vi "main_scan_3.vi"() -> ()   [LabVIEW 2009]
uses:
  <vilib>/userDefined/High Color/IMAQdx.ctl
  <vilib>/vision/Image Controls.llb/IMAQ Image.ctl
  global_stage_initialised.vi
  <vilib>/vision/driver/IMAQdx.llb/IMAQdx Buffer Number Mode.ctl
  <vilib>/Utility/file.llb/Write To Spreadsheet File (DBL).vi
  <vilib>/vision/driver/NI_Vision_Acquisition_Software.lvlib
  C:/Program Files/National Instruments/LabVIEW 2009/resource/objmgr/imaqdx.rc
panel:
  out "Vektor Summierte Helligkeit [a.u.]":dbl[](array[numeric])
  out "Vektor L/2-Position [°]":dbl[](array[numeric])
  out "Daten speichern":bool
  out "Leist/Pol # Schleifen":i64
  out "Leistungs-/Polarisationscan läuft":bool
  in  "Max. Spannungsdifferenz":dbl=150.0
  out "Geschätzte Messzeit":string="00:00"
  out "Start time [ms]":timestamp
  out "2D-Intensitätsverteilung (MCP)":dbl[][](graph)
  in  "# Photosignale":i32
  in  "Achs-ID":i32
  in  "Spannungskanal":refnum<k21>
  out "x-U-Scan läuft":bool
  out "Spannungsscan läuft":bool
  out "LAPD Spannung (V)":dbl format="%#.3g"
  out "Summierte Helligkeit (a.u.)":u64
  out "# Messschritte":i32
  out "Aktueller Messschritt":i32
  in  "LAPD-Daten speichern":bool
  in  "Summierte Helligkeit speichern":bool
  in  "Einzelbilder speichern":bool
  in  "Gemittelte Bilder speichern":bool
  in  "# Bilder/Messschritt":i32=1
  in  "SN von Rotationsbühne":i32=83831982
  in  "Wellenplatte [°]":refnum<k7>(container)
  out "Wellenplatte":bool
  in  "Waveplate ON/OFF":bool
  in  "Registerkarte":T1(tab)=enum."Leistungs-/Polarisationsscan"
  out "Aktuelle xyz-Position [mm]":dbl[](array[numeric]) format="%.5g"
  in  "Rasterweite [µm]":dbl[](array[numeric])
  in  "# Rasterschritte":i32[](array[numeric])=[1, 1, 1] min=1 step=1
  in  "Rasterung ON/OFF":bool
  out "Start xyz-Position [mm]":dbl[](array[numeric]) format="%.5g"
  in  "Rasterart":T2(ring)=enum."2D-Scan(xy)"
  out "Rasterschritt [µm]":dbl[](array[numeric])
  out "2D-Intensitätsverteilung (LAPD)":dbl[][](graph)
  out "Spannungsstart [V]":dbl[](array[numeric])
  out "TIP/SUP":string[](array[string])=["Tip", "Suppressor"]
  out "Spannungsschritt [V]":dbl[](array[numeric]) format="%.1g"
  out "Aktuelle Spannung [V]":dbl[](array[numeric]) format="%.1f"
  in  "# Spannungsschritte":i32[](array[numeric])
  in  "Spannungsweite [V]":dbl[](array[numeric])
  in  "Spannungsscan ON/OFF":bool
  out "Schräglage berücksichtigen":string="Schräglage berücksichtigen"
  in  "Ausgleichslage Start festlegen":bool
  out "x-U-Scan (Ausgleichslage) xy-Start [mm]":dbl[](array[numeric]) format="%_5g"
  in  "Raum-Koordinate 2 (Lagenausgleich)":enum16{"x-Achse", "y-Achse", "z-Achse"}(ring)=enum."y-Achse"
  out "x-U-Scan y-Startposition [mm]":dbl format="%.4g"
  out "x-U-Scan aktuelle y-Position [mm]":dbl format="%.4g"
  in  "x-U-Scan (Ausgleichslage) Steigung":dbl format="%_3g"
  out "x-U-Scan Spannungsstart [V]":dbl
  out "x-U-Scan Spannungsschritt [V]":dbl
  out "x-U-Scan aktuelle Spannung [V]":dbl
  in  "# x-U-Scan Spannungsschritte":i32
  in  "x-U-Scan Spannungsweite [V]":dbl
  in  "Raum-Koordinate 1":enum16{"x-Achse", "y-Achse", "z-Achse"}(ring)
  in  "Spannungs-Koordinate":enum16{"Tip-Spannung", "Suppressor-Spannung"}(ring)=2
  in  "x-U-Scan ON/OFF":bool
  in  "x-U-Scan x-Rasterweite [µm]":dbl
  in  "# x-U-Scan x-Rasterschritte":i32
  out "x-U-Scan x-Startposition [mm]":dbl format="%.4g"
  out "x-U-Scan aktuelle x-Position [mm]":dbl format="%.4g"
  out "x-U-Scan x-Rasterschritt [µm]":dbl
  out "x-U-Scan (Ausgleichslage) xy-End [mm]":dbl[](array[numeric]) format="%_5g"
  in  "Ausgleichslage Ende festlegen":bool
  in  "Max. Leistung (vK) [mW]":dbl
  out "Aktuelle Leistung (iK) [mW]":dbl
  out "Aktuelle L/2-Position [°]":dbl format="%_3g"
  out "L/2-Schritt [°]":dbl
  in  "Hin und Zurück":bool=TRUE
  in  "# L/2-Schritte":i32
  in  "L/2-Weite [°]":dbl
  in  "L/2-Start [°]":dbl
  in  "Leistuns- oder Polarisationsscan":u16(ring) items=["Polarisationsscan", "Leistungsscan"]
  in  "Leistungs-/Polarisationsscan ON/OFF":bool
  out "1D-Intensitätsverteilung (MCP)":T3(graph)
  in  "Sequenz Ordner":string="Referenzbilder"
  in  "Sequenzaufnahme ON":bool
  in  "MCP-Spannung [V]":dbl=1400.0
  in  "P-Schirm-Spannung [V]":dbl=4400.0
  in  "Proben-ID":string="140528_06"
  out "Messlogbuch":path
  out "Gemitteltes Bild":u64[][](array[numeric])
  in  "Polarisation [°]":dbl=90.0
  out "Current y step":i32
  out "Current z step":i32
  out "Current x step":i32
  out "Scanschleifenzähler":i32
  out "Kameraschleifenzähler":i32
  out "Steuerschleifenzähler":i32
  out "Bühne":bool
  in  "HV ON/OFF":bool
  out "HV-Steuerung":bool
  in  "Suppressor-Spannung [V]":dbl min=0.0 max=1000.0 step=1.0 format="%.1p"
  in  "Tip-Spannung [V]":dbl min=0.0 max=800.0 step=1.0 format="%.1p"
  in  "Leistung (iK) [mW]":dbl format="%.1f"
  in  "LAPD-Kanal (Meilhaus)":u32=1 max=31
  out "Save folder":string
  out "Buffer Number":u64
  out "ROI table":string[](array[string])=["Breite [px]", "Höhe [px]", "X-Offset [px]", "Y-Offset [px]"]
  in  "Vollbild":bool
  out "Frame Rate (FPS)":dbl format="%#_3g"
  in  "Buffer Interval":u32=1
  out "Ereignis: FrameDone?":refnum<event-registration>
  out "Image Display":T4(plugin-control)
  in  "ROI":i32[](array[numeric])=[640, 480, 0, 0]
  in  "Shutter time (ms)":u16(ring)=3 items=["1000", "500", "200", "100", "50", "20", "10"]
  out "Buffer Overrun":bool
  out "Image Memory":T4
  out "Kamera":bool
  in  "Kamera ON/OFF":bool
  in  "Detektionskamera":T5="cam0"
  out "Day folder":string
  in  "Root folder":string="E:\\GIPES\\Messungen\\"
  out "z-Achse":i32=3
  out "y-Achse":i32=2
  out "x-Achse":i32=1
  out "Event: Rasterung gestartet?":refnum<user-event>
  out "Fehler (Ausgang)":errorcluster
  in  "Programm beenden":bool
  out "Rasterung läuft":bool
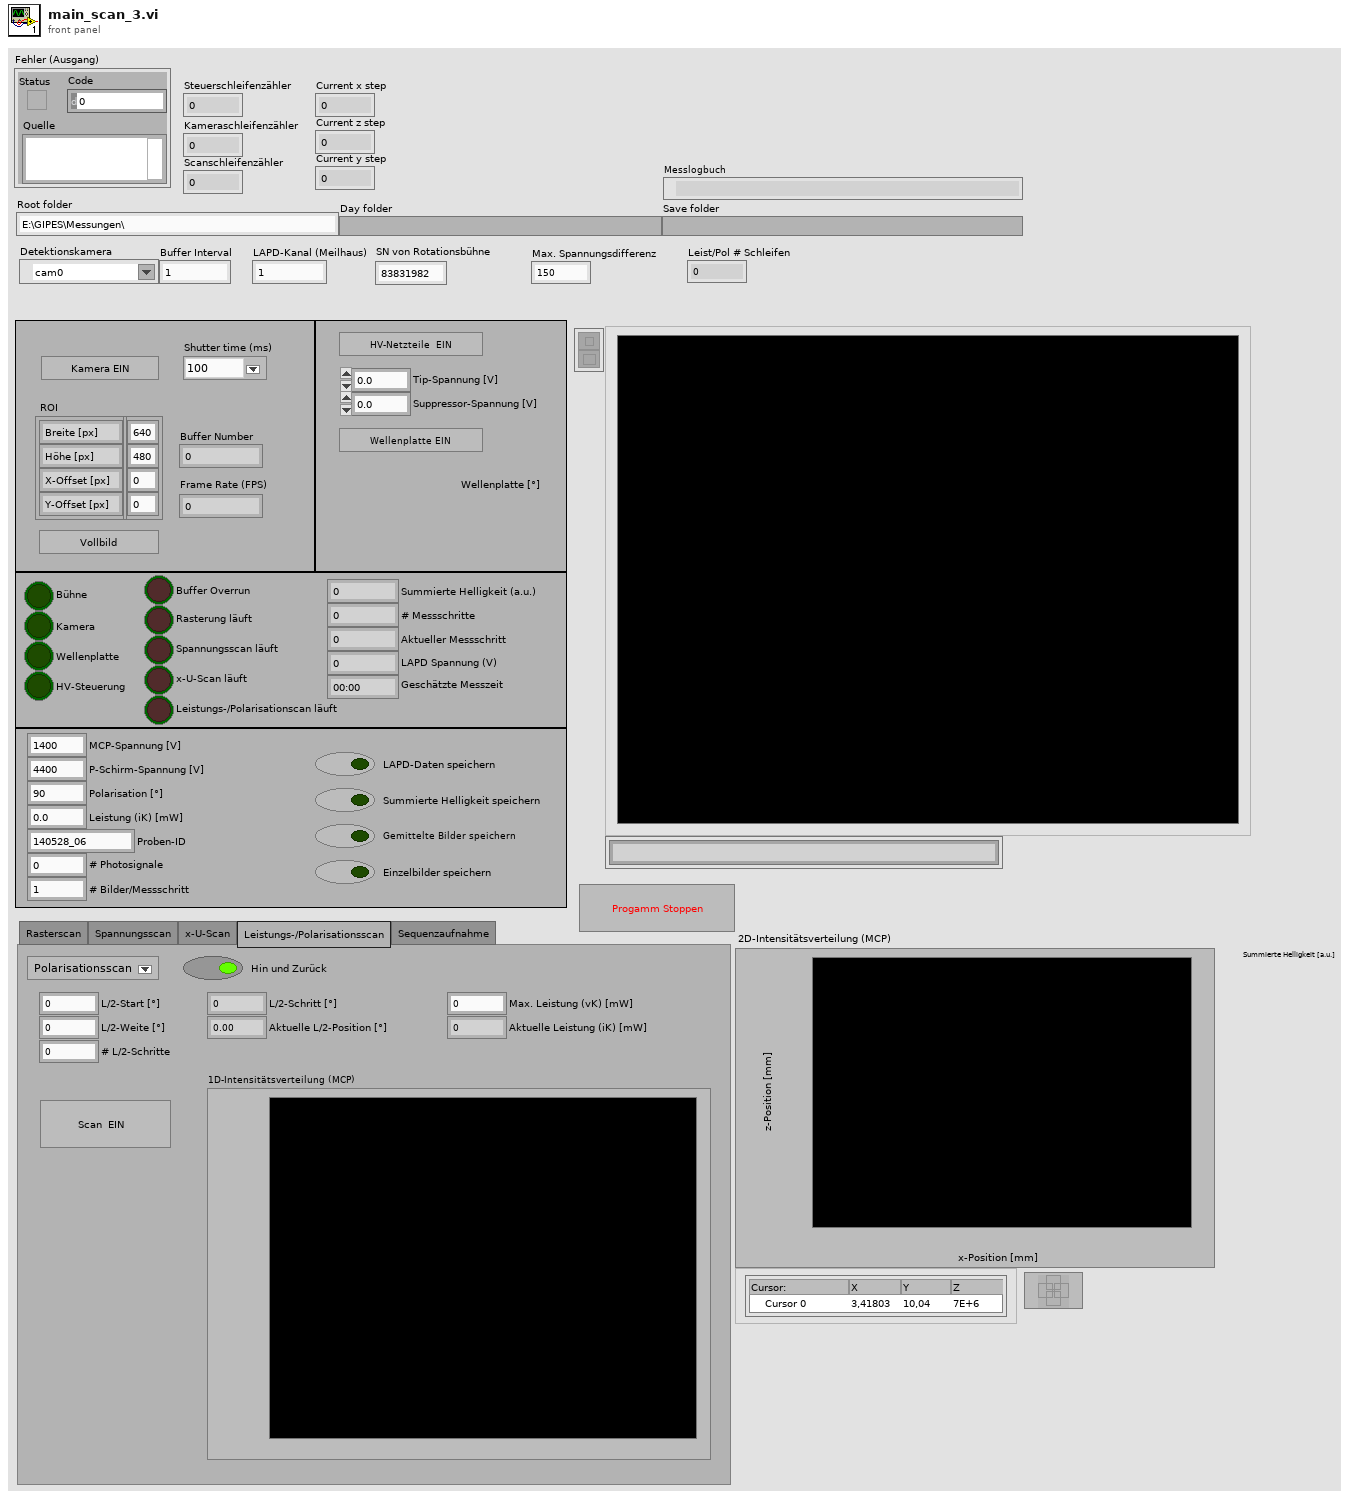
[diagram p1: front panel]
types:
  T1 = enum32{"Rasterscan", "Spannungsscan", "x-U-Scan", "Leistungs-/Polarisationsscan", "Sequenzaufnahme"}
  T2 = enum16{"Linescan(x)", "Linescan(z)", "2D-Scan(xy)", "2D-Scan(yz)", "2D-Scan(xz)"}
  T3 = cluster{"Vektor L/2-Position [°]":dbl[], "Vektor Summierte Helligkeit [a.u.]":dbl[]}
  T4 = typedef "IMAQ Image.ctl" = refnum<image>
  T5 = typedef "IMAQdx.ctl" = refnum<k21>
  T6 = enum32{"Bad", "Idle", "Run top level", "Running"}
  T7 = cluster{"Summierte Helligkeit (a.u.)":u64, "Aktuelle L/2-Position [°]":dbl}
  T8 = typedef "NI_Vision_Acquisition_Software.lvlib/IMAQdx Buffer Number Mode.ctl" = enum32{"Next", "Last", "Buffer Number"}
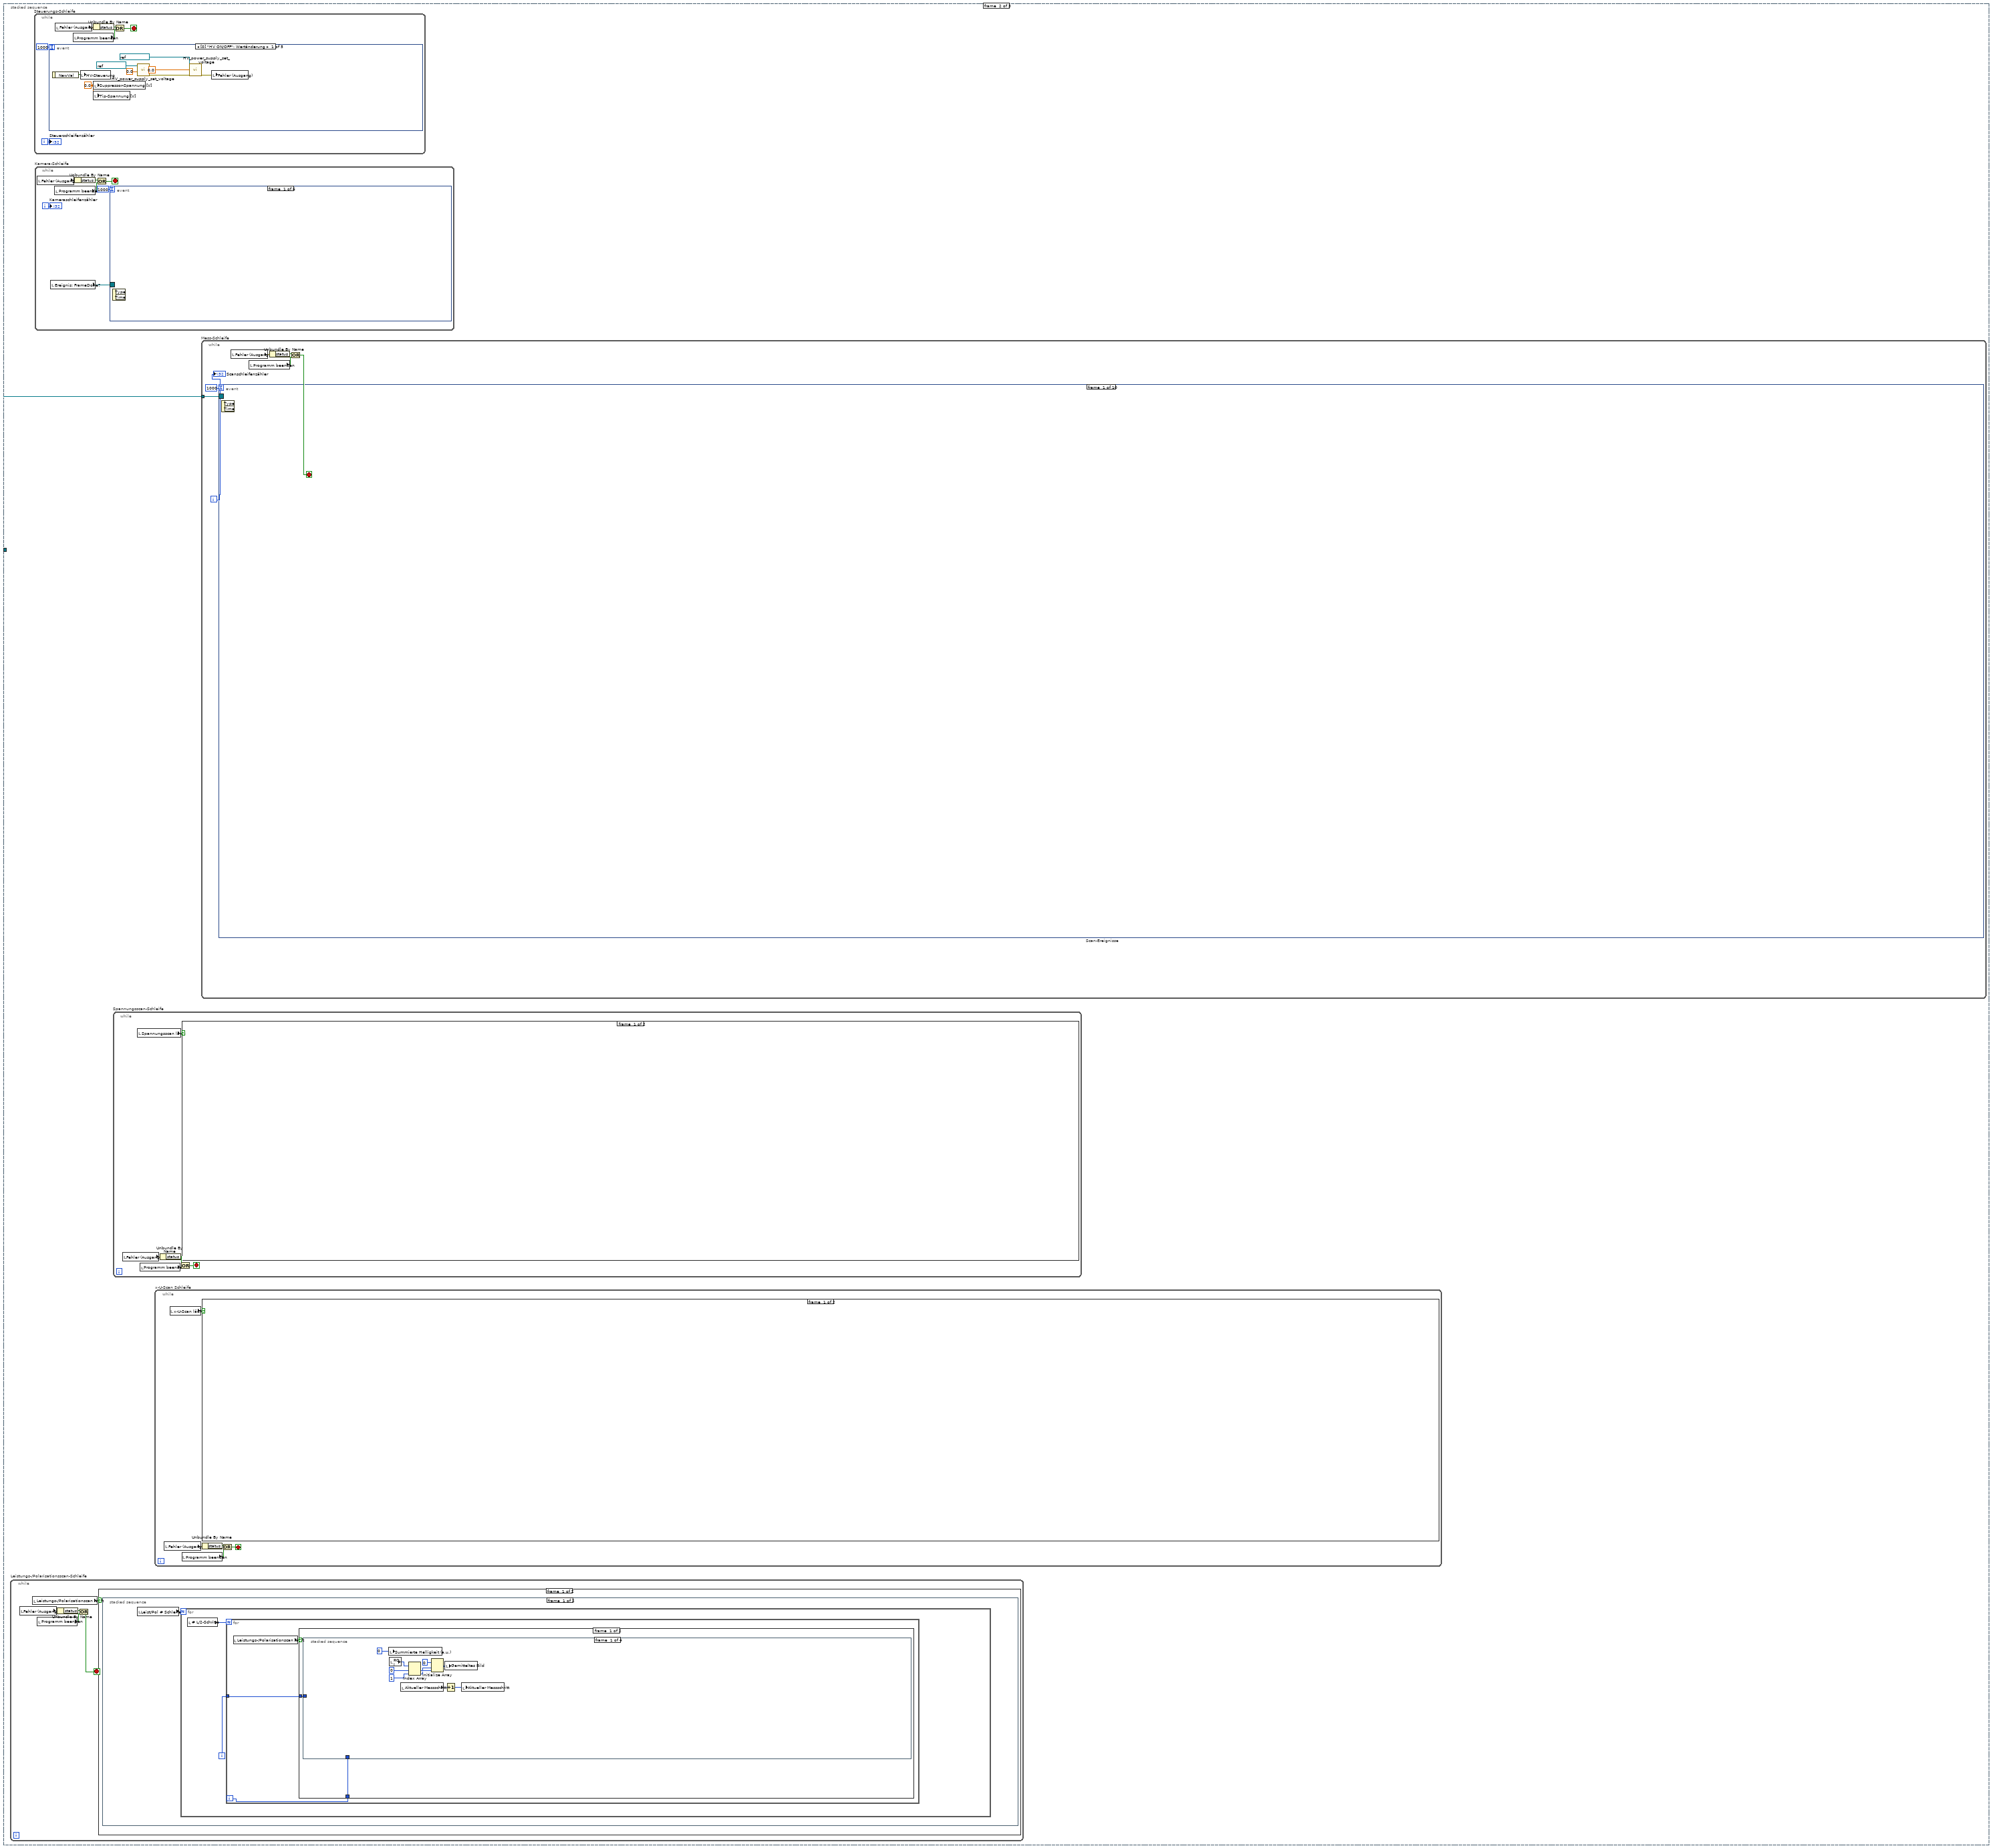
[diagram p3: hidden frame]
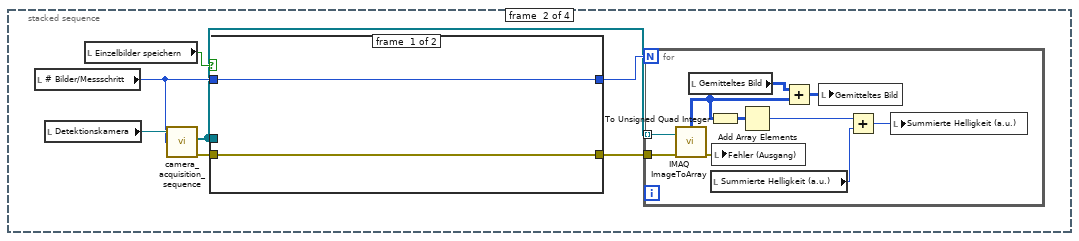
[diagram p4: hidden frame]
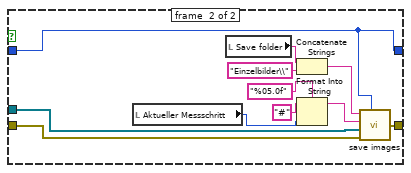
[diagram p5: hidden frame]
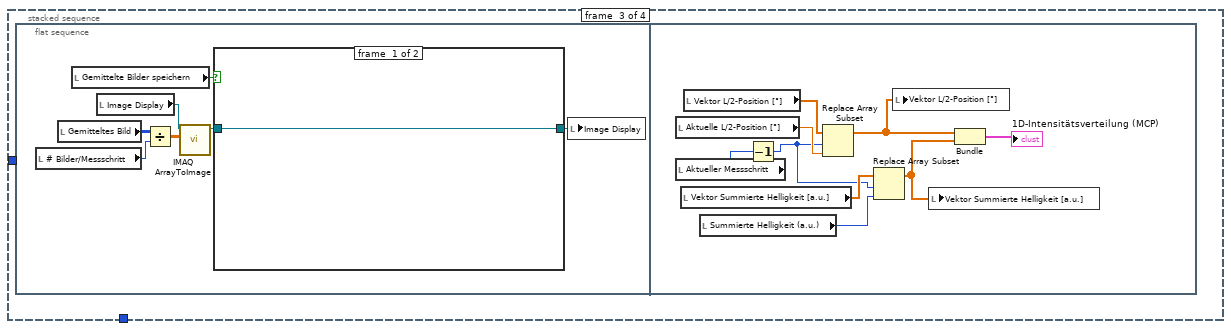
[diagram p6: hidden frame]
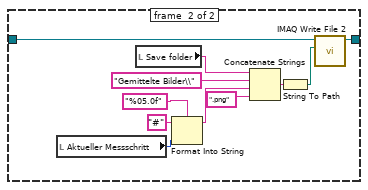
[diagram p7: hidden frame]
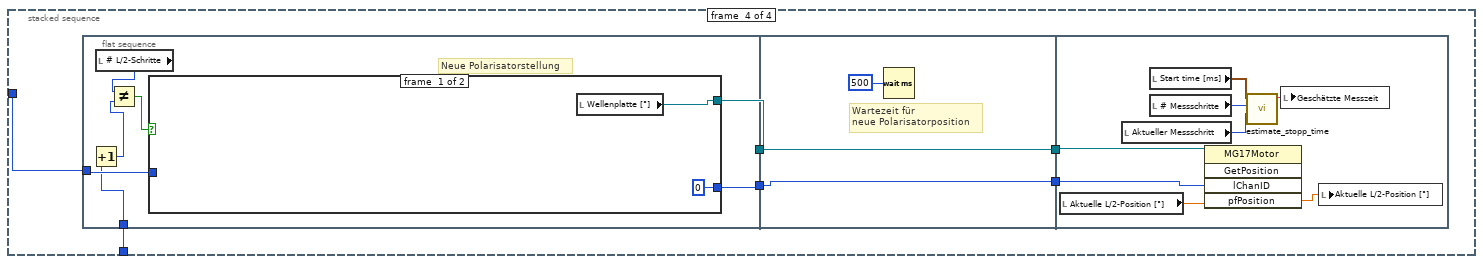
[diagram p8: hidden frame]
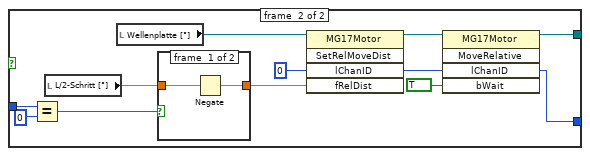
[diagram p9: hidden frame]
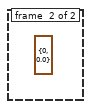
[diagram p11: hidden frame]
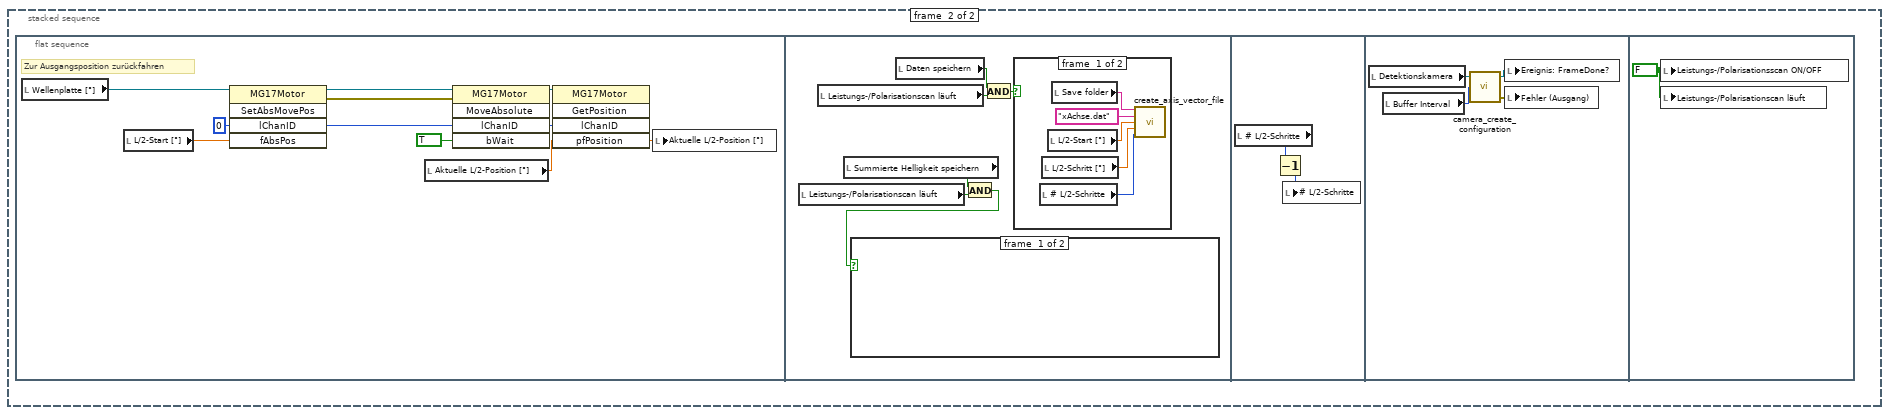
[diagram p12: hidden frame]
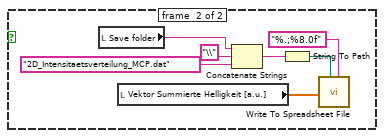
[diagram p13: hidden frame]
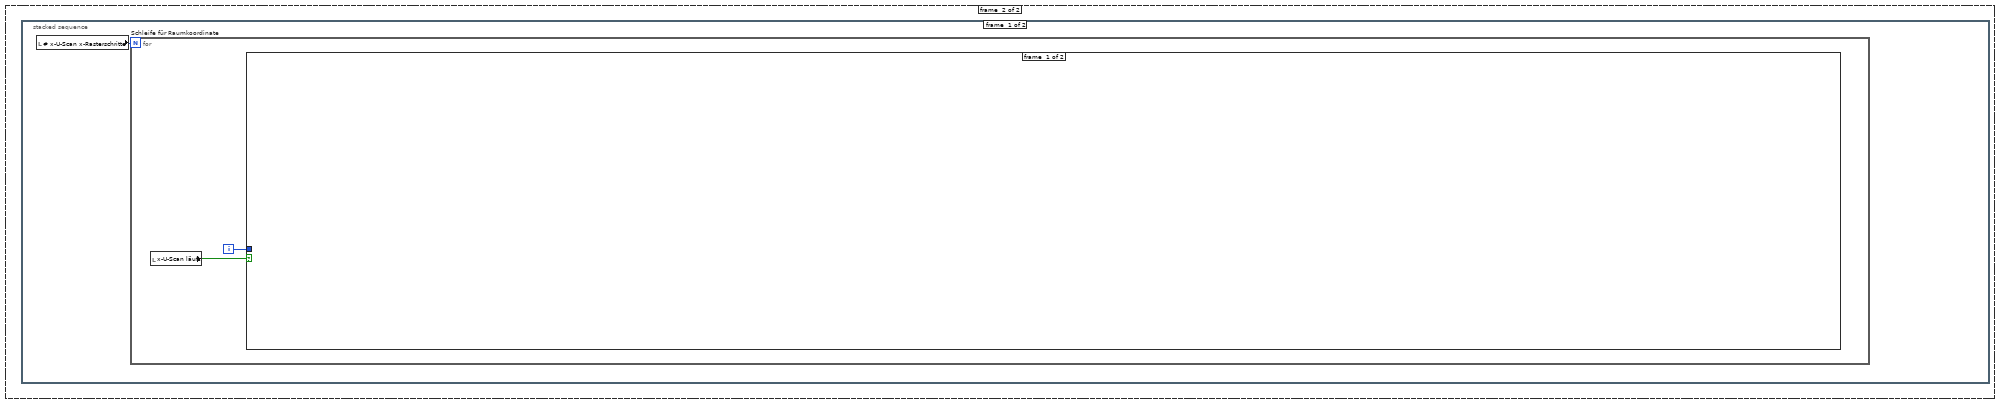
[diagram p16: hidden frame]
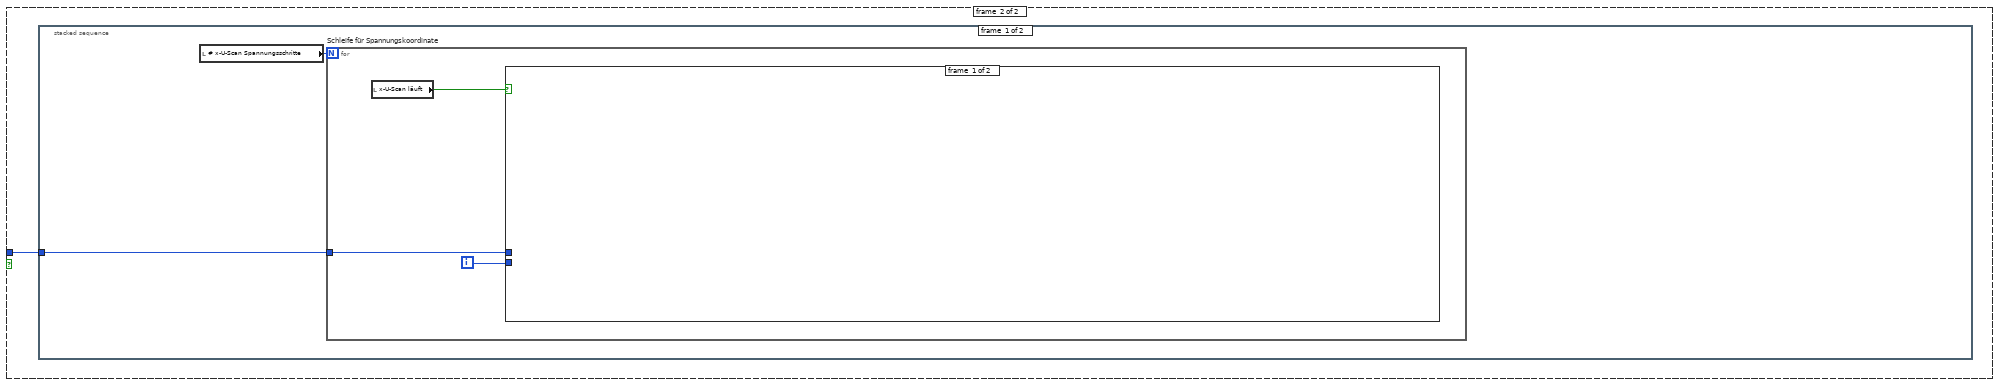
[diagram p17: hidden frame]
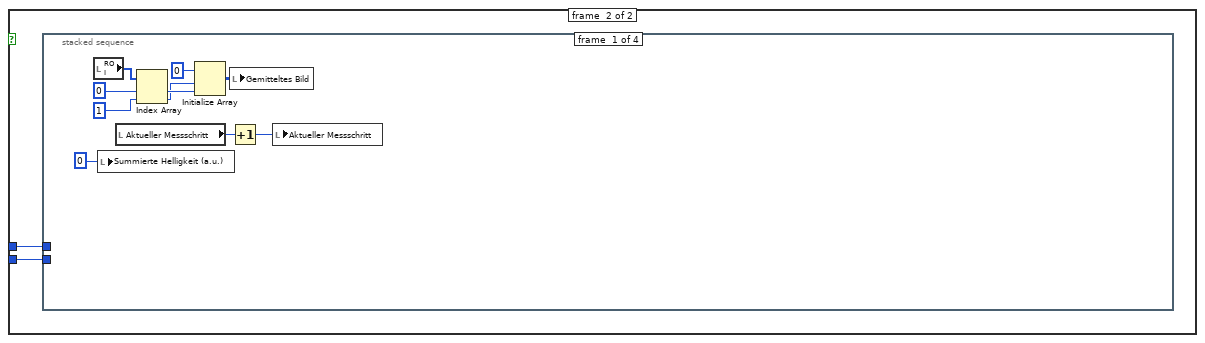
[diagram p18: hidden frame]
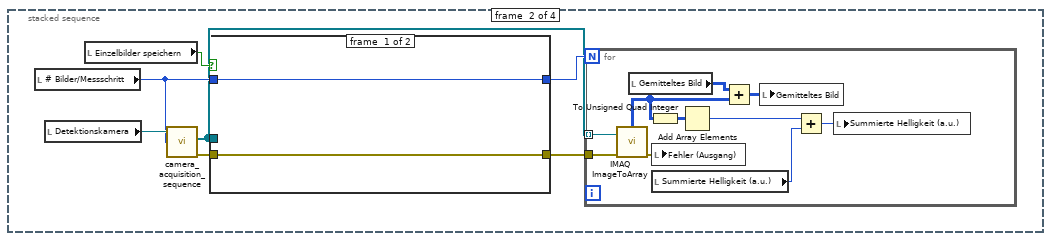
[diagram p19: hidden frame]
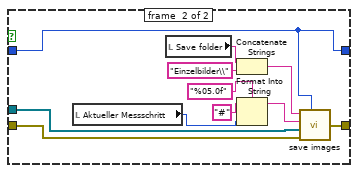
[diagram p20: hidden frame]
diagram:
  n1 = local read "Event: Rasterung gestartet?"() -> (w2:refnum<user-event>)
  n2 = register-events(w2) -> (reference out=w1:refnum<event-registration>)  [unwired: 2 in, 1 out]
  n3 = flat-sequence {
    frame #0 {
      w5 = 0.0 ("Aktuelle x-Position [mm]")
      w11 = 1 ("# x-U-Scan Spannungsschritte")
      w12 = 0.0 ("Aktuelle x-Position [mm]")
      w10 = 0.0 ("Suppressor-Spannung [V]")
      w25 = u16 3 items=["1000", "500", "200", "100", "50", "20", "10"] ("Shutter time (ms)")
      w3 = FALSE ("Scanstart")
      n4 = Initialize Array(1 ("Element"), 2 ("Dimension")) -> (w13:i32[])
      n5 = Initialize Array(1 ("Dimension"), 3 ("Dimension")) -> (w37:i32[])
      n6 = Initialize Array(0.0 ("Element"), 2 ("Dimension")) -> (w9:dbl[])
      "Aktuelle Spannung [V]" <- w9
      "Spannungsstart [V]" <- w9
      "x-U-Scan (Ausgleichslage) xy-Start [mm]" <- w9
      "x-U-Scan (Ausgleichslage) xy-End [mm]" <- w9
      n7 = Initialize Array(0.0 ("Element"), 3 ("Dimension")) -> (w19:dbl[])
      "Aktuelle xyz-Position [mm]" <- w19
      "Start xyz-Position [mm]" <- w19
      "Rasterschritt [µm]" <- w19
      n8 = local write "Tip-Spannung [V]"(0.0 ("Tip-Spannung [V]")) -> ()
      n9 = local write "# Photosignale"(10.0 ("Anzahl Mittelungen")) -> ()
      n10 = local write "# x-U-Scan x-Rasterschritte"(w11) -> ()
      n11 = local write "x-U-Scan x-Rasterweite [µm]"(w10) -> ()
      n12 = local write "Shutter time (ms)"(w25) -> ()
      n13 = local write "# Spannungsschritte"(w13) -> ()
      n14 = local write "ROI"(i32[] [640, 480, 0, 0] ("Region of Interest (px)")) -> ()
      n15 = local write "# x-U-Scan Spannungsschritte"(w11) -> ()
      n16 = local write "x-U-Scan Spannungsweite [V]"(w10) -> ()
      n17 = local write "Suppressor-Spannung [V]"(w10) -> ()
      n18 = local read "Aktueller Messschritt"() -> (w30:i32)
      n19 = local write "# Rasterschritte"(w37) -> ()
      n20 = local write "Spannungsweite [V]"(w9) -> ()
      n21 = local write "Rasterweite [µm]"(w19) -> ()
      n22 = local write "x-U-Scan (Ausgleichslage) Steigung"(0.0 ("x-U-Scan (Ausgleichslage) Steigung")) -> ()
      n23 = local write "HV ON/OFF"(w3) -> ()
      n24 = local write "Spannungsscan ON/OFF"(w3) -> ()
      n25 = local write "Buffer Overrun"(w3) -> ()
      n26 = local write "Programm beenden"(w3) -> ()
      n27 = local write "x-U-Scan ON/OFF"(w3) -> ()
      n28 = local write "x-U-Scan läuft"(w3) -> ()
      n29 = local write "Sequenzaufnahme ON"(w3) -> ()
      n30 = local write "Kamera ON/OFF"(w3) -> ()
      n31 = local write "Rasterung ON/OFF"(w3) -> ()
      n32 = local write "Rasterung läuft"(w3) -> ()
      n33 = local write "Spannungsscan ON/OFF"(w3) -> ()
      n34 = local write "Waveplate ON/OFF"(w3) -> ()
      n35 = Create User Event(user event datatype=w30) -> (user event=→"Event: Rasterung gestartet?":refnum<user-event>)  [unwired: 1 in, 1 out]
      n36 = local write "Leistungs-/Polarisationsscan ON/OFF"(w3) -> ()
      "Rasterung läuft" <- FALSE ("Scan aktiv")
      "# Messschritte" <- 0 ("# Messschritte")
      "Aktueller Messschritt" <- 0 ("Aktueller Messschritt")
      "x-Achse" <- 1 ("x-Achse")
      "y-Achse" <- 2 ("y-Achse")
      "z-Achse" <- 3 ("z-Achse")
      "Summierte Helligkeit (a.u.)" <- i64 0 ("Numerisches Element")
      "LAPD Spannung (V)" <- 0.0 ("Transmittierte Intensität (a.u.)")
      "Bühne" <- w3
      "Wellenplatte" <- w3
      "Kamera" <- FALSE ("Camera eingeschaltet")
      "HV-Steuerung" <- w3
      "Spannungsscan läuft" <- w3
      "x-U-Scan aktuelle x-Position [mm]" <- w12
      "x-U-Scan x-Rasterschritt [µm]" <- w12
      "x-U-Scan aktuelle Spannung [V]" <- w12
      "x-U-Scan Spannungsschritt [V]" <- w12
      "x-U-Scan x-Startposition [mm]" <- w12
      "x-U-Scan Spannungsstart [V]" <- w10
      "x-U-Scan aktuelle y-Position [mm]" <- 0.0 ("x-U-Scan aktuelle y-Position [mm]")
      "x-U-Scan y-Startposition [mm]" <- 0.0 ("x-U-Scan y-Startposition [mm]")
      "L/2-Schritt [°]" <- w5
      "Aktuelle L/2-Position [°]" <- w5
      "Aktuelle Leistung (iK) [mW]" <- w5
      "Leistungs-/Polarisationscan läuft" <- w3
      "Leist/Pol # Schleifen" <- i64 1 ("Leist/Pol # Schleifen")
      "Daten speichern" <- w3
    }
  }
  n37 = stacked-sequence {
    tunnel: w1 -> [_ w63 _]
    frame #0 {
      n38 = flat-sequence {
        frame #0 {
          # "Überprüfung ob die VI stage_control.vi ausgeführt wid, wenn nicht wird sie gestartet und gewartet bis die Bühne initialisiert ist"
          n39 = Open VI Reference(vi path=path "stage_control.vi" ("VI-Pfad")) -> (vi reference=w41:refnum<vi>)  [unwired: 5 in, 1 out]
          n40 = property class="VI"(reference=w41) -> (reference out=w40:refnum<vi>, error out=w39:errorcluster, "Exec.State"=w44:T6)  [unwired: 1 in]
          n41 = Equal?(x=w44, y=T6."Run top level") -> (x = y?=w42:bool)
          n42 = case shown="False" w42 {
            tunnel: w40 -> [w51 _]
            tunnel: w39 -> [w50 _]
            frame #0 {
              n43 = invoke class="VI" method="VI ausführen"(reference=w51, error in=w50, "Wait until done"=FALSE ("Warten bis beendet"), "Auto Dispose Ref"=FALSE ("Referenz automatisch schließen")) -> (reference out=w47:refnum<vi>)  [unwired: 1 in, 4 out]
              n44 = invoke class="VI" method="FP.Öffnen"(reference=w47) -> (reference out=w46:refnum<vi>)  [unwired: 4 in, 4 out]
              n45 = while {
                tunnel: w46 -> [w58]
                stop <- w53 stop-if-true
                n46 = property class="VI"(reference=w58) -> (error out=w57:errorcluster, "Exec.State"=w56:T6)  [unwired: 1 in, 1 out]
                n47 = global read "global_stage_initialised.vi" "Bühne initialisiert"() -> (w52:bool)
                n48 = local write "Fehler (Ausgang)"(w57) -> ()
                n49 = Equal?(x=w56, y=T6."Run top level") -> (x = y?=w54:bool)
                n50 = And(x=w52, y=w54) -> (x .and. y?=w53:bool)
              }
            }
            frame #1 {
            }
          }
        }
        frame #1 {
          n51 = local read "Root folder"() -> (w62:string)
          n52 = local write "Bühne"(TRUE ("Bühne bereit")) -> ()
          n53 = call "create_day_folder.vi"("Root folder"=w62) -> ("Day Folder"=w60:string)  [unwired: 9 in, 1 out]
          n54 = local write "Day folder"(w60) -> ()
          n55 = call "create_measure_log_file.vi"("Tagesordner"=w60) -> ("Messlogbuch"=w59:path)  [unwired: 9 in]
          n56 = local write "Messlogbuch"(w59) -> ()
        }
      }
    }
    frame #1 {
      n57 = while "Leistungs-/Polarisationsscan-Schleife" {
        stop <- w65 stop-if-true
        n58 = local read "Fehler (Ausgang)"() -> (w68:errorcluster)
        n59 = local read "Leistungs-/Polarisationscan läuft"() -> (w64:bool)
        n60 = local read "Programm beenden"() -> (w66:bool)
        n61 = Unbundle By Name(w68) -> ("status"=w67:bool)
        n62 = Or(x=w67, y=w66) -> (x .or. y?=w65:bool)
        n63 = case shown="True" w64 {
          frame #0 {
            n64 = stacked-sequence {
              frame #0 {
                n65 = local read "Leist/Pol # Schleifen"() -> (w69:i64)
                n66 = for {
                  N: w69 -> [_]
                  i -> [w70]
                  n67 = local read "# L/2-Schritte"() -> (w71:i32)
                  n68 = for "Schleife für L/2-Position" {
                    N: w71 -> [_]
                    tunnel: w70 -> [w73]
                    i -> [w72]
                    n69 = local read "Leistungs-/Polarisationscan läuft"() -> (w74:bool)
                    n70 = case shown="True" w74 {
                      tunnel: w73 -> [w76 _]
                      tunnel: w72 -> [w75 _]
                      frame #0 {
                        n71 = stacked-sequence {
                          tunnel: w76 -> [_ _ _ w150]
                          tunnel: w75 -> [_ _ _ w145]
                          frame #0 {
                            n72 = local write "Summierte Helligkeit (a.u.)"(u64 0 ("Summierte Helligkeit (a.u.)")) -> ()
                            n73 = local read "ROI"() -> (w82:i32[])
                            n74 = local read "Aktueller Messschritt"() -> (w79:i32)
                            n75 = Index Array(array=w82, index #1=0 ("Index"), index #2=1 ("Index")) -> (element #1=w86:i32, element #2=w85:i32)
                            n76 = Initialize Array(u64 0 ("Element"), w85, w86) -> (w80:u64[][])
                            n77 = local write "Gemitteltes Bild"(w80) -> ()
                            n78 = Increment(x=w79) -> (x+1=w78:i32)
                            n79 = local write "Aktueller Messschritt"(w78) -> ()
                          }
                          frame #1 {
                            n80 = local read "# Bilder/Messschritt"() -> (w90:i32)
                            n81 = local read "Detektionskamera"() -> (w93:T5)
                            n82 = local read "Einzelbilder speichern"() -> (w88:bool)
                            n83 = call "camera_acquisition_sequence.vi"("Session In"=w93, "Desired image number"=w90) -> ("Image Array"=w87:T4[], "error out"=w92:errorcluster)  [unwired: 2 in, 1 out]
                            n84 = case shown="True" w88 {
                              tunnel: w92 -> [w95 w103]
                              tunnel: [w95 w102] -> w91
                              tunnel: w90 -> [w94 w101]
                              tunnel: [w94 w101] -> w89
                              tunnel: w87 -> [_ w100]
                              frame #0 {
                              }
                              frame #1 {
                                n85 = local read "Aktueller Messschritt"() -> (w106:i32)
                                n86 = local read "Save folder"() -> (w98:string)
                                n87 = Concatenate Strings(w98, "Einzelbilder\\" ("String")) -> (w96:string)
                                n88 = Format Into String(format string="%05.0f" ("Format-String"), initial string="#" ("Eingangs-String"), w106) -> (resulting string=w99:string)  [unwired: 1 in, 1 out]
                                n89 = call "save images.vi"("Save Folder"=w96, "File name prefix"=w99, "Array"=w100, "error out 2"=w103, "Bilder/Messschritt"=w101) -> ("error out"=w102:errorcluster)
                              }
                            }
                            n90 = for {
                              N: w89 -> [_]
                              tunnel: w91 -> [w112]
                              tunnel: w87 -> [w110] mode=indexing
                              n91 = call "IMAQ ImageToArray"("error in (no error)"=w112, "Image"=w110) -> ("error out"=w111:errorcluster, "Image Pixels (U8)"=w109:u8[][])  [unwired: 2 in, 3 out]
                              n92 = local read "Gemitteltes Bild"() -> (w107:u64[][])
                              n93 = To Unsigned Quad Integer(1:w109) -> (0:w114:u64[][])
                              n94 = local read "Summierte Helligkeit (a.u.)"() -> (w115:u64)
                              n95 = local write "Fehler (Ausgang)"(w111) -> ()
                              n96 = Add Array Elements(numeric array=w114) -> (sum=w113:u64)
                              n97 = Add(x=w107, y=w109) -> (x+y=w108:u64[][])
                              n98 = local write "Gemitteltes Bild"(w108) -> ()
                              n99 = Add(x=w113, y=w115) -> (x+y=w116:u64)
                              n100 = local write "Summierte Helligkeit (a.u.)"(w116) -> ()
                            }
                          }
                          frame #2 {
                            n101 = flat-sequence {
                              frame #0 {
                                n102 = local read "# Bilder/Messschritt"() -> (w119:i32)
                                n103 = local read "Gemitteltes Bild"() -> (w117:u64[][])
                                n104 = local read "Gemittelte Bilder speichern"() -> (w123:bool)
                                n105 = local read "Image Display"() -> (w121:T4)
                                n106 = Divide(x=w117, y=w119) -> (x/y=w118:dbl[][])
                                n107 = call "IMAQ ArrayToImage"("Image Pixels (U8)"=w118, "Image"=w121) -> ("Image Out"=w120:T4)  [unwired: 8 in, 1 out]
                                n108 = case shown="True" w123 {
                                tunnel: w120 -> [w124 w135]
                                tunnel: [w124 w126] -> w122
                                frame #0 {
                                }
                                frame #1 {
                                n109 = local read "Aktueller Messschritt"() -> (w130:i32)
                                n110 = local read "Save folder"() -> (w132:string)
                                n111 = Format Into String(format string="%05.0f" ("Format-String"), initial string="#" ("Eingangs-String"), w130) -> (resulting string=w129:string)  [unwired: 1 in, 1 out]
                                n112 = Concatenate Strings(w132, "Gemittelte Bilder\\" ("String"), w129, ".png" ("String")) -> (w128:string)
                                n113 = String To Path(string=w128) -> (path=w127:path)
                                n114 = call-poly "IMAQ Write File 2"("File Path"=w127, "Image"=w135) -> ("Image Out (duplicate)"=w126:T4)  [unwired: 8 in, 1 out]
                                }
                                }
                                n115 = local write "Image Display"(w122) -> ()
                              }
                              frame #1 {
                                n116 = local read "Aktuelle L/2-Position [°]"() -> (w141:dbl)
                                n117 = local read "Aktueller Messschritt"() -> (w139:i32)
                                n118 = local read "Vektor Summierte Helligkeit [a.u.]"() -> (w143:dbl[])
                                n119 = local read "Vektor L/2-Position [°]"() -> (w142:dbl[])
                                n120 = local read "Summierte Helligkeit (a.u.)"() -> (w140:u64)
                                n121 = Decrement(x=w139) -> (x-1=w138:i32)
                                n122 = Replace Array Subset(array=w142, new element=w141, index=w138) -> (w137:dbl[])
                                n123 = Replace Array Subset(array=w143, new element=w140, index=w138) -> (w136:dbl[])
                                n124 = local write "Vektor L/2-Position [°]"(w137) -> ()
                                n125 = local write "Vektor Summierte Helligkeit [a.u.]"(w136) -> ()
                                n126 = Bundle("Vektor L/2-Position [°]"=w137, "Vektor Summierte Helligkeit [a.u.]"=w136) -> (→"1D-Intensitätsverteilung (MCP)":T3)  [unwired: 1 in]
                              }
                            }
                          }
                          frame #3 {
                            n127 = flat-sequence {
                              tunnel: w150 -> [w157]
                              tunnel: [w156] -> w149
                              tunnel: [w155] -> w148
                              tunnel: w145 -> [w154]
                              tunnel: w149 -> [w175]
                              tunnel: w148 -> [w176]
                              tunnel: [w176] -> w147
                              tunnel: [w175] -> w146
                              tunnel: w147 -> [w181]
                              tunnel: w146 -> [w180]
                              frame #0 {
                                # "Neue Polarisatorstellung"
                                n128 = Increment(x=w154) -> (x+1=w153:i32)
                                n129 = local read "# L/2-Schritte"() -> (w152:i32)
                                n130 = Not Equal?(x=w152, y=w153) -> (x != y?=w151:bool)
                                n131 = case shown="True" w151 {
                                tunnel: w157 -> [_ w164]
                                tunnel: [0 ("lChanID") w161] -> w156
                                tunnel: [w159 w160] -> w155
                                frame #0 {
                                n132 = local read "Wellenplatte [°]"() -> (w159:refnum<k7>)
                                }
                                frame #1 {
                                n133 = Equal?(x=w164, y=0) -> (x = y?=w162:bool)
                                n134 = local read "L/2-Schritt [°]"() -> (w166:dbl)
                                n135 = local read "Wellenplatte [°]"() -> (w167:refnum<k7>)
                                n136 = case shown="False" w162 {
                                tunnel: w166 -> [w173 w174]
                                tunnel: [w172 w174] -> w165
                                frame #0 {
                                n137 = Negate(x=w173) -> (-x=w172:dbl)
                                }
                                frame #1 {
                                }
                                }
                                n138 = invoke class="MG17Motor" method="SetRelMoveDist"(reference=w167, "lChanID"=0, "fRelDist"=w165) -> (reference out=w169:refnum<k7>, "lChanID"=w170:i32)  [unwired: 2 in, 3 out]
                                n139 = invoke class="MG17Motor" method="MoveRelative"(reference=w169, "lChanID"=w170, "bWait"=TRUE) -> (reference out=w160:refnum<k7>, "lChanID"=w161:i32)  [unwired: 2 in, 3 out]
                                }
                                }
                              }
                              frame #1 {
                                # "Wartezeit für\nneue Polarisatorposition"
                                n140 = Wait (ms)(milliseconds to wait=u32 500 ("Zu wartende ms")) -> ()  [unwired: 1 out]
                              }
                              frame #2 {
                                n141 = local read "Aktuelle L/2-Position [°]"() -> (w178:dbl)
                                n142 = local read "Aktueller Messschritt"() -> (w183:i32)
                                n143 = local read "Start time [ms]"() -> (w185:timestamp)
                                n144 = local read "# Messschritte"() -> (w184:i32)
                                n145 = invoke class="MG17Motor" method="GetPosition"(reference=w181, "lChanID"=w180, "pfPosition"=w178) -> ("pfPosition"=w179:sgl)  [unwired: 2 in, 4 out]
                                n146 = call "estimate_stopp_time.vi"("Aktueller Messschritt"=w183, "# Messschritte"=w184, "Startzeit"=w185) -> ("Stopp Zeit"=w182:string)  [unwired: 8 in]
                                n147 = local write "Geschätzte Messzeit"(w182) -> ()
                                n148 = local write "Aktuelle L/2-Position [°]"(w179) -> ()
                              }
                            }
                          }
                        }
                      }
                      frame #1 {
                        (unwired) T7 {"Summierte Helligkeit (a.u.)"=0, "Aktuelle L/2-Position [°]"=0.0}
                      }
                    }
                  }
                }
              }
              frame #1 {
                n149 = flat-sequence {
                  frame #0 {
                    # "Zur Ausgangsposition zurückfahren"
                    n150 = local read "Wellenplatte [°]"() -> (w196:refnum<k7>)
                    n151 = local read "L/2-Start [°]"() -> (w190:dbl)
                    n152 = invoke class="MG17Motor" method="SetAbsMovePos"(reference=w196, "lChanID"=0, "fAbsPos"=w190) -> (reference out=w194:refnum<k7>, error out=w191:errorcluster, "lChanID"=w192:i32)  [unwired: 2 in, 2 out]
                    n153 = local read "Aktuelle L/2-Position [°]"() -> (w188:dbl)
                    n154 = invoke class="MG17Motor" method="MoveAbsolute"(reference=w194, error in=w191, "lChanID"=w192, "bWait"=TRUE) -> (reference out=w187:refnum<k7>, "lChanID"=w186:i32)  [unwired: 1 in, 3 out]
                    n155 = invoke class="MG17Motor" method="GetPosition"(reference=w187, "lChanID"=w186, "pfPosition"=w188) -> ("pfPosition"=w189:sgl)  [unwired: 2 in, 4 out]
                    n156 = local write "Aktuelle L/2-Position [°]"(w189) -> ()
                  }
                  frame #1 {
                    n157 = local read "Leistungs-/Polarisationscan läuft"() -> (w199:bool)
                    n158 = local read "Leistungs-/Polarisationscan läuft"() -> (w201:bool)
                    n159 = local read "Summierte Helligkeit speichern"() -> (w198:bool)
                    n160 = local read "Daten speichern"() -> (w202:bool)
                    n161 = And(x=w198, y=w199) -> (x .and. y?=w197:bool)
                    n162 = case shown="True" w197 {
                      frame #0 {
                      }
                      frame #1 {
                        n163 = local read "Save folder"() -> (w203:string)
                        n164 = local read "Vektor Summierte Helligkeit [a.u.]"() -> (w204:dbl[])
                        n165 = Concatenate Strings(w203, "\\" ("String"), "2D_Intensitaetsverteilung_MCP.dat" ("String")) -> (w208:string)
                        n166 = String To Path(string=w208) -> (path=w207:path)
                        n167 = call-poly <vilib>:"Write To Spreadsheet File.vi"("format (%.3f)"="%.;%8.0f", "1D data"=w204, "file path (dialog if empty)"=w207) -> ()  [unwired: 5 in, 1 out]
                      }
                    }
                    n168 = And(x=w202, y=w201) -> (x .and. y?=w200:bool)
                    n169 = case shown="True" w200 {
                      frame #0 {
                        n170 = local read "# L/2-Schritte"() -> (w212:i32)
                        n171 = local read "L/2-Schritt [°]"() -> (w211:dbl)
                        n172 = local read "L/2-Start [°]"() -> (w210:dbl)
                        n173 = local read "Save folder"() -> (w213:string)
                        n174 = call "create_axis_vector_file.vi"("Save folder"=w213, "Dateiname"="xAchse.dat", "Start"=w210, "Schrittlänge"=w211, "# Schritte"=w212) -> ()  [unwired: 11 in]
                      }
                      frame #1 {
                      }
                    }
                  }
                  frame #2 {
                    n175 = local read "# L/2-Schritte"() -> (w216:i32)
                    n176 = Decrement(x=w216) -> (x-1=w215:i32)
                    n177 = local write "# L/2-Schritte"(w215) -> ()
                  }
                  frame #3 {
                    n178 = local read "Detektionskamera"() -> (w218:T5)
                    n179 = local read "Buffer Interval"() -> (w219:u32)
                    n180 = call "camera_create_configuration.vi"("BufferInterval"=w219, "Session Out 2"=w218) -> ("Fehler (Ausgang)"=w220:errorcluster, "Ereignisregistrierung (Referenz)"=w217:refnum<event-registration>)  [unwired: 1 in, 1 out]
                    n181 = local write "Ereignis: FrameDone?"(w217) -> ()
                    n182 = local write "Fehler (Ausgang)"(w220) -> ()
                  }
                  frame #4 {
                    w221 = FALSE ("Spannungsscan läuft")
                    n183 = local write "Leistungs-/Polarisationsscan ON/OFF"(w221) -> ()
                    n184 = local write "Leistungs-/Polarisationscan läuft"(w221) -> ()
                  }
                }
              }
            }
          }
          frame #1 {
          }
        }
      }
      n185 = while "Steuerungs-Schleife" {
        i -> [w578]
        stop <- w577 stop-if-true
        n186 = event shown="[0] \"HV ON/OFF\": Wertänderung" {
          selector: _ -> [_ _ _ _ _]
          dyn-events: _ -> [_ _ _ _ _]
          timeout: 1000 -> [_ _ _ _ _]
          event #0 {
            w583 = 0.0 ("Suppressor-Spannung [V]")
            n187 = event-data() -> ("NewVal"=w584:bool)  [unwired: 1 in]
            n188 = local write "HV-Steuerung"(w584) -> ()
            n189 = local write "Suppressor-Spannung [V]"(w583) -> ()
            n190 = local write "Tip-Spannung [V]"(w583) -> ()
            n191 = call "HV_power_supply_set_voltage.vi"("Desired output voltage in V (HV power supply)"=0.0, "Channel of HV power supply"=refnum<k21> "Dev0/Ao0") -> ("error out"=w586:errorcluster)  [unwired: 8 in]
            n192 = call "HV_power_supply_set_voltage.vi"("error in"=w586, "Desired output voltage in V (HV power supply)"=0.0, "Channel of HV power supply"=refnum<k21> "Dev0/Ao1") -> ("error out"=w585:errorcluster)  [unwired: 7 in]
            n193 = local write "Fehler (Ausgang)"(w585) -> ()
          }
          event #1 {
            n194 = event-data() -> ("NewVal"=w591:bool)  [unwired: 1 in]
            n195 = case shown="True" w591 {
              frame #0 {
                n196 = local read "Wellenplatte [°]"() -> (w594:refnum<k7>)
                n197 = invoke class="MG17Motor" method="StopCtrl"(reference=w594) -> (error out=w593:errorcluster)  [unwired: 2 in, 2 out]
                n198 = Unbundle By Name(w593) -> ("status"=w592:bool)
                n199 = local write "Wellenplatte"(w592) -> ()
              }
              frame #1 {
                n200 = property class="MG17Motor"(reference="Wellenplatte [°]", "HWSerialNum"="SN von Rotationsbühne") -> (reference out=w601:refnum<k7>, error out=w600:errorcluster)  [unwired: 1 in]
                n201 = invoke class="MG17Motor" method="StartCtrl"(reference=w601, error in=w600) -> (error out=w599:errorcluster)  [unwired: 1 in, 2 out]
                n202 = local write "Fehler (Ausgang)"(w599) -> ()
                n203 = Unbundle By Name(w599) -> ("status"=w598:bool)
                n204 = Not(x=w598) -> (.not. x?=w597:bool)
                n205 = local write "Wellenplatte"(w597) -> ()
              }
            }
          }
          event #2 {
            n206 = event-data() -> ("OldVal"=w602:dbl, "NewVal"=w608:dbl)  [unwired: 1 in]
            n207 = local read "Suppressor-Spannung [V]"() -> (w607:dbl)
            n208 = local read "Max. Spannungsdifferenz"() -> (w605:dbl)
            n209 = Subtract(x=w608, y=w607) -> (x-y=w606:dbl)
            n210 = local read "HV-Steuerung"() -> (w603:bool)
            n211 = Less Or Equal?(x=w606, y=w605) -> (x <= y?=w604:bool)
            n212 = case shown="True" w603 {
              tunnel: w604 -> [_ w610]
              tunnel: w602 -> [_ w609]
              frame #0 {
              }
              frame #1 {
                n213 = case shown="True" w610 {
                  tunnel: w609 -> [w611 _]
                  frame #0 {
                    n214 = local write "Tip-Spannung [V]"(w611) -> ()
                  }
                  frame #1 {
                    n215 = local read "Tip-Spannung [V]"() -> (w612:dbl)
                    n216 = call "HV_power_supply_set_voltage.vi"("Desired output voltage in V (HV power supply)"=w612, "Channel of HV power supply"=refnum<k21> "Dev0/Ao1") -> ("error out"=w613:errorcluster)  [unwired: 8 in]
                    n217 = local write "Fehler (Ausgang)"(w613) -> ()
                  }
                }
              }
            }
          }
          event #3 {
            n218 = event-data() -> ("OldVal"=w615:dbl, "NewVal"=w617:dbl)  [unwired: 1 in]
            n219 = local read "Tip-Spannung [V]"() -> (w616:dbl)
            n220 = local read "Max. Spannungsdifferenz"() -> (w618:dbl)
            n221 = Subtract(x=w616, y=w617) -> (x-y=w620:dbl)
            n222 = local read "HV-Steuerung"() -> (w621:bool)
            n223 = Less Or Equal?(x=w620, y=w618) -> (x <= y?=w619:bool)
            n224 = case shown="True" w621 {
              tunnel: w619 -> [_ w623]
              tunnel: w615 -> [_ w622]
              frame #0 {
              }
              frame #1 {
                n225 = case shown="True" w623 {
                  tunnel: w622 -> [w624 _]
                  frame #0 {
                    n226 = local write "Suppressor-Spannung [V]"(w624) -> ()
                  }
                  frame #1 {
                    n227 = local read "Suppressor-Spannung [V]"() -> (w625:dbl)
                    n228 = call "HV_power_supply_set_voltage.vi"("Desired output voltage in V (HV power supply)"=w625, "Channel of HV power supply"=refnum<k21> "Dev0/Ao0") -> ("error out"=w626:errorcluster)  [unwired: 8 in]
                    n229 = local write "Fehler (Ausgang)"(w626) -> ()
                  }
                }
              }
            }
          }
          event #4 {
            n230 = event-data() -> ()  [unwired: 1 in, 2 out]
          }
        }
        n231 = local read "Fehler (Ausgang)"() -> (w582:errorcluster)
        n232 = local read "Programm beenden"() -> (w581:bool)
        n233 = Unbundle By Name(w582) -> ("status"=w580:bool)
        n234 = Or(x=w580, y=w581) -> (x .or. y?=w577:bool)
        "Steuerschleifenzähler" <- w578
      }
      n235 = while "Kamera-Schleife" {
        i -> [w1587]
        stop <- w1588 stop-if-true
        n236 = local read "Fehler (Ausgang)"() -> (w1589:errorcluster)
        n237 = local read "Ereignis: FrameDone?"() -> (w1592:refnum<event-registration>)
        n238 = local read "Programm beenden"() -> (w1591:bool)
        n239 = Unbundle By Name(w1589) -> ("status"=w1590:bool)
        n240 = Or(x=w1590, y=w1591) -> (x .or. y?=w1588:bool)
        n241 = event "Kamera-Ereignisse" shown="[1] \"Kamera ON/OFF\": Wertänderung" {
          selector: w1592 -> [_ _ _ _ _ _]
          dyn-events: _ -> [_ _ _ _ _ _]
          timeout: 1000 -> [_ _ _ _ _ _]
          event #0 {
            n242 = event-data() -> ()  [unwired: 1 in, 2 out]
          }
          event #1 {
            n243 = event-data() -> ()  [unwired: 1 in, 4 out]
            n244 = local read "Detektionskamera"() -> (w1595:T5)
            n245 = local read "Kamera ON/OFF"() -> (w1596:bool)
            n246 = case shown="True" w1596 {
              tunnel: w1595 -> [w1597 w1602]
              tunnel: [w1600 w1603] -> w1594
              frame #0 {
                n247 = local read "Image Memory"() -> (w1598:T4)
                n248 = call "camera_release configuration_stop.vi"("Image Memory"=w1598, "Detektionskamera"=w1597) -> ("error out"=w1600:errorcluster, "status"=w1599:bool)
                n249 = local write "Kamera"(w1599) -> ()
              }
              frame #1 {
                n250 = local read "Buffer Interval"() -> (w1601:u32)
                n251 = call "camera_acquisition_continously.vi"("BufferInterval"=w1601, "Detektionskamera"=w1602) -> ("error out"=w1603:errorcluster, "Ereignis: FrameDone?"=w1604:refnum<event-registration>, "Image Memory"=w1605:T4, "Detektionskamera"=w1606:T5, "Kamera eingeschaltet?"=w1607:bool)
                n252 = local write "Kamera"(w1607) -> ()
                n253 = local write "Detektionskamera"(w1606) -> ()
                n254 = local write "Image Memory"(w1605) -> ()
                n255 = local write "Ereignis: FrameDone?"(w1604) -> ()
              }
            }
            n256 = local write "Fehler (Ausgang)"(w1594) -> ()
          }
          event #2 {
            w1620 = IMAQdx_Buffer_Number_Mode."Buffer Number"  # Buffer Number Mode
            n257 = event-data() -> ("ActualBufferNumber"=w1614:u32)  [unwired: 1 in]
            n258 = local read "Detektionskamera"() -> (w1619:T5)
            n259 = local read "Image Memory"() -> (w1618:T4)
            n260 = call <vilib>:"IMAQdx Get Image.vi"("Buffer Number Mode (Next)"=w1620, "Buffer Number In"=w1614, "Image In"=w1618, "Session In"=w1619) -> ("error out"=w1612:errorcluster, "Buffer Number Out"=w1615:u32, "Image Out"=w1611:T4, "Session Out"=w1616:T5)  [unwired: 1 in, 3 out]
            n261 = Not Equal?(x=w1615, y=w1614) -> (x != y?=w1613:bool)
            n262 = local write "Detektionskamera"(w1616) -> ()
            n263 = local write "Image Display"(w1611) -> ()
            n264 = call "IMAQ ImageToArray"("Image"=w1611) -> ("Image Pixels (U8)"=w1610:u8[][])  [unwired: 3 in, 4 out]
            n265 = local write "Image Memory"(w1611) -> ()
            n266 = local write "Buffer Number"(w1615) -> ()
            n267 = call "CalculateFPS.vi"("buffer number"=w1615) -> ("processed FPS"=w1617:dbl)  [unwired: 2 out]
            n268 = local write "Fehler (Ausgang)"(w1612) -> ()
            n269 = To Unsigned Quad Integer(1:w1610) -> (0:w1609:u64[][])
            n270 = local write "Frame Rate (FPS)"(w1617) -> ()
            n271 = local write "Buffer Overrun"(w1613) -> ()
            n272 = Add Array Elements(numeric array=w1609) -> (sum=w1608:u64)
            n273 = local write "Summierte Helligkeit (a.u.)"(w1608) -> ()
          }
          event #3 {
            n274 = event-data() -> ()  [unwired: 1 in, 2 out]
            n275 = local read "Kamera"() -> (w1621:bool)
            n276 = case shown="True" w1621 {
              frame #0 {
              }
              frame #1 {
                n277 = control-ref of="Shutter time (ms)"() -> (w1628:refnum<vi>)
                n278 = property class="Ring (strikt)"(reference=w1628) -> ("RingText.Text"=w1627:string)  [unwired: 1 in, 2 out]
                n279 = local read "Detektionskamera"() -> (w1626:T5)
                n280 = Decimal String To Number(string=w1627) -> (number=w1623:i32)  [unwired: 2 in, 1 out]
                n281 = property class="IMAQdx"(reference=w1626, "ActiveAttribute"="CameraAttributes::Shutter::Value", "ValueDBL"=w1623) -> (reference out=w1625:T5, error out=w1622:errorcluster)  [unwired: 1 in]
                n282 = local write "Detektionskamera"(w1625) -> ()
                n283 = local write "Fehler (Ausgang)"(w1622) -> ()
              }
            }
          }
          event #4 {
            n284 = event-data() -> ()  [unwired: 1 in, 1 out]
            n285 = local read "Kamera"() -> (w1629:bool)
            n286 = case shown="True" w1629 {
              frame #0 {
              }
              frame #1 {
                n287 = local read "Ereignis: FrameDone?"() -> (w1631:refnum<event-registration>)
                n288 = local read "Detektionskamera"() -> (w1635:T5)
                n289 = local read "Buffer Interval"() -> (w1634:u32)
                n290 = local read "ROI"() -> (w1636:i32[])
                n291 = call "camera_change_ROI.vi"("BufferInterval"=w1634, "Region of Interest"=w1636, "Ereignisregistrierung (Referenz) 2"=w1631, "Session In"=w1635) -> ("Fehler (Ausgang)"=w1630:errorcluster, "Ereignisregistrierung (Referenz)"=w1633:refnum<event-registration>, "Session Out"=w1632:T5)  [unwired: 5 in]
                n292 = local write "Detektionskamera"(w1632) -> ()
                n293 = local write "Ereignis: FrameDone?"(w1633) -> ()
                n294 = local write "Fehler (Ausgang)"(w1630) -> ()
              }
            }
          }
          event #5 {
            n295 = event-data() -> ("NewVal"=w1638:bool)  [unwired: 1 in, 1 out]
            n296 = local read "Kamera"() -> (w1639:bool)
            n297 = And(x=w1639, y=w1638) -> (x .and. y?=w1637:bool)
            n298 = case shown="True" w1637 {
              frame #0 {
              }
              frame #1 {
                n299 = local read "Ereignis: FrameDone?"() -> (w1642:refnum<event-registration>)
                n300 = local read "Detektionskamera"() -> (w1646:T5)
                n301 = local read "Buffer Interval"() -> (w1645:u32)
                n302 = call "camera_change_ROI.vi"("BufferInterval"=w1645, "Region of Interest"=i32[] [640, 480, 0, 0] ("Region of Interest (px)"), "Ereignisregistrierung (Referenz) 2"=w1642, "Session In"=w1646) -> ("Fehler (Ausgang)"=w1640:errorcluster, "Ereignisregistrierung (Referenz)"=w1644:refnum<event-registration>, "Session Out"=w1643:T5)  [unwired: 5 in]
                n303 = local write "Detektionskamera"(w1643) -> ()
                n304 = local write "Ereignis: FrameDone?"(w1644) -> ()
                n305 = local write "Fehler (Ausgang)"(w1640) -> ()
              }
            }
          }
        }
        "Kameraschleifenzähler" <- w1587
      }
      n306 = while "Spannungsscan-Schleife" {
        stop <- w401 stop-if-true
        n307 = local read "Fehler (Ausgang)"() -> (w402:errorcluster)
        n308 = local read "Spannungsscan läuft"() -> (w400:bool)
        n309 = local read "Programm beenden"() -> (w404:bool)
        n310 = Unbundle By Name(w402) -> ("status"=w403:bool)
        n311 = Or(x=w403, y=w404) -> (x .or. y?=w401:bool)
        n312 = case shown="True" w400 {
          frame #0 {
          }
          frame #1 {
            n313 = stacked-sequence {
              frame #0 {
                n314 = local read "# Spannungsschritte"() -> (w409:i32[])
                n315 = Index Array(array=w409, index #1=0 ("Index"), index #2=1 ("Index")) -> (element #1=w406:i32, element #2=w405:i32)
                n316 = for "Schleife für Tip-Spannung" {
                  N: w406 -> [_]
                  tunnel: w405 -> [w410]
                  i -> [w411]
                  n317 = local read "Spannungsscan läuft"() -> (w412:bool)
                  n318 = case shown="True" w412 {
                    tunnel: w411 -> [_ w414]
                    tunnel: w410 -> [_ w413]
                    frame #0 {
                    }
                    frame #1 {
                      n319 = stacked-sequence {
                        tunnel: w414 -> [w416 _]
                        tunnel: w413 -> [w415 _]
                        frame #0 {
                          n320 = for "Schleife für Suppressor-Spannung" {
                            N: w415 -> [_]
                            tunnel: w416 -> [w418]
                            i -> [w417]
                            n321 = local read "Spannungsscan läuft"() -> (w419:bool)
                            n322 = case shown="True" w419 {
                              tunnel: w418 -> [_ w421]
                              tunnel: w417 -> [_ w420]
                              frame #0 {
                              }
                              frame #1 {
                                n323 = stacked-sequence {
                                tunnel: w421 -> [_ _ w463 _]
                                tunnel: w420 -> [_ _ w462 _]
                                frame #0 {
                                n324 = local write "Summierte Helligkeit (a.u.)"(u64 0 ("Summierte Helligkeit (a.u.)")) -> ()
                                n325 = local read "ROI"() -> (w427:i32[])
                                n326 = local read "Aktueller Messschritt"() -> (w424:i32)
                                n327 = Index Array(array=w427, index #1=0 ("Index"), index #2=1 ("Index")) -> (element #1=w431:i32, element #2=w430:i32)
                                n328 = Initialize Array(u64 0 ("Element"), w430, w431) -> (w425:u64[][])
                                n329 = local write "Gemitteltes Bild"(w425) -> ()
                                n330 = Increment(x=w424) -> (x+1=w423:i32)
                                n331 = local write "Aktueller Messschritt"(w423) -> ()
                                }
                                frame #1 {
                                n332 = local read "# Bilder/Messschritt"() -> (w435:i32)
                                n333 = local read "Detektionskamera"() -> (w438:T5)
                                n334 = local read "Einzelbilder speichern"() -> (w433:bool)
                                n335 = call "camera_acquisition_sequence.vi"("Session In"=w438, "Desired image number"=w435) -> ("Image Array"=w432:T4[], "error out"=w437:errorcluster)  [unwired: 2 in, 1 out]
                                n336 = case shown="True" w433 {
                                tunnel: w437 -> [w440 w448]
                                tunnel: [w440 w447] -> w436
                                tunnel: w435 -> [w439 w446]
                                tunnel: [w439 w446] -> w434
                                tunnel: w432 -> [_ w445]
                                frame #0 {
                                }
                                frame #1 {
                                n337 = local read "Aktueller Messschritt"() -> (w451:i32)
                                n338 = local read "Save folder"() -> (w443:string)
                                n339 = Concatenate Strings(w443, "Einzelbilder\\" ("String")) -> (w441:string)
                                n340 = Format Into String(format string="%05.0f" ("Format-String"), initial string="#" ("Eingangs-String"), w451) -> (resulting string=w444:string)  [unwired: 1 in, 1 out]
                                n341 = call "save images.vi"("Save Folder"=w441, "File name prefix"=w444, "Array"=w445, "error out 2"=w448, "Bilder/Messschritt"=w446) -> ("error out"=w447:errorcluster)
                                }
                                }
                                n342 = for {
                                N: w434 -> [_]
                                tunnel: w436 -> [w457]
                                tunnel: w432 -> [w455] mode=indexing
                                n343 = call "IMAQ ImageToArray"("error in (no error)"=w457, "Image"=w455) -> ("error out"=w456:errorcluster, "Image Pixels (U8)"=w454:u8[][])  [unwired: 2 in, 3 out]
                                n344 = local read "Gemitteltes Bild"() -> (w452:u64[][])
                                n345 = To Unsigned Quad Integer(1:w454) -> (0:w459:u64[][])
                                n346 = local write "Fehler (Ausgang)"(w456) -> ()
                                n347 = Add Array Elements(numeric array=w459) -> (sum=w458:u64)
                                n348 = local read "Summierte Helligkeit (a.u.)"() -> (w460:u64)
                                n349 = Add(x=w452, y=w454) -> (x+y=w453:u64[][])
                                n350 = local write "Gemitteltes Bild"(w453) -> ()
                                n351 = Add(x=w458, y=w460) -> (x+y=w461:u64)
                                n352 = local write "Summierte Helligkeit (a.u.)"(w461) -> ()
                                }
                                }
                                frame #2 {
                                n353 = local read "# Bilder/Messschritt"() -> (w469:i32)
                                n354 = local read "2D-Intensitätsverteilung (MCP)"() -> (w466:dbl[][])
                                n355 = local read "Gemitteltes Bild"() -> (w467:u64[][])
                                n356 = local read "Summierte Helligkeit (a.u.)"() -> (w464:u64)
                                n357 = local read "Gemittelte Bilder speichern"() -> (w473:bool)
                                n358 = local read "Image Display"() -> (w471:T4)
                                n359 = Divide(x=w467, y=w469) -> (x/y=w468:dbl[][])
                                n360 = Replace Array Subset(array=w466, new element=w464, index (row)=w463, index (col)=w462) -> (w465:dbl[][])
                                n361 = call "IMAQ ArrayToImage"("Image Pixels (U8)"=w468, "Image"=w471) -> ("Image Out"=w470:T4)  [unwired: 8 in, 1 out]
                                n362 = local write "2D-Intensitätsverteilung (MCP)"(w465) -> ()
                                n363 = case shown="True" w473 {
                                tunnel: w470 -> [w474 w485]
                                tunnel: [w474 w476] -> w472
                                frame #0 {
                                }
                                frame #1 {
                                n364 = local read "Aktueller Messschritt"() -> (w480:i32)
                                n365 = local read "Save folder"() -> (w482:string)
                                n366 = Format Into String(format string="%05.0f" ("Format-String"), initial string="#" ("Eingangs-String"), w480) -> (resulting string=w479:string)  [unwired: 1 in, 1 out]
                                n367 = Concatenate Strings(w482, "Gemittelte Bilder\\" ("String"), w479, ".png" ("String")) -> (w478:string)
                                n368 = String To Path(string=w478) -> (path=w477:path)
                                n369 = call-poly "IMAQ Write File 2"("File Path"=w477, "Image"=w485) -> ("Image Out (duplicate)"=w476:T4)  [unwired: 8 in, 1 out]
                                }
                                }
                                n370 = local write "Image Display"(w472) -> ()
                                }
                                frame #3 {
                                n371 = flat-sequence {
                                frame #0 {
                                n372 = local read "Aktuelle Spannung [V]"() -> (w488:dbl[])
                                n373 = local read "Spannungsschritt [V]"() -> (w492:dbl[])
                                n374 = Index Array(array=w488, index=1 ("Index")) -> (element=w490:dbl)
                                n375 = Index Array(array=w492, index=1 ("Index")) -> (element=w491:dbl)
                                n376 = Add(x=w490, y=w491) -> (x+y=w486:dbl)
                                n377 = local write "Suppressor-Spannung [V]"(w486) -> ()
                                n378 = call "HV_power_supply_set_voltage.vi"("Desired output voltage in V (HV power supply)"=w486, "Channel of HV power supply"=refnum<k21> "Dev0/Ao0") -> ("error out"=w495:errorcluster)  [unwired: 8 in]
                                n379 = Replace Array Subset(array=w488, new element=w486, index=1 ("Index")) -> (w487:dbl[])
                                n380 = local write "Fehler (Ausgang)"(w495) -> ()
                                n381 = local write "Aktuelle Spannung [V]"(w487) -> ()
                                }
                                frame #1 {
                                # "Wartezeit für\nneue Spannung"
                                n382 = Wait (ms)(milliseconds to wait=u32 200 ("Zu wartende ms")) -> ()  [unwired: 1 out]
                                }
                                frame #2 {
                                n383 = local read "Aktueller Messschritt"() -> (w499:i32)
                                n384 = local read "Start time [ms]"() -> (w501:timestamp)
                                n385 = local read "# Messschritte"() -> (w500:i32)
                                n386 = call "estimate_stopp_time.vi"("Aktueller Messschritt"=w499, "# Messschritte"=w500, "Startzeit"=w501) -> ("Stopp Zeit"=w498:string)  [unwired: 8 in]
                                n387 = local write "Geschätzte Messzeit"(w498) -> ()
                                }
                                }
                                }
                                }
                              }
                            }
                          }
                        }
                        frame #1 {
                          n388 = flat-sequence {
                            frame #0 {
                              n389 = local read "Spannungsstart [V]"() -> (w507:dbl[])
                              n390 = local read "Aktuelle Spannung [V]"() -> (w509:dbl[])
                              n391 = Index Array(array=w507, index=1 ("Index")) -> (element=w502:dbl)
                              n392 = call "HV_power_supply_set_voltage.vi"("Desired output voltage in V (HV power supply)"=w502, "Channel of HV power supply"=refnum<k21> "Dev0/Ao0") -> ("error out"=w503:errorcluster)  [unwired: 8 in]
                              n393 = local write "Suppressor-Spannung [V]"(w502) -> ()
                              n394 = Replace Array Subset(array=w509, new element=w502, index=1 ("Index")) -> (w505:dbl[])
                              n395 = local write "Fehler (Ausgang)"(w503) -> ()
                              n396 = local write "Aktuelle Spannung [V]"(w505) -> ()
                            }
                            frame #1 {
                              n397 = local read "Aktuelle Spannung [V]"() -> (w512:dbl[])
                              n398 = local read "Spannungsschritt [V]"() -> (w516:dbl[])
                              n399 = Index Array(array=w512, index=0 ("Index")) -> (element=w514:dbl)
                              n400 = Index Array(array=w516, index=0 ("Index")) -> (element=w515:dbl)
                              n401 = Add(x=w514, y=w515) -> (x+y=w510:dbl)
                              n402 = call "HV_power_supply_set_voltage.vi"("Desired output voltage in V (HV power supply)"=w510, "Channel of HV power supply"=refnum<k21> "Dev0/Ao1") -> ("error out"=w519:errorcluster)  [unwired: 8 in]
                              n403 = local write "Tip-Spannung [V]"(w510) -> ()
                              n404 = local write "Fehler (Ausgang)"(w519) -> ()
                              n405 = Replace Array Subset(array=w512, new element=w510, index=0 ("Index")) -> (w511:dbl[])
                              n406 = local write "Aktuelle Spannung [V]"(w511) -> ()
                            }
                            frame #2 {
                              # "Wartezeit für\nStartspannung"
                              n407 = Wait (ms)(milliseconds to wait=u32 6000 ("Zu wartende ms")) -> ()  [unwired: 1 out]
                            }
                          }
                        }
                      }
                    }
                  }
                }
              }
              frame #1 {
                n408 = local read "Spannungsscan läuft"() -> (w522:bool)
                n409 = case shown="False" w522 {
                  frame #0 {
                    n410 = flat-sequence {
                      frame #0 {
                        # "Zur Ausgangsposition zurückfahren"
                        n411 = local read "Spannungsstart [V]"() -> (w528:dbl[])
                        n412 = local read "Spannungsstart [V]"() -> (w523:dbl[])
                        n413 = local read "Detektionskamera"() -> (w535:T5)
                        n414 = local read "Buffer Interval"() -> (w534:u32)
                        n415 = local write "Aktuelle Spannung [V]"(w523) -> ()
                        n416 = call "camera_create_configuration.vi"("BufferInterval"=w534, "Session Out 2"=w535) -> ("Fehler (Ausgang)"=w529:errorcluster, "Ereignisregistrierung (Referenz)"=w536:refnum<event-registration>)  [unwired: 1 in, 1 out]
                        n417 = Index Array(array=w528, index #1=0 ("Index"), index #2=1 ("Index")) -> (element #1=w524:dbl, element #2=w525:dbl)
                        n418 = local write "Tip-Spannung [V]"(w524) -> ()
                        n419 = local write "Suppressor-Spannung [V]"(w525) -> ()
                        n420 = local write "Ereignis: FrameDone?"(w536) -> ()
                        n421 = call "HV_power_supply_set_voltage.vi"("error in"=w529, "Desired output voltage in V (HV power supply)"=w525, "Channel of HV power supply"=refnum<k21> "Dev0/Ao0") -> ("error out"=w531:errorcluster)  [unwired: 7 in]
                        n422 = call "HV_power_supply_set_voltage.vi"("error in"=w531, "Desired output voltage in V (HV power supply)"=w524, "Channel of HV power supply"=refnum<k21> "Dev0/Ao1") -> ("error out"=w530:errorcluster)  [unwired: 7 in]
                        n423 = local write "Fehler (Ausgang)"(w530) -> ()
                      }
                    }
                  }
                  frame #1 {
                    n424 = flat-sequence {
                      frame #0 {
                        n425 = local read "2D-Intensitätsverteilung (MCP)"() -> (w537:dbl[][])
                        n426 = control-ref of="2D-Intensitätsverteilung (MCP)"() -> (w540:refnum<vi>)
                        n427 = Array Max & Min(array=w537) -> (max value=w538:dbl, min value=w539:dbl)  [unwired: 2 out]
                        n428 = property class="IntGraph (strikt)"(reference=w540, "ZScale.Maximum"=w538, "ZScale.Minimum"=w539) -> ()  [unwired: 1 in, 2 out]
                      }
                      frame #1 {
                        # "Zur Ausgangsposition zurückfahren"
                        n429 = local read "Spannungsstart [V]"() -> (w541:dbl[])
                        n430 = local read "Spannungsstart [V]"() -> (w546:dbl[])
                        n431 = local read "Detektionskamera"() -> (w553:T5)
                        n432 = local read "Buffer Interval"() -> (w552:u32)
                        n433 = local write "Aktuelle Spannung [V]"(w541) -> ()
                        n434 = call "camera_create_configuration.vi"("BufferInterval"=w552, "Session Out 2"=w553) -> ("Fehler (Ausgang)"=w547:errorcluster, "Ereignisregistrierung (Referenz)"=w554:refnum<event-registration>)  [unwired: 1 in, 1 out]
                        n435 = Index Array(array=w546, index #1=0 ("Index"), index #2=1 ("Index")) -> (element #1=w542:dbl, element #2=w543:dbl)
                        n436 = local write "Tip-Spannung [V]"(w542) -> ()
                        n437 = local write "Suppressor-Spannung [V]"(w543) -> ()
                        n438 = local write "Ereignis: FrameDone?"(w554) -> ()
                        n439 = call "HV_power_supply_set_voltage.vi"("error in"=w547, "Desired output voltage in V (HV power supply)"=w543, "Channel of HV power supply"=refnum<k21> "Dev0/Ao0") -> ("error out"=w549:errorcluster)  [unwired: 7 in]
                        n440 = call "HV_power_supply_set_voltage.vi"("error in"=w549, "Desired output voltage in V (HV power supply)"=w542, "Channel of HV power supply"=refnum<k21> "Dev0/Ao1") -> ("error out"=w548:errorcluster)  [unwired: 7 in]
                        n441 = local write "Fehler (Ausgang)"(w548) -> ()
                      }
                      frame #2 {
                        n442 = local read "Daten speichern"() -> (w555:bool)
                        n443 = case shown="True" w555 {
                          frame #0 {
                          }
                          frame #1 {
                            w556 = 1 ("Index")
                            w568 = 0 ("Index")
                            n444 = local read "Spannungsschritt [V]"() -> (w566:dbl[])
                            n445 = local read "# Spannungsschritte"() -> (w567:i32[])
                            n446 = local read "Spannungsstart [V]"() -> (w565:dbl[])
                            n447 = local read "Save folder"() -> (w557:string)
                            n448 = Index Array(array=w565, index #1=w568, index #2=w556) -> (element #1=w564:dbl, element #2=w560:dbl)
                            n449 = Index Array(array=w566, index #1=w568, index #2=w556) -> (element #1=w563:dbl, element #2=w559:dbl)
                            n450 = Index Array(array=w567, index #1=w568, index #2=w556) -> (element #1=w562:i32, element #2=w558:i32)
                            n451 = local read "2D-Intensitätsverteilung (MCP)"() -> (w574:dbl[][])
                            n452 = call "create_axis_vector_file.vi"("Save folder"=w557, "Dateiname"="xAchse.dat" ("Save folder"), "Start"=w564, "Schrittlänge"=w563, "# Schritte"=w562) -> ()  [unwired: 11 in]
                            n453 = call "create_axis_vector_file.vi"("Save folder"=w557, "Dateiname"="yAchse.dat", "Start"=w560, "Schrittlänge"=w559, "# Schritte"=w558) -> ()  [unwired: 11 in]
                            n454 = Concatenate Strings(w557, "\\" ("String"), "2D_Intensitaetsverteilung_MCP.dat" ("String")) -> (w571:string)
                            n455 = String To Path(string=w571) -> (path=w572:path)
                            n456 = call-poly <vilib>:"Write To Spreadsheet File.vi"("format (%.3f)"="%.;%8.0f", "2D data"=w574, "file path (dialog if empty)"=w572) -> ()  [unwired: 5 in, 1 out]
                          }
                        }
                      }
                      frame #3 {
                        w576 = FALSE ("Spannungsscan läuft")
                        n457 = local write "Spannungsscan ON/OFF"(w576) -> ()
                        n458 = local write "Spannungsscan läuft"(w576) -> ()
                      }
                    }
                  }
                }
              }
            }
          }
        }
      }
      n459 = while "x-U-Scan Schleife" {
        stop <- w223 stop-if-true
        n460 = local read "Fehler (Ausgang)"() -> (w224:errorcluster)
        n461 = local read "x-U-Scan läuft"() -> (w222:bool)
        n462 = local read "Programm beenden"() -> (w226:bool)
        n463 = case shown="True" w222 {
          frame #0 {
          }
          frame #1 {
            n464 = stacked-sequence {
              frame #0 {
                n465 = local read "# x-U-Scan x-Rasterschritte"() -> (w227:i32)
                n466 = for "Schleife für Raumkoordinate" {
                  N: w227 -> [_]
                  i -> [w228]
                  n467 = local read "x-U-Scan läuft"() -> (w229:bool)
                  n468 = case shown="True" w229 {
                    tunnel: w228 -> [_ w230]
                    frame #0 {
                    }
                    frame #1 {
                      n469 = stacked-sequence {
                        tunnel: w230 -> [w232 _]
                        frame #0 {
                          n470 = local read "# x-U-Scan Spannungsschritte"() -> (w231:i32)
                          n471 = for "Schleife für Spannungskoordinate" {
                            N: w231 -> [_]
                            tunnel: w232 -> [w234]
                            i -> [w233]
                            n472 = local read "x-U-Scan läuft"() -> (w235:bool)
                            n473 = case shown="True" w235 {
                              tunnel: w234 -> [_ w237]
                              tunnel: w233 -> [_ w236]
                              frame #0 {
                              }
                              frame #1 {
                                n474 = stacked-sequence {
                                tunnel: w237 -> [_ _ w279 _]
                                tunnel: w236 -> [_ _ w278 _]
                                frame #0 {
                                n475 = local read "ROI"() -> (w243:i32[])
                                n476 = local write "Summierte Helligkeit (a.u.)"(u64 0 ("Summierte Helligkeit (a.u.)")) -> ()
                                n477 = local read "Aktueller Messschritt"() -> (w240:i32)
                                n478 = Index Array(array=w243, index #1=0 ("Index"), index #2=1 ("Index")) -> (element #1=w247:i32, element #2=w246:i32)
                                n479 = Initialize Array(u64 0 ("Element"), w246, w247) -> (w241:u64[][])
                                n480 = local write "Gemitteltes Bild"(w241) -> ()
                                n481 = Increment(x=w240) -> (x+1=w239:i32)
                                n482 = local write "Aktueller Messschritt"(w239) -> ()
                                }
                                frame #1 {
                                n483 = local read "# Bilder/Messschritt"() -> (w251:i32)
                                n484 = local read "Detektionskamera"() -> (w254:T5)
                                n485 = local read "Einzelbilder speichern"() -> (w249:bool)
                                n486 = call "camera_acquisition_sequence.vi"("Session In"=w254, "Desired image number"=w251) -> ("Image Array"=w248:T4[], "error out"=w253:errorcluster)  [unwired: 2 in, 1 out]
                                n487 = case shown="True" w249 {
                                tunnel: w253 -> [w256 w264]
                                tunnel: [w256 w263] -> w252
                                tunnel: w251 -> [w255 w262]
                                tunnel: [w255 w262] -> w250
                                tunnel: w248 -> [_ w261]
                                frame #0 {
                                }
                                frame #1 {
                                n488 = local read "Aktueller Messschritt"() -> (w267:i32)
                                n489 = local read "Save folder"() -> (w259:string)
                                n490 = Concatenate Strings(w259, "Einzelbilder\\" ("String")) -> (w257:string)
                                n491 = Format Into String(format string="%05.0f" ("Format-String"), initial string="#" ("Eingangs-String"), w267) -> (resulting string=w260:string)  [unwired: 1 in, 1 out]
                                n492 = call "save images.vi"("Save Folder"=w257, "File name prefix"=w260, "Array"=w261, "error out 2"=w264, "Bilder/Messschritt"=w262) -> ("error out"=w263:errorcluster)
                                }
                                }
                                n493 = for {
                                N: w250 -> [_]
                                tunnel: w252 -> [w273]
                                tunnel: w248 -> [w271] mode=indexing
                                n494 = call "IMAQ ImageToArray"("error in (no error)"=w273, "Image"=w271) -> ("error out"=w272:errorcluster, "Image Pixels (U8)"=w270:u8[][])  [unwired: 2 in, 3 out]
                                n495 = local read "Gemitteltes Bild"() -> (w268:u64[][])
                                n496 = To Unsigned Quad Integer(1:w270) -> (0:w275:u64[][])
                                n497 = local write "Fehler (Ausgang)"(w272) -> ()
                                n498 = local read "Summierte Helligkeit (a.u.)"() -> (w276:u64)
                                n499 = Add Array Elements(numeric array=w275) -> (sum=w274:u64)
                                n500 = Add(x=w268, y=w270) -> (x+y=w269:u64[][])
                                n501 = local write "Gemitteltes Bild"(w269) -> ()
                                n502 = Add(x=w274, y=w276) -> (x+y=w277:u64)
                                n503 = local write "Summierte Helligkeit (a.u.)"(w277) -> ()
                                }
                                }
                                frame #2 {
                                n504 = local read "# Bilder/Messschritt"() -> (w285:i32)
                                n505 = local read "2D-Intensitätsverteilung (MCP)"() -> (w282:dbl[][])
                                n506 = local read "Gemitteltes Bild"() -> (w283:u64[][])
                                n507 = local read "Summierte Helligkeit (a.u.)"() -> (w280:u64)
                                n508 = local read "Gemittelte Bilder speichern"() -> (w289:bool)
                                n509 = local read "Image Display"() -> (w287:T4)
                                n510 = Divide(x=w283, y=w285) -> (x/y=w284:dbl[][])
                                n511 = call "IMAQ ArrayToImage"("Image Pixels (U8)"=w284, "Image"=w287) -> ("Image Out"=w286:T4)  [unwired: 8 in, 1 out]
                                n512 = Replace Array Subset(array=w282, new element=w280, index (row)=w279, index (col)=w278) -> (w281:dbl[][])
                                n513 = case shown="True" w289 {
                                tunnel: w286 -> [w290 w301]
                                tunnel: [w290 w292] -> w288
                                frame #0 {
                                }
                                frame #1 {
                                n514 = local read "Aktueller Messschritt"() -> (w296:i32)
                                n515 = local read "Save folder"() -> (w298:string)
                                n516 = Format Into String(format string="%05.0f" ("Format-String"), initial string="#" ("Eingangs-String"), w296) -> (resulting string=w295:string)  [unwired: 1 in, 1 out]
                                n517 = Concatenate Strings(w298, "Gemittelte Bilder\\" ("String"), w295, ".png" ("String")) -> (w294:string)
                                n518 = String To Path(string=w294) -> (path=w293:path)
                                n519 = call-poly "IMAQ Write File 2"("File Path"=w293, "Image"=w301) -> ("Image Out (duplicate)"=w292:T4)  [unwired: 8 in, 1 out]
                                }
                                }
                                n520 = local write "2D-Intensitätsverteilung (MCP)"(w281) -> ()
                                n521 = local write "Image Display"(w288) -> ()
                                }
                                frame #3 {
                                n522 = flat-sequence {
                                frame #0 {
                                n523 = local read "x-U-Scan aktuelle Spannung [V]"() -> (w304:dbl)
                                n524 = local read "x-U-Scan Spannungsschritt [V]"() -> (w305:dbl)
                                n525 = local read "Spannungskanal"() -> (w303:refnum<k21>)
                                n526 = Add(x=w304, y=w305) -> (x+y=w302:dbl)
                                n527 = call "HV_power_supply_set_voltage.vi"("Desired output voltage in V (HV power supply)"=w302, "Channel of HV power supply"=w303) -> ("error out"=w306:errorcluster)  [unwired: 8 in]
                                n528 = local write "x-U-Scan aktuelle Spannung [V]"(w302) -> ()
                                n529 = local write "Fehler (Ausgang)"(w306) -> ()
                                }
                                frame #1 {
                                # "Wartezeit für\nneue Spannung"
                                n530 = Wait (ms)(milliseconds to wait=u32 200 ("Zu wartende ms")) -> ()  [unwired: 1 out]
                                }
                                frame #2 {
                                n531 = local read "Aktueller Messschritt"() -> (w309:i32)
                                n532 = local read "# Messschritte"() -> (w310:i32)
                                n533 = local read "Start time [ms]"() -> (w311:timestamp)
                                n534 = call "estimate_stopp_time.vi"("Aktueller Messschritt"=w309, "# Messschritte"=w310, "Startzeit"=w311) -> ("Stopp Zeit"=w308:string)  [unwired: 8 in]
                                n535 = local write "Geschätzte Messzeit"(w308) -> ()
                                }
                                }
                                }
                                }
                              }
                            }
                          }
                        }
                        frame #1 {
                          n536 = flat-sequence {
                            frame #0 {
                              n537 = local read "x-U-Scan Spannungsstart [V]"() -> (w312:dbl)
                              n538 = local read "Spannungskanal"() -> (w313:refnum<k21>)
                              n539 = call "HV_power_supply_set_voltage.vi"("Desired output voltage in V (HV power supply)"=w312, "Channel of HV power supply"=w313) -> ("error out"=w314:errorcluster)  [unwired: 8 in]
                              n540 = local write "x-U-Scan aktuelle Spannung [V]"(w312) -> ()
                              n541 = local write "Fehler (Ausgang)"(w314) -> ()
                            }
                            frame #1 {
                              # "Fahre nächste x-Position an"
                              n542 = local read "x-U-Scan x-Rasterschritt [µm]"() -> (w319:dbl)
                              n543 = local read "Achs-ID"() -> (w318:i32)
                              n544 = Decrement(x=w318) -> (x-1=w317:i32)
                              n545 = call "stage_move_axis_relative.vi"("Achse"=w318, "Schrittweite [µm]"=w319) -> ("xyz-Position OUT [mm]"=w316:dbl[])  [unwired: 1 in, 2 out]
                              n546 = Index Array(array=w316, index=w317) -> (element=w315:dbl)
                              n547 = local write "x-U-Scan aktuelle x-Position [mm]"(w315) -> ()
                            }
                            frame #2 {
                              n548 = local read "x-U-Scan (Ausgleichslage) Steigung"() -> (w321:dbl)
                              n549 = Not Equal?(x=w321, y=0.0) -> (x != y?=w322:bool)
                              n550 = case shown="True" w322 {
                                frame #0 {
                                }
                                frame #1 {
                                # "Fahre nächste y-Position an"
                                n551 = local read "Raum-Koordinate 2 (Lagenausgleich)"() -> (w323:enum16{"x-Achse", "y-Achse", "z-Achse"})
                                n552 = local read "x-U-Scan (Ausgleichslage) Steigung"() -> (w325:dbl)
                                n553 = local read "x-U-Scan x-Rasterschritt [µm]"() -> (w327:dbl)
                                n554 = Multiply(x=w327, y=w325) -> (x*y=w326:dbl)
                                n555 = Increment(x=w323) -> (x+1=w324:enum16{"x-Achse", "y-Achse", "z-Achse"})
                                n556 = call "stage_move_axis_relative.vi"("Achse"=w324, "Schrittweite [µm]"=w326) -> ("xyz-Position OUT [mm]"=w328:dbl[])  [unwired: 1 in, 2 out]
                                n557 = Index Array(array=w328, index=w323) -> (element=w329:dbl)
                                n558 = local write "x-U-Scan aktuelle y-Position [mm]"(w329) -> ()
                                }
                              }
                            }
                            frame #3 {
                              # "Wartezeit für\nStartspannung"
                              n559 = Wait (ms)(milliseconds to wait=u32 6000 ("Zu wartende ms")) -> ()  [unwired: 1 out]
                            }
                          }
                        }
                      }
                    }
                  }
                }
              }
              frame #1 {
                n560 = local read "x-U-Scan läuft"() -> (w331:bool)
                n561 = case shown="True" w331 {
                  frame #0 {
                    n562 = flat-sequence {
                      frame #0 {
                        # "Zur Ausgangsposition zurückfahren"
                        n563 = local read "x-U-Scan x-Startposition [mm]"() -> (w332:dbl)
                        n564 = local read "Aktuelle xyz-Position [mm]"() -> (w335:dbl[])
                        n565 = local read "Achs-ID"() -> (w333:i32)
                        n566 = local read "x-U-Scan Spannungsstart [V]"() -> (w339:dbl)
                        n567 = Decrement(x=w333) -> (x-1=w334:i32)
                        n568 = Replace Array Subset(array=w335, new element=w332, index=w334) -> (w336:dbl[])
                        n569 = local read "Detektionskamera"() -> (w343:T5)
                        n570 = local read "Buffer Interval"() -> (w342:u32)
                        n571 = call "stage_move_axis_absolute.vi"("Ziel xyz IN [mm]"=w336, "Achse"=w333) -> ("error out"=w337:errorcluster)  [unwired: 1 in, 2 out]
                        n572 = local write "x-U-Scan aktuelle Spannung [V]"(w339) -> ()
                        n573 = local read "Spannungskanal"() -> (w340:refnum<k21>)
                        n574 = call "camera_create_configuration.vi"("error in"=w337, "BufferInterval"=w342, "Session Out 2"=w343) -> ("Fehler (Ausgang)"=w341:errorcluster, "Ereignisregistrierung (Referenz)"=w344:refnum<event-registration>)  [unwired: 1 out]
                        n575 = local write "Ereignis: FrameDone?"(w344) -> ()
                        n576 = call "HV_power_supply_set_voltage.vi"("error in"=w341, "Desired output voltage in V (HV power supply)"=w339, "Channel of HV power supply"=w340) -> ("error out"=w338:errorcluster)  [unwired: 7 in]
                        n577 = local write "Fehler (Ausgang)"(w338) -> ()
                      }
                    }
                  }
                  frame #1 {
                    n578 = flat-sequence {
                      frame #0 {
                        n579 = local read "2D-Intensitätsverteilung (MCP)"() -> (w345:dbl[][])
                        n580 = control-ref of="2D-Intensitätsverteilung (MCP)"() -> (w348:refnum<vi>)
                        n581 = Array Max & Min(array=w345) -> (max value=w346:dbl, min value=w347:dbl)  [unwired: 2 out]
                        n582 = property class="IntGraph (strikt)"(reference=w348, "ZScale.Maximum"=w346, "ZScale.Minimum"=w347) -> ()  [unwired: 1 in, 2 out]
                      }
                      frame #1 {
                        # "Zur Ausgangsposition zurückfahren"
                        n583 = local read "Start xyz-Position [mm]"() -> (w353:dbl[])
                        n584 = local read "x-U-Scan Spannungsstart [V]"() -> (w358:dbl)
                        n585 = local read "x-U-Scan Spannungsstart [V]"() -> (w356:dbl)
                        n586 = local read "Detektionskamera"() -> (w361:T5)
                        n587 = local read "Achs-ID"() -> (w350:i32)
                        n588 = local read "Buffer Interval"() -> (w360:u32)
                        n589 = local read "Spannungskanal"() -> (w357:refnum<k21>)
                        n590 = Decrement(x=w350) -> (x-1=w351:i32)
                        n591 = call "stage_move_axis_absolute.vi"("Ziel xyz IN [mm]"=w353, "Achse"=w350) -> ("error out"=w354:errorcluster, "Ziel xyz OUT [mm]"=w352:dbl[])  [unwired: 1 in, 1 out]
                        n592 = local write "x-U-Scan aktuelle Spannung [V]"(w358) -> ()
                        n593 = call "camera_create_configuration.vi"("error in"=w354, "BufferInterval"=w360, "Session Out 2"=w361) -> ("Fehler (Ausgang)"=w355:errorcluster, "Ereignisregistrierung (Referenz)"=w362:refnum<event-registration>)  [unwired: 1 out]
                        n594 = Index Array(array=w352, index=w351) -> (element=w349:dbl)
                        n595 = local write "x-U-Scan aktuelle Spannung [V]"(w356) -> ()
                        n596 = local write "x-U-Scan aktuelle x-Position [mm]"(w349) -> ()
                        n597 = local write "Ereignis: FrameDone?"(w362) -> ()
                        n598 = call "HV_power_supply_set_voltage.vi"("error in"=w355, "Desired output voltage in V (HV power supply)"=w356, "Channel of HV power supply"=w357) -> ("error out"=w359:errorcluster)  [unwired: 7 in]
                        n599 = local write "Fehler (Ausgang)"(w359) -> ()
                      }
                      frame #2 {
                        n600 = local read "x-U-Scan (Ausgleichslage) Steigung"() -> (w364:dbl)
                        n601 = Not Equal?(x=w364, y=0.0) -> (x != y?=w363:bool)
                        n602 = case shown="True" w363 {
                          frame #0 {
                          }
                          frame #1 {
                            n603 = local read "Raum-Koordinate 2 (Lagenausgleich)"() -> (w366:enum16{"x-Achse", "y-Achse", "z-Achse"})
                            n604 = local read "Start xyz-Position [mm]"() -> (w368:dbl[])
                            n605 = Increment(x=w366) -> (x+1=w367:enum16{"x-Achse", "y-Achse", "z-Achse"})
                            n606 = call "stage_move_axis_absolute.vi"("Ziel xyz IN [mm]"=w368, "Achse"=w367) -> ("Ziel xyz OUT [mm]"=w369:dbl[])  [unwired: 1 in, 2 out]
                            n607 = Index Array(array=w369, index=w366) -> (element=w370:dbl)
                            n608 = local write "x-U-Scan aktuelle y-Position [mm]"(w370) -> ()
                          }
                        }
                      }
                      frame #3 {
                        n609 = local read "Daten speichern"() -> (w371:bool)
                        n610 = case shown="True" w371 {
                          frame #0 {
                          }
                          frame #1 {
                            n611 = local read "x-U-Scan x-Rasterschritt [µm]"() -> (w379:dbl)
                            n612 = local read "x-U-Scan (Ausgleichslage) Steigung"() -> (w373:dbl)
                            n613 = local read "# x-U-Scan Spannungsschritte"() -> (w381:i32)
                            n614 = local read "x-U-Scan Spannungsschritt [V]"() -> (w382:dbl)
                            n615 = local read "x-U-Scan x-Startposition [mm]"() -> (w380:dbl)
                            n616 = local read "x-U-Scan Spannungsstart [V]"() -> (w383:dbl)
                            n617 = local read "# x-U-Scan x-Rasterschritte"() -> (w375:i32)
                            n618 = Divide(x=w379, y=1000.0) -> (x/y=w376:dbl)
                            n619 = local read "Save folder"() -> (w377:string)
                            n620 = Not Equal?(x=w373, y=0.0) -> (x != y?=w374:bool)
                            n621 = local read "2D-Intensitätsverteilung (MCP)"() -> (w390:dbl[][])
                            n622 = call "create_axis_vector_file.vi"("Save folder"=w377, "Dateiname"="yAchse.dat", "Start"=w383, "Schrittlänge"=w382, "# Schritte"=w381) -> ()  [unwired: 11 in]
                            n623 = case shown="True" w374 {
                              tunnel: w377 -> [_ w398]
                              tunnel: w376 -> [_ w395]
                              tunnel: w375 -> [_ w392]
                              frame #0 {
                              }
                              frame #1 {
                                n624 = local read "x-U-Scan (Ausgleichslage) Steigung"() -> (w396:dbl)
                                n625 = local read "x-U-Scan y-Startposition [mm]"() -> (w393:dbl)
                                n626 = Multiply(x=w395, y=w396) -> (x*y=w394:dbl)
                                n627 = call "create_axis_vector_file.vi"("Save folder"=w398, "Dateiname"="zAchse.dat", "Start"=w393, "Schrittlänge"=w394, "# Schritte"=w392) -> ()  [unwired: 11 in]
                              }
                            }
                            n628 = call "create_axis_vector_file.vi"("Save folder"=w377, "Dateiname"="xAchse.dat", "Start"=w380, "Schrittlänge"=w376, "# Schritte"=w375) -> ()  [unwired: 11 in]
                            n629 = Concatenate Strings(w377, "\\" ("String"), "2D_Intensitaetsverteilung_MCP.dat" ("String")) -> (w387:string)
                            n630 = String To Path(string=w387) -> (path=w388:path)
                            n631 = call-poly <vilib>:"Write To Spreadsheet File.vi"("format (%.3f)"="%.;%8.0f", "2D data"=w390, "file path (dialog if empty)"=w388) -> ()  [unwired: 5 in, 1 out]
                          }
                        }
                      }
                      frame #4 {
                        w399 = FALSE ("Spannungsscan läuft")
                        n632 = local write "x-U-Scan ON/OFF"(w399) -> ()
                        n633 = local write "x-U-Scan läuft"(w399) -> ()
                      }
                    }
                  }
                }
              }
            }
          }
        }
        n634 = Unbundle By Name(w224) -> ("status"=w225:bool)
        n635 = Or(x=w225, y=w226) -> (x .or. y?=w223:bool)
      }
      n636 = while "Mess-Schleife" {
        tunnel: w63 -> [w630]
        i -> [w629]
        stop <- w628 stop-if-true
        n637 = event "Scan-Ereignisse" shown="[4] \"Leistungs-/Polarisationsscan ON/OFF\": Wertänderung" {
          selector: w630 -> [_ _ _ _ _ _ _ _ _ _]
          dyn-events: _ -> [_ _ _ _ _ _ _ _ _ _]
          timeout: 1000 -> [_ _ _ _ _ _ _ _ _ _]
          event #0 {
            n638 = event-data() -> ()  [unwired: 1 in, 2 out]
          }
          event #1 {
            n639 = event-data() -> ("NewVal"=w637:bool)  [unwired: 1 in]
            n640 = local read "Kamera"() -> (w636:bool)
            n641 = And(x=w636, y=w637) -> (x .and. y?=w635:bool)
            n642 = case shown="True" w635 {
              frame #0 {
                n643 = local write "Rasterung läuft"(FALSE ("Rasterung läuft")) -> ()
              }
              frame #1 {
                n644 = stacked-sequence {
                  frame #0 {
                    n645 = flat-sequence {
                      tunnel: [w649] -> w639
                      tunnel: w639 -> [w717]
                      frame #0 {
                        n646 = Get Date/Time In Seconds() -> (seconds since 1Jan1904=w640:timestamp)
                        n647 = local write "Start time [ms]"(w640) -> ()
                        n648 = local read "Rasterweite [µm]"() -> (w660:dbl[])
                        n649 = local read "# Rasterschritte"() -> (w662:i32[])
                        n650 = control-ref of="Shutter time (ms)"() -> (w657:refnum<vi>)
                        n651 = local read "Rasterart"() -> (w663:T2)
                        n652 = case shown="\"2D-Scan(xz)\"" w663 {
                          tunnel: w662 -> [w671 w687 w692 w701 w707]
                          tunnel: [w670 w686 w693 w700 w704] -> w661
                          tunnel: w660 -> [w669 w677 w689 w697 w706]
                          tunnel: [w668 w676 w688 w696 w705] -> w659
                          frame #0 {
                            n653 = Replace Array Subset(array=w671, new element #1=1 ("Neues Element/Teil-Array"), index #1=1 ("Index"), new element #2=1 ("Neues Element/Teil-Array"), index #2=2 ("Index")) -> (w670:i32[])
                            n654 = Replace Array Subset(array=w669, new element #1=0.0 ("Neues Element/Teil-Array"), index #1=1 ("Index"), new element #2=0.0 ("Neues Element/Teil-Array"), index #2=2 ("Index")) -> (w668:dbl[])
                          }
                          frame #1 {
                            n655 = Replace Array Subset(array=w687, new element #1=1 ("Neues Element/Teil-Array"), index #1=0 ("Index"), new element #2=1 ("Neues Element/Teil-Array"), index #2=1 ("Index")) -> (w686:i32[])
                            n656 = Replace Array Subset(array=w677, new element #1=0.0 ("Neues Element/Teil-Array"), index #1=0 ("Index"), new element #2=0.0 ("Neues Element/Teil-Array"), index #2=1 ("Index")) -> (w676:dbl[])
                          }
                          frame #2 {
                            n657 = Replace Array Subset(array=w692, new element=1 ("Neues Element/Teil-Array"), index=2 ("Index")) -> (w693:i32[])
                            n658 = Replace Array Subset(array=w689, new element=0.0 ("Neues Element/Teil-Array"), index=2 ("Index")) -> (w688:dbl[])
                          }
                          frame #3 {
                            n659 = Replace Array Subset(array=w701, new element=1 ("Neues Element/Teil-Array"), index=0 ("Index")) -> (w700:i32[])
                            n660 = Replace Array Subset(array=w697, new element=0.0 ("Neues Element/Teil-Array"), index=0 ("Index")) -> (w696:dbl[])
                          }
                          frame #4 {
                            n661 = Replace Array Subset(array=w707, new element=1 ("Neues Element/Teil-Array"), index=1 ("Index")) -> (w704:i32[])
                            n662 = Replace Array Subset(array=w706, new element=0.0 ("Neues Element/Teil-Array"), index=1 ("Index")) -> (w705:dbl[])
                          }
                        }
                        n663 = property class="Ring (strikt)"(reference=w657) -> ("RingText.Text"=w656:string)  [unwired: 1 in, 2 out]
                        n664 = local read "# Bilder/Messschritt"() -> (w655:i32)
                        n665 = control-ref of="Rasterart"() -> (w658:refnum<vi>)
                        n666 = Decimal String To Number(string=w656) -> (number=w653:i32)  [unwired: 2 in, 1 out]
                        n667 = local read "Suppressor-Spannung [V]"() -> (w642:dbl)
                        n668 = local read "P-Schirm-Spannung [V]"() -> (w647:dbl)
                        n669 = property class="Enum (strikt)"(reference=w658) -> ("RingText.Text"=w644:string)  [unwired: 1 in, 2 out]
                        n670 = local read "MCP-Spannung [V]"() -> (w646:dbl)
                        n671 = local read "Leistung (iK) [mW]"() -> (w645:dbl)
                        n672 = local read "Tip-Spannung [V]"() -> (w641:dbl)
                        n673 = local read "Polarisation [°]"() -> (w650:dbl)
                        n674 = Multiply(x=w655, y=w653) -> (x*y=w654:i32)
                        n675 = local read "Messlogbuch"() -> (w652:path)
                        n676 = local read "Proben-ID"() -> (w651:string)
                        n677 = local read "ROI"() -> (w643:i32[])
                        n678 = local write "# Rasterschritte"(w661) -> ()
                        n679 = local write "Rasterweite [µm]"(w659) -> ()
                        n680 = call "stage_get_current_xyz.vi"() -> ("Aktuelle xyz-Position OUT [mm]"=w648:dbl[])  [unwired: 3 in, 1 out]
                        n681 = call "create_measure_log_entry.vi"("Messlogbuch-Pfad"=w652, "Probe"=w651, "Polarisation [°]"=w650, "Messart"=w644, "ROI"=w643, "Messungen/Messschritt"=w655, "Maximalleistung (iK) [mW]"=w645, "Tip-Spannung [V]"=w641, "Suppressor-Spannung [V]"=w642, "Zeit/Messschritt [ms]"=w653, "MCP-Spannung [V]"=w646, "Zeit/Messung [ms]"=w654, "Phosphorschirm-Spannung [V]"=w647, "xyz [mm]"=w648) -> ("Messung Nr."=w649:i32)  [unwired: 4 in, 1 out]
                      }
                      frame #1 {
                        n682 = local write "Aktueller Messschritt"(0 ("Aktueller Messschritt")) -> ()
                        n683 = local read "Rasterweite [µm]"() -> (w743:dbl[])
                        n684 = local read "Fehler (Ausgang)"() -> (w718:errorcluster)
                        n685 = local read "# Rasterschritte"() -> (w742:i32[])
                        n686 = local read "# Rasterschritte"() -> (w740:i32[])
                        n687 = local read "Day folder"() -> (w723:string)
                        n688 = Divide(x=w743, y=w742) -> (x/y=w741:dbl[])
                        n689 = local read "Summierte Helligkeit speichern"() -> (w715:bool)
                        n690 = Index Array(array=w740, index #1=0 ("Index"), index #2=1 ("Index"), index #3=2 ("Index")) -> (element #1=w737:i32, element #2=w736:i32, element #3=w735:i32)
                        n691 = local read "Gemittelte Bilder speichern"() -> (w713:bool)
                        n692 = local read "LAPD-Daten speichern"() -> (w712:bool)
                        n693 = local read "Einzelbilder speichern"() -> (w714:bool)
                        n694 = local read "Einzelbilder speichern"() -> (w726:bool)
                        n695 = local write "Rasterschritt [µm]"(w741) -> ()
                        n696 = call "create_save_folder.vi"("Day folder"=w723, "Measuring number"=w717, "Measuring folder"="Rasterung" ("Subfolder"), "error in"=w718) -> ("Save Folder"=w722:string, "Error Out"=w721:errorcluster)  [unwired: 5 in]
                        n697 = Multiply(x=w737, y=w736) -> (x*y=w734:i32)
                        n698 = local write "Save folder"(w722) -> ()
                        n699 = case shown="True" w726 {
                          tunnel: w721 -> [w744 w746]
                          tunnel: [w744 w745] -> w720
                          frame #0 {
                          }
                          frame #1 {
                            n700 = local read "Save folder"() -> (w749:string)
                            n701 = Concatenate Strings(w749, "\\Einzelbilder" ("Subfolder")) -> (w747:string)
                            n702 = String To Path(string=w747) -> (path=w750:path)
                            n703 = call <vilib>:"Check if File or Folder Exists.vi"("error in (no error)"=w746, "path"=w750) -> ("error out"=w745:errorcluster, "file or folder exists?"=w751:bool, "dup path"=w752:path)  [unwired: 7 in]
                            n704 = case shown="False" w751 {
                              tunnel: w752 -> [w753 _]
                              frame #0 {
                                n705 = Create Folder(path (use dialog)=w753) -> ()  [unwired: 2 in, 3 out]
                              }
                              frame #1 {
                              }
                            }
                          }
                        }
                        n706 = Compound Arithmetic op=OR(w713, w714, w715, w712) -> (w716:bool)
                        n707 = Multiply(x=w734, y=w735) -> (x*y=w733:i32)
                        n708 = local write "Daten speichern"(w716) -> ()
                        n709 = local write "# Messschritte"(w733) -> ()
                        n710 = local read "Gemittelte Bilder speichern"() -> (w727:bool)
                        n711 = case shown="True" w727 {
                          tunnel: w720 -> [w754 w756]
                          tunnel: [w754 w755] -> w719
                          frame #0 {
                          }
                          frame #1 {
                            n712 = local read "Save folder"() -> (w760:string)
                            n713 = Concatenate Strings(w760, "\\Gemittelte Bilder" ("Subfolder")) -> (w762:string)
                            n714 = String To Path(string=w762) -> (path=w759:path)
                            n715 = call <vilib>:"Check if File or Folder Exists.vi"("error in (no error)"=w756, "path"=w759) -> ("error out"=w755:errorcluster, "file or folder exists?"=w758:bool, "dup path"=w757:path)  [unwired: 7 in]
                            n716 = case shown="False" w758 {
                              tunnel: w757 -> [w763 _]
                              frame #0 {
                                n717 = Create Folder(path (use dialog)=w763) -> ()  [unwired: 2 in, 3 out]
                              }
                              frame #1 {
                              }
                            }
                          }
                        }
                        n718 = local read "Kamera"() -> (w729:bool)
                        n719 = case shown="True" w729 {
                          tunnel: [w764 w766] -> w728
                          tunnel: w719 -> [w764 w765]
                          frame #0 {
                          }
                          frame #1 {
                            n720 = local read "Ereignis: FrameDone?"() -> (w767:refnum<event-registration>)
                            n721 = local read "Detektionskamera"() -> (w768:T5)
                            n722 = call "camera_release_configuration.vi"("error in"=w765, "Session In"=w768, "Ereignisregistrierung (Referenz) 2"=w767) -> ("error out"=w766:errorcluster)  [unwired: 1 out]
                          }
                        }
                        n723 = call "stage_get_current_xyz.vi"("error in"=w728) -> ("error out"=w725:errorcluster, "Aktuelle xyz-Position OUT [mm]"=w730:dbl[])  [unwired: 2 in]
                        n724 = local write "Start xyz-Position [mm]"(w730) -> ()
                        n725 = local write "Fehler (Ausgang)"(w725) -> ()
                      }
                    }
                  }
                  frame #1 {
                    n726 = flat-sequence {
                      tunnel: [w783] -> w779
                      tunnel: [w782] -> w778
                      tunnel: [w781] -> w777
                      tunnel: [w781] -> w776
                      tunnel: [w781] -> w775
                      tunnel: [w781] -> w774
                      tunnel: [w781] -> w773
                      tunnel: [w780] -> w772
                      tunnel: [w781] -> w771
                      tunnel: [w781] -> w770
                      tunnel: [w780] -> w769
                      tunnel: w779 -> [w797]
                      tunnel: w778 -> [w807]
                      tunnel: w777 -> [w806]
                      tunnel: w776 -> [w805]
                      tunnel: w775 -> [w804]
                      tunnel: w774 -> [w803]
                      tunnel: w773 -> [w802]
                      tunnel: w772 -> [w801]
                      tunnel: w771 -> [w800]
                      tunnel: w770 -> [w799]
                      tunnel: w769 -> [w798]
                      frame #0 {
                        n727 = local read "Rasterart"() -> (w784:T2)
                        n728 = case shown="\"2D-Scan(yz)\"" w784 {
                          tunnel: [0 ("Index") 2 ("Index") 0 ("Index")] -> w780
                          tunnel: [1 ("Index") 1 ("Index") 2 ("Index")] -> w781
                          tunnel: ["x-Position [mm]" ("X-Achse.Namensbeschriftung.Text") "z-Position [mm]" ("Y-Achse.Namensbeschriftung.Text") "x-Position [mm]" ("Y-Achse.Namensbeschriftung.Text")] -> w783
                          tunnel: ["y-Position [mm]" ("Y-Achse.Namensbeschriftung.Text") "y-Position [mm]" ("X-Achse.Namensbeschriftung.Text") "z-Position [mm]" ("X-Achse.Namensbeschriftung.Text")] -> w782
                          frame #0 {
                          }
                          frame #1 {
                          }
                          frame #2 {
                          }
                        }
                      }
                      frame #1 {
                        w815 = 1000.0 ("y")
                        w834 = 1000.0 ("y")
                        n729 = local read "Rasterweite [µm]"() -> (w839:dbl[])
                        n730 = local read "Rasterweite [µm]"() -> (w810:dbl[])
                        n731 = local read "# Rasterschritte"() -> (w843:i32[])
                        n732 = local read "# Rasterschritte"() -> (w832:i32[])
                        n733 = local read "# Rasterschritte"() -> (w817:i32[])
                        n734 = local read "Start xyz-Position [mm]"() -> (w838:dbl[])
                        n735 = local read "Start xyz-Position [mm]"() -> (w811:dbl[])
                        n736 = Index Array(array=w843, index #1=w801, index #2=w806) -> (element #1=w841:i32, element #2=w842:i32)
                        n737 = Index Array(array=w839, index #1=w801, index #2=w800) -> (element #1=w835:dbl, element #2=w836:dbl)
                        n738 = Index Array(array=w832, index #1=w801, index #2=w805) -> (element #1=w828:i32, element #2=w830:i32)
                        n739 = Index Array(array=w810, index #1=w801, index #2=w802) -> (element #1=w814:dbl, element #2=w813:dbl)
                        n740 = Index Array(array=w817, index #1=w801, index #2=w804) -> (element #1=w821:i32, element #2=w819:i32)
                        n741 = Divide(x=w835, y=w834) -> (x/y=w829:dbl)
                        n742 = Divide(x=w836, y=w834) -> (x/y=w831:dbl)
                        n743 = Divide(x=w814, y=w815) -> (x/y=w820:dbl)
                        n744 = Divide(x=w813, y=w815) -> (x/y=w818:dbl)
                        n745 = Index Array(array=w838, index #1=w798, index #2=w799) -> (element #1=w837:dbl, element #2=w833:dbl)
                        n746 = Index Array(array=w811, index #1=w801, index #2=w803) -> (element #1=w812:dbl, element #2=w816:dbl)
                        n747 = control-ref of="2D-Intensitätsverteilung (MCP)"() -> (w840:refnum<vi>)
                        n748 = Initialize Array(0.0 ("y"), w841, w842) -> (w824:dbl[][])
                        n749 = Divide(x=w820, y=w821) -> (x/y=w822:dbl)
                        n750 = Divide(x=w818, y=w819) -> (x/y=w823:dbl)
                        n751 = Divide(x=w829, y=w828) -> (x/y=w827:dbl)
                        n752 = Divide(x=w831, y=w830) -> (x/y=w826:dbl)
                        n753 = local write "2D-Intensitätsverteilung (LAPD)"(w824) -> ()
                        n754 = local write "2D-Intensitätsverteilung (MCP)"(w824) -> ()
                        n755 = property class="IntGraph (strikt)"(reference=w840, "XScale.Offset"=w837, "XScale.Multiplier"=w827, "YScale.Offset"=w833, "YScale.Multiplier"=w826, "XScale.MinorInc"=w827, "YScale.MinorInc"=w826, "XScale.NameLbl.Text"=w797, "YScale.NameLbl.Text"=w807) -> (error out=w844:errorcluster)  [unwired: 1 in, 1 out]
                        n756 = control-ref of="2D-Intensitätsverteilung (LAPD)"() -> (w808:refnum<vi>)
                        n757 = property class="IntGraph (strikt)"(reference=w808, error in=w844, "XScale.Offset"=w812, "XScale.Multiplier"=w822, "YScale.Offset"=w816, "YScale.Multiplier"=w823, "XScale.MinorInc"=w822, "YScale.MinorInc"=w823, "XScale.NameLbl.Text"=w797, "YScale.NameLbl.Text"=w807) -> (error out=w809:errorcluster)  [unwired: 1 out]
                        n758 = local write "Fehler (Ausgang)"(w809) -> ()
                      }
                    }
                  }
                  frame #2 {
                    n759 = local write "Rasterung läuft"(TRUE ("x-Linsescan")) -> ()
                    n760 = local read "Event: Rasterung gestartet?"() -> (w848:refnum<user-event>)
                    n761 = local read "Aktueller Messschritt"() -> (w847:i32)
                    n762 = Generate User Event(user event=w848, event data cluster=w847) -> (user event out=w846:refnum<user-event>)  [unwired: 1 in, 1 out]
                    n763 = local write "Event: Rasterung gestartet?"(w846) -> ()
                  }
                }
              }
            }
          }
          event #2 {
            n764 = event-data() -> ()  [unwired: 1 in, 1 out]
            n765 = local read "Rasterweite [µm]"() -> (w850:dbl[])
            n766 = local read "# Rasterschritte"() -> (w861:i32[])
            n767 = Replace Array Subset(array=w861, new element #1=1 ("Neues Element/Teil-Array"), index #1=0 ("Index"), new element #2=1 ("Neues Element/Teil-Array"), index #2=1 ("Index"), new element #3=1 ("Neues Element/Teil-Array"), index #3=2 ("Index")) -> (w857:i32[])
            n768 = Replace Array Subset(array=w850, new element #1=0 ("Neues Element/Teil-Array"), index #1=0 ("Index"), new element #2=0 ("Neues Element/Teil-Array"), index #2=1 ("Index"), new element #3=0 ("Neues Element/Teil-Array"), index #3=2 ("Index")) -> (w849:dbl[])
            n769 = local write "# Rasterschritte"(w857) -> ()
            n770 = local write "Rasterweite [µm]"(w849) -> ()
          }
          event #3 {
            n771 = event-data() -> ()  [unwired: 1 in, 1 out]
            n772 = stacked-sequence {
              frame #0 {
                n773 = while "x-Schleife" {
                  i -> [w867]
                  stop <- w868 stop-if-true
                  n774 = stacked-sequence {
                    frame #0 {
                      n775 = while "z-Schleife" {
                        i -> [w875]
                        stop <- w877 stop-if-true
                        n776 = stacked-sequence {
                          frame #0 {
                            n777 = while "y-Schleife" {
                              i -> [w886]
                              stop <- w892 stop-if-true
                              # "Schleife für y-Achse"
                              n778 = stacked-sequence {
                                frame #0 {
                                # "Hier findet die Messung statt"
                                n779 = stacked-sequence {
                                frame #0 {
                                n780 = local write "LAPD Spannung (V)"(0.0 ("Transmittierte Intensität (a.u.)")) -> ()
                                n781 = local write "Summierte Helligkeit (a.u.)"(u64 0 ("Summierte Helligkeit (a.u.)")) -> ()
                                n782 = local read "ROI"() -> (w899:i32[])
                                n783 = Index Array(array=w899, index #1=0 ("Index"), index #2=1 ("Index")) -> (element #1=w895:i32, element #2=w896:i32)
                                n784 = local read "Aktueller Messschritt"() -> (w902:i32)
                                n785 = Initialize Array(u64 0 ("Element"), w896, w895) -> (w901:u64[][])
                                n786 = local write "Gemitteltes Bild"(w901) -> ()
                                n787 = Increment(x=w902) -> (x+1=w903:i32)
                                n788 = local write "Aktueller Messschritt"(w903) -> ()
                                }
                                frame #1 {
                                n789 = local read "# Photosignale"() -> (w913:i32)
                                n790 = local read "# Bilder/Messschritt"() -> (w909:i32)
                                n791 = local read "Detektionskamera"() -> (w912:T5)
                                n792 = for {
                                N: w913 -> [_]
                                n793 = Wait (ms)(milliseconds to wait=u32 10 ("Zu wartende ms")) -> ()  [unwired: 1 out]
                                n794 = local read "LAPD-Kanal (Meilhaus)"() -> (w931:u32)
                                n795 = local read "LAPD Spannung (V)"() -> (w929:dbl)
                                n796 = call "AISingle.vi"("Time Out"=u32 0, "Channel Number"=w931, "Board Number"=u32 0) -> ("Analog Input Voltage"=w930:dbl)
                                n797 = Add(x=w930, y=w929) -> (x+y=w928:dbl)
                                n798 = local write "LAPD Spannung (V)"(w928) -> ()
                                }
                                n799 = local read "Einzelbilder speichern"() -> (w907:bool)
                                n800 = call "camera_acquisition_sequence.vi"("Session In"=w912, "Desired image number"=w909) -> ("Image Array"=w906:T4[], "error out"=w911:errorcluster)  [unwired: 2 in, 1 out]
                                n801 = case shown="True" w907 {
                                tunnel: w911 -> [w915 w923]
                                tunnel: [w915 w922] -> w910
                                tunnel: w909 -> [w914 w921]
                                tunnel: [w914 w921] -> w908
                                tunnel: w906 -> [_ w920]
                                frame #0 {
                                }
                                frame #1 {
                                n802 = local read "Aktueller Messschritt"() -> (w926:i32)
                                n803 = local read "Save folder"() -> (w918:string)
                                n804 = Concatenate Strings(w918, "Einzelbilder\\" ("String")) -> (w916:string)
                                n805 = Format Into String(format string="%05.0f" ("Format-String"), initial string="#" ("Eingangs-String"), w926) -> (resulting string=w919:string)  [unwired: 1 in, 1 out]
                                n806 = call "save images.vi"("Save Folder"=w916, "File name prefix"=w919, "Array"=w920, "error out 2"=w923, "Bilder/Messschritt"=w921) -> ("error out"=w922:errorcluster)
                                }
                                }
                                n807 = for {
                                N: w908 -> [_]
                                tunnel: w910 -> [w939]
                                tunnel: w906 -> [w937] mode=indexing
                                n808 = call "IMAQ ImageToArray"("error in (no error)"=w939, "Image"=w937) -> ("error out"=w938:errorcluster, "Image Pixels (U8)"=w936:u8[][])  [unwired: 2 in, 3 out]
                                n809 = To Unsigned Quad Integer(1:w936) -> (0:w941:u64[][])
                                n810 = local write "Fehler (Ausgang)"(w938) -> ()
                                n811 = local read "Gemitteltes Bild"() -> (w934:u64[][])
                                n812 = Add Array Elements(numeric array=w941) -> (sum=w940:u64)
                                n813 = local read "Summierte Helligkeit (a.u.)"() -> (w942:u64)
                                n814 = Add(x=w934, y=w936) -> (x+y=w935:u64[][])
                                n815 = local write "Gemitteltes Bild"(w935) -> ()
                                n816 = Add(x=w940, y=w942) -> (x+y=w943:u64)
                                n817 = local write "Summierte Helligkeit (a.u.)"(w943) -> ()
                                }
                                }
                                frame #2 {
                                n818 = local read "Rasterart"() -> (w953:T2)
                                n819 = case shown="\"2D-Scan(xz)\"" w953 {
                                tunnel: [w975 w976 w978 w979 w981] -> w952
                                tunnel: [w974 w977 w978 w979 w980] -> w951
                                frame #0 {
                                n820 = local read "Current x step"() -> (w975:i32)
                                n821 = local read "Current y step"() -> (w974:i32)
                                }
                                frame #1 {
                                n822 = local read "Current z step"() -> (w976:i32)
                                n823 = local read "Current y step"() -> (w977:i32)
                                }
                                frame #2 {
                                n824 = local read "Current z step"() -> (w978:i32)
                                }
                                frame #3 {
                                n825 = local read "Current x step"() -> (w979:i32)
                                }
                                frame #4 {
                                n826 = local read "Current x step"() -> (w981:i32)
                                n827 = local read "Current z step"() -> (w980:i32)
                                }
                                }
                                n828 = local read "# Bilder/Messschritt"() -> (w948:i32)
                                n829 = local read "Gemitteltes Bild"() -> (w950:u64[][])
                                n830 = local read "LAPD Spannung (V)"() -> (w959:dbl)
                                n831 = local read "# Photosignale"() -> (w958:i32)
                                n832 = local read "Image Display"() -> (w946:T4)
                                n833 = Divide(x=w950, y=w948) -> (x/y=w949:dbl[][])
                                n834 = local read "2D-Intensitätsverteilung (LAPD)"() -> (w954:dbl[][])
                                n835 = local read "2D-Intensitätsverteilung (MCP)"() -> (w955:dbl[][])
                                n836 = local read "Gemittelte Bilder speichern"() -> (w944:bool)
                                n837 = local read "Summierte Helligkeit (a.u.)"() -> (w960:u64)
                                n838 = Divide(x=w959, y=w958) -> (x/y=w956:dbl)
                                n839 = call "IMAQ ArrayToImage"("Image Pixels (U8)"=w949, "Image"=w946) -> ("Image Out"=w947:T4)  [unwired: 8 in, 1 out]
                                n840 = Replace Array Subset(array=w955, new element=w960, index (row)=w952, index (col)=w951) -> (w961:dbl[][])
                                n841 = local write "LAPD Spannung (V)"(w956) -> ()
                                n842 = Replace Array Subset(array=w954, new element=w956, index (row)=w952, index (col)=w951) -> (w957:dbl[][])
                                n843 = case shown="True" w944 {
                                tunnel: w947 -> [w962 w973]
                                tunnel: [w962 w964] -> w945
                                frame #0 {
                                }
                                frame #1 {
                                n844 = local read "Aktueller Messschritt"() -> (w968:i32)
                                n845 = local read "Save folder"() -> (w970:string)
                                n846 = Format Into String(format string="%05.0f" ("Format-String"), initial string="#" ("Eingangs-String"), w968) -> (resulting string=w967:string)  [unwired: 1 in, 1 out]
                                n847 = Concatenate Strings(w970, "Gemittelte Bilder\\" ("String"), w967, ".png" ("String")) -> (w966:string)
                                n848 = String To Path(string=w966) -> (path=w965:path)
                                n849 = call-poly "IMAQ Write File 2"("File Path"=w965, "Image"=w973) -> ("Image Out (duplicate)"=w964:T4)  [unwired: 8 in, 1 out]
                                }
                                }
                                n850 = local write "2D-Intensitätsverteilung (MCP)"(w961) -> ()
                                n851 = local write "2D-Intensitätsverteilung (LAPD)"(w957) -> ()
                                n852 = local write "Image Display"(w945) -> ()
                                }
                                }
                                }
                                frame #1 {
                                n853 = local read "y-Achse"() -> (w987:i32)
                                n854 = local read "Aktueller Messschritt"() -> (w984:i32)
                                n855 = local read "Rasterschritt [µm]"() -> (w991:dbl[])
                                n856 = local read "Start time [ms]"() -> (w985:timestamp)
                                n857 = local read "# Messschritte"() -> (w983:i32)
                                n858 = Decrement(x=w987) -> (x-1=w990:i32)
                                n859 = Index Array(array=w991, index=w990) -> (element=w986:dbl)
                                n860 = call "estimate_stopp_time.vi"("Aktueller Messschritt"=w984, "# Messschritte"=w983, "Startzeit"=w985) -> ("Stopp Zeit"=w982:string)  [unwired: 8 in]
                                n861 = local write "Geschätzte Messzeit"(w982) -> ()
                                n862 = Not Equal?(x=w986, y=0.0) -> (x != y?=w988:bool)
                                n863 = case shown="True" w988 {
                                tunnel: w987 -> [_ w993]
                                tunnel: w986 -> [_ w992]
                                frame #0 {
                                }
                                frame #1 {
                                # "Fahre nächste y-Position an"
                                n864 = call "stage_move_axis_relative.vi"("Achse"=w993, "Schrittweite [µm]"=w992) -> ("error out"=w995:errorcluster, "xyz-Position OUT [mm]"=w994:dbl[])  [unwired: 1 in, 1 out]
                                n865 = local write "Aktuelle xyz-Position [mm]"(w994) -> ()
                                n866 = local write "Fehler (Ausgang)"(w995) -> ()
                                }
                                }
                                }
                              }
                              n867 = local read "y-Achse"() -> (w885:i32)
                              n868 = local read "# Rasterschritte"() -> (w891:i32[])
                              n869 = Decrement(x=w885) -> (x-1=w887:i32)
                              n870 = local read "Rasterung ON/OFF"() -> (w893:bool)
                              n871 = Increment(x=w886) -> (x+1=w888:i32)
                              n872 = Index Array(array=w891, index=w887) -> (element=w890:i32)
                              n873 = Equal?(x=w890, y=w888) -> (x = y?=w889:bool)
                              n874 = Not(x=w893) -> (.not. x?=w894:bool)
                              n875 = Or(x=w889, y=w894) -> (x .or. y?=w892:bool)
                              "Current y step" <- w886
                            }
                          }
                          frame #1 {
                            n876 = flat-sequence {
                              frame #0 {
                                n877 = local read "y-Achse"() -> (w997:i32)
                                n878 = local read "Rasterschritt [µm]"() -> (w1002:dbl[])
                                n879 = Decrement(x=w997) -> (x-1=w1001:i32)
                                n880 = local read "Start xyz-Position [mm]"() -> (w996:dbl[])
                                n881 = Index Array(array=w1002, index=w1001) -> (element=w1000:dbl)
                                n882 = Not Equal?(x=w1000, y=0.0) -> (x != y?=w998:bool)
                                n883 = case shown="True" w998 {
                                tunnel: w997 -> [_ w1004]
                                tunnel: w996 -> [_ w1003]
                                frame #0 {
                                }
                                frame #1 {
                                # "Fahre Startposition für y an"
                                n884 = call "stage_move_axis_absolute.vi"("Ziel xyz IN [mm]"=w1003, "Achse"=w1004) -> ("error out"=w1006:errorcluster, "Ziel xyz OUT [mm]"=w1005:dbl[])  [unwired: 1 in, 1 out]
                                n885 = local write "Aktuelle xyz-Position [mm]"(w1005) -> ()
                                n886 = local write "Fehler (Ausgang)"(w1006) -> ()
                                }
                                }
                              }
                              frame #1 {
                                n887 = local read "Rasterschritt [µm]"() -> (w1012:dbl[])
                                n888 = local read "z-Achse"() -> (w1007:i32)
                                n889 = Decrement(x=w1007) -> (x-1=w1008:i32)
                                n890 = Index Array(array=w1012, index=w1008) -> (element=w1009:dbl)
                                n891 = Not Equal?(x=w1009, y=0.0) -> (x != y?=w1010:bool)
                                n892 = case shown="True" w1010 {
                                tunnel: w1009 -> [_ w1014]
                                tunnel: w1007 -> [_ w1013]
                                frame #0 {
                                }
                                frame #1 {
                                # "Fahre nächste Position für z an"
                                n893 = call "stage_move_axis_relative.vi"("Achse"=w1013, "Schrittweite [µm]"=w1014) -> ("error out"=w1015:errorcluster, "xyz-Position OUT [mm]"=w1016:dbl[])  [unwired: 1 in, 1 out]
                                n894 = local write "Aktuelle xyz-Position [mm]"(w1016) -> ()
                                n895 = local write "Fehler (Ausgang)"(w1015) -> ()
                                }
                                }
                              }
                            }
                          }
                        }
                        n896 = local read "z-Achse"() -> (w876:i32)
                        n897 = local read "# Rasterschritte"() -> (w880:i32[])
                        n898 = Decrement(x=w876) -> (x-1=w884:i32)
                        n899 = local read "Rasterung ON/OFF"() -> (w879:bool)
                        n900 = Increment(x=w875) -> (x+1=w883:i32)
                        n901 = Index Array(array=w880, index=w884) -> (element=w881:i32)
                        n902 = Equal?(x=w881, y=w883) -> (x = y?=w882:bool)
                        n903 = Not(x=w879) -> (.not. x?=w878:bool)
                        n904 = Or(x=w882, y=w878) -> (x .or. y?=w877:bool)
                        "Current z step" <- w875
                      }
                    }
                    frame #1 {
                      n905 = flat-sequence {
                        frame #0 {
                          n906 = local read "z-Achse"() -> (w1017:i32)
                          n907 = local read "Rasterschritt [µm]"() -> (w1020:dbl[])
                          n908 = Decrement(x=w1017) -> (x-1=w1021:i32)
                          n909 = local read "Start xyz-Position [mm]"() -> (w1018:dbl[])
                          n910 = Index Array(array=w1020, index=w1021) -> (element=w1022:dbl)
                          n911 = Not Equal?(x=w1022, y=0.0) -> (x != y?=w1019:bool)
                          n912 = case shown="True" w1019 {
                            tunnel: w1018 -> [_ w1025]
                            tunnel: w1017 -> [_ w1024]
                            frame #0 {
                            }
                            frame #1 {
                              # "Fahre Startposition für z an"
                              n913 = call "stage_move_axis_absolute.vi"("Ziel xyz IN [mm]"=w1025, "Achse"=w1024) -> ("error out"=w1026:errorcluster, "Ziel xyz OUT [mm]"=w1027:dbl[])  [unwired: 1 in, 1 out]
                              n914 = local write "Aktuelle xyz-Position [mm]"(w1027) -> ()
                              n915 = local write "Fehler (Ausgang)"(w1026) -> ()
                            }
                          }
                        }
                        frame #1 {
                          n916 = local read "Rasterschritt [µm]"() -> (w1033:dbl[])
                          n917 = local read "x-Achse"() -> (w1028:i32)
                          n918 = Decrement(x=w1028) -> (x-1=w1032:i32)
                          n919 = Index Array(array=w1033, index=w1032) -> (element=w1031:dbl)
                          n920 = Not Equal?(x=w1031, y=0.0) -> (x != y?=w1029:bool)
                          n921 = case shown="True" w1029 {
                            tunnel: w1031 -> [_ w1036]
                            tunnel: w1028 -> [_ w1034]
                            frame #0 {
                            }
                            frame #1 {
                              # "Fahre nächste Position für x an"
                              n922 = call "stage_move_axis_relative.vi"("Achse"=w1034, "Schrittweite [µm]"=w1036) -> ("error out"=w1037:errorcluster, "xyz-Position OUT [mm]"=w1035:dbl[])  [unwired: 1 in, 1 out]
                              n923 = local write "Aktuelle xyz-Position [mm]"(w1035) -> ()
                              n924 = local write "Fehler (Ausgang)"(w1037) -> ()
                            }
                          }
                        }
                      }
                    }
                  }
                  n925 = local read "# Rasterschritte"() -> (w865:i32[])
                  n926 = local read "x-Achse"() -> (w866:i32)
                  n927 = Decrement(x=w866) -> (x-1=w869:i32)
                  n928 = local read "Rasterung ON/OFF"() -> (w873:bool)
                  n929 = Increment(x=w867) -> (x+1=w870:i32)
                  n930 = Index Array(array=w865, index=w869) -> (element=w872:i32)
                  n931 = Equal?(x=w872, y=w870) -> (x = y?=w871:bool)
                  n932 = Not(x=w873) -> (.not. x?=w874:bool)
                  n933 = Or(x=w871, y=w874) -> (x .or. y?=w868:bool)
                  "Current x step" <- w867
                }
              }
              frame #1 {
                n934 = flat-sequence {
                  frame #0 {
                    # "Zur Ausgangsposition zurückfahren"
                    n935 = local read "Start xyz-Position [mm]"() -> (w1128:dbl[])
                    n936 = local read "Detektionskamera"() -> (w1118:T5)
                    n937 = local read "Buffer Interval"() -> (w1117:u32)
                    n938 = call "camera_create_configuration.vi"("BufferInterval"=w1117, "Session Out 2"=w1118) -> ("Fehler (Ausgang)"=w1116:errorcluster, "Ereignisregistrierung (Referenz)"=w1119:refnum<event-registration>)  [unwired: 1 in, 1 out]
                    n939 = local write "Ereignis: FrameDone?"(w1119) -> ()
                    n940 = local read "x-Achse"() -> (w1125:i32)
                    n941 = call "stage_move_axis_absolute.vi"("error in"=w1116, "Ziel xyz IN [mm]"=w1128, "Achse"=w1125) -> ("error out"=w1121:errorcluster)  [unwired: 2 out]
                    n942 = local read "y-Achse"() -> (w1126:i32)
                    n943 = call "stage_move_axis_absolute.vi"("error in"=w1121, "Ziel xyz IN [mm]"=w1128, "Achse"=w1126) -> ("error out"=w1122:errorcluster)  [unwired: 2 out]
                    n944 = local read "z-Achse"() -> (w1127:i32)
                    n945 = call "stage_move_axis_absolute.vi"("error in"=w1122, "Ziel xyz IN [mm]"=w1128, "Achse"=w1127) -> ("error out"=w1123:errorcluster, "Fertig?"=w1124:bool, "Ziel xyz OUT [mm]"=w1129:dbl[])
                    n946 = Not(x=w1124) -> (.not. x?=w1120:bool)
                    n947 = local write "Aktuelle xyz-Position [mm]"(w1129) -> ()
                    n948 = local write "Fehler (Ausgang)"(w1123) -> ()
                    n949 = local write "Rasterung ON/OFF"(w1120) -> ()
                    n950 = local write "Rasterung läuft"(w1120) -> ()
                  }
                }
                n951 = local read "Daten speichern"() -> (w1038:bool)
                n952 = local read "LAPD-Daten speichern"() -> (w1047:bool)
                n953 = local read "2D-Intensitätsverteilung (MCP)"() -> (w1046:dbl[][])
                n954 = local read "Summierte Helligkeit speichern"() -> (w1048:bool)
                n955 = case shown="True" w1038 {
                  frame #0 {
                  }
                  frame #1 {
                    n956 = local read "Rasterschritt [µm]"() -> (w1050:dbl[])
                    n957 = Divide(x=w1050, y=1000) -> (x/y=w1051:dbl[])
                    n958 = local read "Start xyz-Position [mm]"() -> (w1053:dbl[])
                    n959 = local read "# Rasterschritte"() -> (w1054:i32[])
                    n960 = local read "Save folder"() -> (w1052:string)
                    n961 = local read "Rasterart"() -> (w1055:T2)
                    n962 = case shown="\"2D-Scan(xz)\"" w1055 {
                      tunnel: w1054 -> [w1058 w1065 w1077 w1098 w1108]
                      tunnel: w1053 -> [w1056 w1067 w1075 w1099 w1110]
                      tunnel: w1052 -> [w1059 w1068 w1074 w1097 w1111]
                      tunnel: w1051 -> [w1057 w1066 w1076 w1088 w1109]
                      frame #0 {
                        w1064 = 0 ("Index")
                        n963 = Index Array(array=w1056, index=w1064) -> (element=w1062:dbl)
                        n964 = Index Array(array=w1057, index=w1064) -> (element=w1060:dbl)
                        n965 = Index Array(array=w1058, index=w1064) -> (element=w1061:i32)
                        n966 = call "create_axis_vector_file.vi"("Save folder"=w1059, "Dateiname"="xAchse.dat", "Start"=w1062, "Schrittlänge"=w1060, "# Schritte"=w1061) -> ()  [unwired: 11 in]
                      }
                      frame #1 {
                        w1073 = 2 ("Index")
                        n967 = Index Array(array=w1067, index=w1073) -> (element=w1071:dbl)
                        n968 = Index Array(array=w1066, index=w1073) -> (element=w1069:dbl)
                        n969 = Index Array(array=w1065, index=w1073) -> (element=w1070:i32)
                        n970 = call "create_axis_vector_file.vi"("Save folder"=w1068, "Dateiname"="xAchse.dat", "Start"=w1071, "Schrittlänge"=w1069, "# Schritte"=w1070) -> ()  [unwired: 11 in]
                      }
                      frame #2 {
                        w1086 = 1 ("Index")
                        w1087 = 0 ("Index")
                        n971 = Index Array(array=w1075, index #1=w1087, index #2=w1086) -> (element #1=w1083:dbl, element #2=w1080:dbl)
                        n972 = Index Array(array=w1076, index #1=w1087, index #2=w1086) -> (element #1=w1081:dbl, element #2=w1079:dbl)
                        n973 = Index Array(array=w1077, index #1=w1087, index #2=w1086) -> (element #1=w1082:i32, element #2=w1078:i32)
                        n974 = call "create_axis_vector_file.vi"("Save folder"=w1074, "Dateiname"="xAchse.dat", "Start"=w1083, "Schrittlänge"=w1081, "# Schritte"=w1082) -> ()  [unwired: 11 in]
                        n975 = call "create_axis_vector_file.vi"("Save folder"=w1074, "Dateiname"="yAchse.dat", "Start"=w1080, "Schrittlänge"=w1079, "# Schritte"=w1078) -> ()  [unwired: 11 in]
                      }
                      frame #3 {
                        w1100 = 2 ("Index")
                        w1101 = 1 ("Index")
                        n976 = Index Array(array=w1099, index #1=w1101, index #2=w1100) -> (element #1=w1094:dbl, element #2=w1091:dbl)
                        n977 = Index Array(array=w1088, index #1=w1101, index #2=w1100) -> (element #1=w1092:dbl, element #2=w1090:dbl)
                        n978 = Index Array(array=w1098, index #1=w1101, index #2=w1100) -> (element #1=w1093:i32, element #2=w1089:i32)
                        n979 = call "create_axis_vector_file.vi"("Save folder"=w1097, "Dateiname"="yAchse.dat", "Start"=w1094, "Schrittlänge"=w1092, "# Schritte"=w1093) -> ()  [unwired: 11 in]
                        n980 = call "create_axis_vector_file.vi"("Save folder"=w1097, "Dateiname"="xAchse.dat", "Start"=w1091, "Schrittlänge"=w1090, "# Schritte"=w1089) -> ()  [unwired: 11 in]
                      }
                      frame #4 {
                        w1114 = 2 ("Index")
                        w1115 = 0 ("Index")
                        n981 = Index Array(array=w1110, index #1=w1115, index #2=w1114) -> (element #1=w1107:dbl, element #2=w1102:dbl)
                        n982 = Index Array(array=w1109, index #1=w1115, index #2=w1114) -> (element #1=w1106:dbl, element #2=w1103:dbl)
                        n983 = Index Array(array=w1108, index #1=w1115, index #2=w1114) -> (element #1=w1105:i32, element #2=w1104:i32)
                        n984 = call "create_axis_vector_file.vi"("Save folder"=w1111, "Dateiname"="xAchse.dat", "Start"=w1107, "Schrittlänge"=w1106, "# Schritte"=w1105) -> ()  [unwired: 11 in]
                        n985 = call "create_axis_vector_file.vi"("Save folder"=w1111, "Dateiname"="yAchse.dat", "Start"=w1102, "Schrittlänge"=w1103, "# Schritte"=w1104) -> ()  [unwired: 11 in]
                      }
                    }
                  }
                }
                n986 = local read "2D-Intensitätsverteilung (LAPD)"() -> (w1042:dbl[][])
                n987 = case shown="True" w1047 {
                  frame #0 {
                  }
                  frame #1 {
                    n988 = local read "Save folder"() -> (w1134:string)
                    n989 = Concatenate Strings(w1134, "\\" ("String"), "2D_Intensitaetsverteilung_LAPD.dat" ("String")) -> (w1136:string)
                    n990 = local read "2D-Intensitätsverteilung (LAPD)"() -> (w1132:dbl[][])
                    n991 = String To Path(string=w1136) -> (path=w1135:path)
                    n992 = call-poly <vilib>:"Write To Spreadsheet File.vi"("format (%.3f)"="%.;%.5f", "2D data"=w1132, "file path (dialog if empty)"=w1135) -> ()  [unwired: 5 in, 1 out]
                  }
                }
                n993 = control-ref of="2D-Intensitätsverteilung (MCP)"() -> (w1045:refnum<vi>)
                n994 = case shown="True" w1048 {
                  frame #0 {
                  }
                  frame #1 {
                    n995 = local read "Save folder"() -> (w1140:string)
                    n996 = Concatenate Strings(w1140, "\\" ("String"), "2D_Intensitaetsverteilung_MCP.dat" ("String")) -> (w1138:string)
                    n997 = local read "2D-Intensitätsverteilung (MCP)"() -> (w1142:dbl[][])
                    n998 = String To Path(string=w1138) -> (path=w1139:path)
                    n999 = call-poly <vilib>:"Write To Spreadsheet File.vi"("format (%.3f)"="%.;%8.0f", "2D data"=w1142, "file path (dialog if empty)"=w1139) -> ()  [unwired: 5 in, 1 out]
                  }
                }
                n1000 = Array Max & Min(array=w1046) -> (max value=w1044:dbl, min value=w1043:dbl)  [unwired: 2 out]
                n1001 = control-ref of="2D-Intensitätsverteilung (LAPD)"() -> (w1039:refnum<vi>)
                n1002 = Array Max & Min(array=w1042) -> (max value=w1041:dbl, min value=w1040:dbl)  [unwired: 2 out]
                n1003 = property class="IntGraph (strikt)"(reference=w1045, "ZScale.Maximum"=w1044, "ZScale.Minimum"=w1043) -> ()  [unwired: 1 in, 2 out]
                n1004 = property class="IntGraph (strikt)"(reference=w1039, "ZScale.Maximum"=w1041, "ZScale.Minimum"=w1040) -> ()  [unwired: 1 in, 2 out]
              }
            }
          }
          event #4 {
            n1005 = event-data() -> ("NewVal"=w1145:bool)  [unwired: 1 in, 3 out]
            n1006 = local read "Wellenplatte"() -> (w1146:bool)
            n1007 = local read "Kamera"() -> (w1147:bool)
            n1008 = Compound Arithmetic op=AND(w1147, w1145, w1146) -> (w1144:bool)
            n1009 = case shown="True" w1144 {
              frame #0 {
                n1010 = local write "Leistungs-/Polarisationscan läuft"(FALSE ("Messung läuft")) -> ()
              }
              frame #1 {
                n1011 = stacked-sequence {
                  frame #0 {
                    n1012 = flat-sequence {
                      tunnel: [w1173] -> w1152
                      tunnel: [w1165] -> w1150
                      tunnel: w1152 -> [w1202]
                      tunnel: [w1202] -> w1151
                      tunnel: w1150 -> [w1201]
                      tunnel: [w1201] -> w1149
                      tunnel: w1151 -> [w1209]
                      tunnel: w1149 -> [w1208]
                      frame #0 {
                        n1013 = local read "Hin und Zurück"() -> (w1159:bool)
                        n1014 = Get Date/Time In Seconds() -> (seconds since 1Jan1904=w1168:timestamp)
                        n1015 = local read "# L/2-Schritte"() -> (w1158:i32)
                        n1016 = local read "L/2-Weite [°]"() -> (w1163:dbl)
                        n1017 = local write "Aktueller Messschritt"(0 ("Aktueller Messschritt")) -> ()
                        n1018 = local write "Start time [ms]"(w1168) -> ()
                        n1019 = local read "Leistuns- oder Polarisationsscan"() -> (w1166:u16)
                        n1020 = Divide(x=w1163, y=w1158) -> (x/y=w1162:dbl)
                        n1021 = case shown="False" w1159 {
                          tunnel: w1158 -> [w1185 w1190]
                          tunnel: [w1183 w1188] -> w1153
                          frame #0 {
                            n1022 = local write "Leist/Pol # Schleifen"(i64 1 ("Leist/Pol # Schleifen")) -> ()
                            n1023 = Increment(x=w1185) -> (x+1=w1183:i32)
                          }
                          frame #1 {
                            n1024 = local write "Leist/Pol # Schleifen"(i64 2 ("Leist/Pol # Schleifen")) -> ()
                            n1025 = Increment(x=w1190) -> (x+1=w1186:i32)
                            n1026 = Multiply(x=w1186, y=2) -> (x*y=w1188:i32)
                          }
                        }
                        n1027 = local write "L/2-Schritt [°]"(w1162) -> ()
                        n1028 = local read "L/2-Start [°]"() -> (w1160:dbl)
                        n1029 = case shown="1" w1166 {
                          tunnel: ["Polarisationsscan" ("Subfolder") "Leistungsscan" ("Subfolder")] -> w1165
                          tunnel: [w1191 w1197] -> w1164
                          tunnel: [w1192 w1194] -> w1161
                          tunnel: w1160 -> [w1191 w1196]
                          frame #0 {
                            n1030 = local read "Leistung (iK) [mW]"() -> (w1192:dbl)
                          }
                          frame #1 {
                            n1031 = local read "Max. Leistung (vK) [mW]"() -> (w1195:dbl)
                            n1032 = local read "Polarisation [°]"() -> (w1197:dbl)
                            n1033 = call "calculate_power_in_chamber.vi"("Aktuelle L/2 Position [°]"=w1196, "Eingestellte Polarisation [°]"=w1197, "Max. Leistung (vK) [mW]"=w1195) -> ("Aktuelle Leistung (iK) [mW]"=w1194:dbl)  [unwired: 8 in]
                            n1034 = local write "Leistung (iK) [mW]"(w1194) -> ()
                          }
                        }
                        n1035 = Initialize Array(0.0 ("Element"), w1153) -> (w1157:dbl[])
                        n1036 = Initialize Array(0.0 ("Element"), w1153) -> (w1156:dbl[])
                        n1037 = local write "# Messschritte"(w1153) -> ()
                        n1038 = local write "Vektor Summierte Helligkeit [a.u.]"(w1157) -> ()
                        n1039 = local write "Vektor L/2-Position [°]"(w1156) -> ()
                        n1040 = control-ref of="Shutter time (ms)"() -> (w1182:refnum<vi>)
                        n1041 = property class="Ring (strikt)"(reference=w1182) -> ("RingText.Text"=w1181:string)  [unwired: 1 in, 2 out]
                        n1042 = local read "# Bilder/Messschritt"() -> (w1174:i32)
                        n1043 = local read "Suppressor-Spannung [V]"() -> (w1170:dbl)
                        n1044 = local read "P-Schirm-Spannung [V]"() -> (w1172:dbl)
                        n1045 = local read "MCP-Spannung [V]"() -> (w1171:dbl)
                        n1046 = local read "Tip-Spannung [V]"() -> (w1169:dbl)
                        n1047 = local read "Messlogbuch"() -> (w1179:path)
                        n1048 = call "stage_get_current_xyz.vi"() -> ("Aktuelle xyz-Position OUT [mm]"=w1167:dbl[])  [unwired: 3 in, 1 out]
                        n1049 = Decimal String To Number(string=w1181) -> (number=w1175:i32)  [unwired: 2 in, 1 out]
                        n1050 = local read "Proben-ID"() -> (w1178:string)
                        n1051 = Multiply(x=w1174, y=w1175) -> (x*y=w1176:i32)
                        n1052 = local write "Start xyz-Position [mm]"(w1167) -> ()
                        n1053 = local read "ROI"() -> (w1177:i32[])
                        n1054 = call "create_measure_log_entry.vi"("Messlogbuch-Pfad"=w1179, "Probe"=w1178, "Polarisation [°]"=w1164, "Messart"=w1165, "ROI"=w1177, "Messungen/Messschritt"=w1174, "Maximalleistung (iK) [mW]"=w1161, "Tip-Spannung [V]"=w1169, "Suppressor-Spannung [V]"=w1170, "Zeit/Messschritt [ms]"=w1175, "MCP-Spannung [V]"=w1171, "Zeit/Messung [ms]"=w1176, "Phosphorschirm-Spannung [V]"=w1172, "xyz [mm]"=w1167) -> ("Messung Nr."=w1173:i32)  [unwired: 4 in, 1 out]
                      }
                      frame #1 {
                        n1055 = local read "# L/2-Schritte"() -> (w1200:i32)
                        n1056 = Increment(x=w1200) -> (x+1=w1199:i32)
                        n1057 = local write "# L/2-Schritte"(w1199) -> ()
                      }
                      frame #2 {
                        n1058 = local read "Fehler (Ausgang)"() -> (w1211:errorcluster)
                        n1059 = local read "Summierte Helligkeit speichern"() -> (w1204:bool)
                        n1060 = local read "Einzelbilder speichern"() -> (w1217:bool)
                        n1061 = local read "Gemittelte Bilder speichern"() -> (w1206:bool)
                        n1062 = local read "Day folder"() -> (w1216:string)
                        n1063 = local read "LAPD-Daten speichern"() -> (w1207:bool)
                        n1064 = local read "Einzelbilder speichern"() -> (w1205:bool)
                        n1065 = call "create_save_folder.vi"("Day folder"=w1216, "Measuring number"=w1209, "Measuring folder"=w1208, "error in"=w1211) -> ("Save Folder"=w1215:string, "Error Out"=w1214:errorcluster)  [unwired: 5 in]
                        n1066 = local write "Save folder"(w1215) -> ()
                        n1067 = case shown="True" w1217 {
                          tunnel: w1214 -> [w1220 w1222]
                          tunnel: [w1220 w1221] -> w1213
                          frame #0 {
                          }
                          frame #1 {
                            n1068 = local read "Save folder"() -> (w1225:string)
                            n1069 = Concatenate Strings(w1225, "\\Einzelbilder" ("Subfolder")) -> (w1223:string)
                            n1070 = String To Path(string=w1223) -> (path=w1226:path)
                            n1071 = call <vilib>:"Check if File or Folder Exists.vi"("error in (no error)"=w1222, "path"=w1226) -> ("error out"=w1221:errorcluster, "file or folder exists?"=w1227:bool, "dup path"=w1228:path)  [unwired: 7 in]
                            n1072 = case shown="False" w1227 {
                              tunnel: w1228 -> [w1229 _]
                              frame #0 {
                                n1073 = Create Folder(path (use dialog)=w1229) -> ()  [unwired: 2 in, 3 out]
                              }
                              frame #1 {
                              }
                            }
                          }
                        }
                        n1074 = Compound Arithmetic op=OR(w1206, w1205, w1204, w1207) -> (w1203:bool)
                        n1075 = local write "Daten speichern"(w1203) -> ()
                        n1076 = local read "Gemittelte Bilder speichern"() -> (w1218:bool)
                        n1077 = case shown="True" w1218 {
                          tunnel: w1213 -> [w1230 w1232]
                          tunnel: [w1230 w1231] -> w1212
                          frame #0 {
                          }
                          frame #1 {
                            n1078 = local read "Save folder"() -> (w1236:string)
                            n1079 = Concatenate Strings(w1236, "\\Gemittelte Bilder" ("Subfolder")) -> (w1238:string)
                            n1080 = String To Path(string=w1238) -> (path=w1235:path)
                            n1081 = call <vilib>:"Check if File or Folder Exists.vi"("error in (no error)"=w1232, "path"=w1235) -> ("error out"=w1231:errorcluster, "file or folder exists?"=w1234:bool, "dup path"=w1233:path)  [unwired: 7 in]
                            n1082 = case shown="False" w1234 {
                              tunnel: w1233 -> [w1239 _]
                              frame #0 {
                                n1083 = Create Folder(path (use dialog)=w1239) -> ()  [unwired: 2 in, 3 out]
                              }
                              frame #1 {
                              }
                            }
                          }
                        }
                        n1084 = local read "Kamera"() -> (w1219:bool)
                        n1085 = case shown="True" w1219 {
                          tunnel: [w1240 w1242] -> w1210
                          tunnel: w1212 -> [w1240 w1241]
                          frame #0 {
                          }
                          frame #1 {
                            n1086 = local read "Ereignis: FrameDone?"() -> (w1243:refnum<event-registration>)
                            n1087 = local read "Detektionskamera"() -> (w1244:T5)
                            n1088 = call "camera_release_configuration.vi"("error in"=w1241, "Session In"=w1244, "Ereignisregistrierung (Referenz) 2"=w1243) -> ("error out"=w1242:errorcluster)  [unwired: 1 out]
                          }
                        }
                        n1089 = local write "Fehler (Ausgang)"(w1210) -> ()
                      }
                    }
                  }
                  frame #1 {
                    n1090 = flat-sequence {
                      frame #0 {
                        n1091 = local read "Wellenplatte [°]"() -> (w1255:refnum<k7>)
                        n1092 = local read "L/2-Start [°]"() -> (w1249:dbl)
                        n1093 = invoke class="MG17Motor" method="SetAbsMovePos"(reference=w1255, "lChanID"=0, "fAbsPos"=w1249) -> (reference out=w1253:refnum<k7>, error out=w1250:errorcluster, "lChanID"=w1251:i32)  [unwired: 2 in, 2 out]
                        n1094 = local read "Aktuelle L/2-Position [°]"() -> (w1247:dbl)
                        n1095 = invoke class="MG17Motor" method="MoveAbsolute"(reference=w1253, error in=w1250, "lChanID"=w1251, "bWait"=TRUE) -> (reference out=w1246:refnum<k7>, "lChanID"=w1245:i32)  [unwired: 1 in, 3 out]
                        n1096 = invoke class="MG17Motor" method="GetPosition"(reference=w1246, "lChanID"=w1245, "pfPosition"=w1247) -> ("pfPosition"=w1248:sgl)  [unwired: 2 in, 4 out]
                        n1097 = local write "Aktuelle L/2-Position [°]"(w1248) -> ()
                      }
                      frame #1 {
                        n1098 = local write "Leistungs-/Polarisationscan läuft"(TRUE ("Messung läuft")) -> ()
                      }
                    }
                  }
                }
              }
            }
          }
          event #5 {
            n1099 = event-data() -> ("NewVal"=w1259:bool)  [unwired: 1 in]
            n1100 = local read "HV-Steuerung"() -> (w1257:bool)
            n1101 = local read "Kamera"() -> (w1260:bool)
            n1102 = Compound Arithmetic op=AND(w1260, w1259, w1257) -> (w1258:bool)
            n1103 = case shown="True" w1258 {
              frame #0 {
                n1104 = local write "Spannungsscan läuft"(FALSE ("Messung läuft")) -> ()
              }
              frame #1 {
                n1105 = stacked-sequence {
                  frame #0 {
                    n1106 = flat-sequence {
                      tunnel: [w1275] -> w1262
                      tunnel: w1262 -> [w1296]
                      frame #0 {
                        n1107 = Get Date/Time In Seconds() -> (seconds since 1Jan1904=w1263:timestamp)
                        n1108 = local write "Aktueller Messschritt"(0 ("Aktueller Messschritt")) -> ()
                        n1109 = local write "Start time [ms]"(w1263) -> ()
                        n1110 = local read "# Spannungsschritte"() -> (w1284:i32[])
                        n1111 = local read "Spannungsweite [V]"() -> (w1283:dbl[])
                        n1112 = control-ref of="Shutter time (ms)"() -> (w1288:refnum<vi>)
                        n1113 = property class="Ring (strikt)"(reference=w1288) -> ("RingText.Text"=w1287:string)  [unwired: 1 in, 2 out]
                        n1114 = local read "Suppressor-Spannung [V]"() -> (w1265:dbl)
                        n1115 = local read "# Bilder/Messschritt"() -> (w1281:i32)
                        n1116 = local read "Spannungsstart [V]"() -> (w1269:dbl[])
                        n1117 = local read "Tip-Spannung [V]"() -> (w1266:dbl)
                        n1118 = Divide(x=w1283, y=w1284) -> (x/y=w1285:dbl[])
                        n1119 = Decimal String To Number(string=w1287) -> (number=w1270:i32)  [unwired: 2 in, 1 out]
                        n1120 = local read "P-Schirm-Spannung [V]"() -> (w1273:dbl)
                        n1121 = local read "MCP-Spannung [V]"() -> (w1272:dbl)
                        n1122 = local read "Leistung (iK) [mW]"() -> (w1271:dbl)
                        n1123 = local read "Polarisation [°]"() -> (w1278:dbl)
                        n1124 = local read "Messlogbuch"() -> (w1280:path)
                        n1125 = local read "Proben-ID"() -> (w1279:string)
                        n1126 = Multiply(x=w1281, y=w1270) -> (x*y=w1282:i32)
                        n1127 = local write "Spannungsschritt [V]"(w1285) -> ()
                        n1128 = Replace Array Subset(array=w1269, new element #1=w1266, index #1=0 ("Index"), new element #2=w1265, index #2=1 ("Index")) -> (w1264:dbl[])
                        n1129 = local read "ROI"() -> (w1276:i32[])
                        n1130 = local write "Spannungsstart [V]"(w1264) -> ()
                        n1131 = local write "Aktuelle Spannung [V]"(w1264) -> ()
                        n1132 = call "stage_get_current_xyz.vi"() -> ("Aktuelle xyz-Position OUT [mm]"=w1274:dbl[])  [unwired: 3 in, 1 out]
                        n1133 = call "create_measure_log_entry.vi"("Messlogbuch-Pfad"=w1280, "Probe"=w1279, "Polarisation [°]"=w1278, "Messart"="Spannungsscan", "ROI"=w1276, "Messungen/Messschritt"=w1281, "Maximalleistung (iK) [mW]"=w1271, "Tip-Spannung [V]"=w1266, "Suppressor-Spannung [V]"=w1265, "Zeit/Messschritt [ms]"=w1270, "MCP-Spannung [V]"=w1272, "Zeit/Messung [ms]"=w1282, "Phosphorschirm-Spannung [V]"=w1273, "xyz [mm]"=w1274) -> ("Messung Nr."=w1275:i32)  [unwired: 4 in, 1 out]
                      }
                      frame #1 {
                        n1134 = local read "Fehler (Ausgang)"() -> (w1297:errorcluster)
                        n1135 = local read "Day folder"() -> (w1302:string)
                        n1136 = local read "Einzelbilder speichern"() -> (w1304:bool)
                        n1137 = local read "# Spannungsschritte"() -> (w1311:i32[])
                        n1138 = local read "Summierte Helligkeit speichern"() -> (w1292:bool)
                        n1139 = call "create_save_folder.vi"("Day folder"=w1302, "Measuring number"=w1296, "Measuring folder"="Spannungsscan" ("Subfolder"), "error in"=w1297) -> ("Save Folder"=w1301:string, "Error Out"=w1300:errorcluster)  [unwired: 5 in]
                        n1140 = local read "Gemittelte Bilder speichern"() -> (w1290:bool)
                        n1141 = local read "LAPD-Daten speichern"() -> (w1289:bool)
                        n1142 = local read "Einzelbilder speichern"() -> (w1291:bool)
                        n1143 = local write "Save folder"(w1301) -> ()
                        n1144 = case shown="True" w1304 {
                          tunnel: w1300 -> [w1312 w1314]
                          tunnel: [w1312 w1313] -> w1299
                          frame #0 {
                          }
                          frame #1 {
                            n1145 = local read "Save folder"() -> (w1317:string)
                            n1146 = Concatenate Strings(w1317, "\\Einzelbilder" ("Subfolder")) -> (w1315:string)
                            n1147 = String To Path(string=w1315) -> (path=w1318:path)
                            n1148 = call <vilib>:"Check if File or Folder Exists.vi"("error in (no error)"=w1314, "path"=w1318) -> ("error out"=w1313:errorcluster, "file or folder exists?"=w1319:bool, "dup path"=w1320:path)  [unwired: 7 in]
                            n1149 = case shown="False" w1319 {
                              tunnel: w1320 -> [w1321 _]
                              frame #0 {
                                n1150 = Create Folder(path (use dialog)=w1321) -> ()  [unwired: 2 in, 3 out]
                              }
                              frame #1 {
                              }
                            }
                          }
                        }
                        n1151 = Index Array(array=w1311, index #1=0 ("Index"), index #2=1 ("Index")) -> (element #1=w1308:i32, element #2=w1307:i32)
                        n1152 = Multiply(x=w1308, y=w1307) -> (x*y=w1294:i32)
                        n1153 = Compound Arithmetic op=OR(w1290, w1291, w1292, w1289) -> (w1293:bool)
                        n1154 = local write "Daten speichern"(w1293) -> ()
                        n1155 = local write "# Messschritte"(w1294) -> ()
                        n1156 = local read "Gemittelte Bilder speichern"() -> (w1305:bool)
                        n1157 = case shown="True" w1305 {
                          tunnel: w1299 -> [w1322 w1324]
                          tunnel: [w1322 w1323] -> w1298
                          frame #0 {
                          }
                          frame #1 {
                            n1158 = local read "Save folder"() -> (w1328:string)
                            n1159 = Concatenate Strings(w1328, "\\Gemittelte Bilder" ("Subfolder")) -> (w1330:string)
                            n1160 = String To Path(string=w1330) -> (path=w1327:path)
                            n1161 = call <vilib>:"Check if File or Folder Exists.vi"("error in (no error)"=w1324, "path"=w1327) -> ("error out"=w1323:errorcluster, "file or folder exists?"=w1326:bool, "dup path"=w1325:path)  [unwired: 7 in]
                            n1162 = case shown="False" w1326 {
                              tunnel: w1325 -> [w1331 _]
                              frame #0 {
                                n1163 = Create Folder(path (use dialog)=w1331) -> ()  [unwired: 2 in, 3 out]
                              }
                              frame #1 {
                              }
                            }
                          }
                        }
                        n1164 = local read "Kamera"() -> (w1306:bool)
                        n1165 = case shown="True" w1306 {
                          tunnel: [w1332 w1334] -> w1295
                          tunnel: w1298 -> [w1332 w1333]
                          frame #0 {
                          }
                          frame #1 {
                            n1166 = local read "Ereignis: FrameDone?"() -> (w1335:refnum<event-registration>)
                            n1167 = local read "Detektionskamera"() -> (w1336:T5)
                            n1168 = call "camera_release_configuration.vi"("error in"=w1333, "Session In"=w1336, "Ereignisregistrierung (Referenz) 2"=w1335) -> ("error out"=w1334:errorcluster)  [unwired: 1 out]
                          }
                        }
                        n1169 = local write "Fehler (Ausgang)"(w1295) -> ()
                      }
                    }
                  }
                  frame #1 {
                    n1170 = flat-sequence {
                      frame #0 {
                        w1342 = 1 ("Index")
                        w1343 = 0 ("Index")
                        n1171 = local read "# Spannungsschritte"() -> (w1353:i32[])
                        n1172 = local read "Spannungsstart [V]"() -> (w1338:dbl[])
                        n1173 = local read "Spannungsschritt [V]"() -> (w1341:dbl[])
                        n1174 = Index Array(array=w1353, index #1=w1343, index #2=w1342) -> (element #1=w1351:i32, element #2=w1352:i32)
                        n1175 = Index Array(array=w1338, index #1=w1343, index #2=w1342) -> (element #1=w1340:dbl, element #2=w1339:dbl)
                        n1176 = control-ref of="2D-Intensitätsverteilung (MCP)"() -> (w1337:refnum<vi>)
                        n1177 = Index Array(array=w1341, index #1=w1343, index #2=w1342) -> (element #1=w1345:dbl, element #2=w1344:dbl)
                        n1178 = Initialize Array(0.0 ("y"), w1351, w1352) -> (w1349:dbl[][])
                        n1179 = local write "2D-Intensitätsverteilung (MCP)"(w1349) -> ()
                        n1180 = property class="IntGraph (strikt)"(reference=w1337, "XScale.Offset"=w1340, "XScale.Multiplier"=w1345, "YScale.Offset"=w1339, "YScale.Multiplier"=w1344, "XScale.MinorInc"=w1345, "YScale.MinorInc"=w1344, "XScale.NameLbl.Text"="Tip-Spannung [V]" ("Y-Achse.Namensbeschriftung.Text"), "YScale.NameLbl.Text"="Suppressor-Spannung [V]" ("X-Achse.Namensbeschriftung.Text")) -> (error out=w1348:errorcluster)  [unwired: 1 in, 1 out]
                        n1181 = local write "Fehler (Ausgang)"(w1348) -> ()
                      }
                      frame #1 {
                        n1182 = local write "Spannungsscan läuft"(TRUE ("Messung läuft")) -> ()
                      }
                    }
                  }
                }
              }
            }
          }
          event #6 {
            n1183 = event-data() -> ("NewVal"=w1357:bool)  [unwired: 1 in]
            n1184 = local read "HV-Steuerung"() -> (w1355:bool)
            n1185 = local read "Kamera"() -> (w1358:bool)
            n1186 = Compound Arithmetic op=AND(w1358, w1357, w1355) -> (w1356:bool)
            n1187 = case shown="True" w1356 {
              frame #0 {
                n1188 = local write "x-U-Scan läuft"(FALSE ("Messung läuft")) -> ()
              }
              frame #1 {
                n1189 = stacked-sequence {
                  frame #0 {
                    # "Falls der gewählte Startwert für den Scan und der Startwert zur Berechnung der Ausgleichslage nicht identisch sind muss ein korrigierter Wert für die Raum-Koordinate 2 angefahren werden"
                    n1190 = local read "x-U-Scan (Ausgleichslage) Steigung"() -> (w1361:dbl)
                    n1191 = Not Equal?(x=w1361, y=0.0) -> (x != y?=w1362:bool)
                    n1192 = case shown="True" w1362 {
                      frame #0 {
                      }
                      frame #1 {
                        n1193 = flat-sequence {
                          tunnel: [w1365] -> w1363
                          tunnel: w1363 -> [w1378]
                          frame #0 {
                            n1194 = local read "x-U-Scan (Ausgleichslage) xy-Start [mm]"() -> (w1376:dbl[])
                            n1195 = local read "Raum-Koordinate 2 (Lagenausgleich)"() -> (w1365:enum16{"x-Achse", "y-Achse", "z-Achse"})
                            n1196 = local read "Raum-Koordinate 1"() -> (w1374:enum16{"x-Achse", "y-Achse", "z-Achse"})
                            n1197 = call "stage_get_current_xyz.vi"() -> ("Aktuelle xyz-Position OUT [mm]"=w1367:dbl[])  [unwired: 3 in, 1 out]
                            n1198 = local read "x-U-Scan (Ausgleichslage) Steigung"() -> (w1371:dbl)
                            n1199 = Index Array(array=w1367, index=w1374) -> (element=w1373:dbl)
                            n1200 = Index Array(array=w1376, index #1=w1374, index #2=w1365) -> (element #1=w1375:dbl, element #2=w1368:dbl)
                            n1201 = Subtract(x=w1373, y=w1375) -> (x-y=w1372:dbl)
                            n1202 = local write "x-U-Scan x-Startposition [mm]"(w1373) -> ()
                            n1203 = Multiply(x=w1372, y=w1371) -> (x*y=w1369:dbl)
                            n1204 = Increment(x=w1365) -> (x+1=w1370:enum16{"x-Achse", "y-Achse", "z-Achse"})
                            n1205 = Add(x=w1369, y=w1368) -> (x+y=w1364:dbl)
                            n1206 = Replace Array Subset(array=w1367, new element=w1364, index=w1365) -> (w1366:dbl[])
                            n1207 = call "stage_move_axis_absolute.vi"("Ziel xyz IN [mm]"=w1366, "Achse"=w1370) -> ()  [unwired: 1 in, 3 out]
                          }
                          frame #1 {
                            n1208 = call "stage_get_current_xyz.vi"() -> ("Aktuelle xyz-Position OUT [mm]"=w1379:dbl[])  [unwired: 3 in, 1 out]
                            n1209 = local write "Start xyz-Position [mm]"(w1379) -> ()
                            n1210 = Index Array(array=w1379, index=w1378) -> (element=w1377:dbl)
                            n1211 = local write "x-U-Scan y-Startposition [mm]"(w1377) -> ()
                          }
                        }
                      }
                    }
                  }
                  frame #1 {
                    n1212 = flat-sequence {
                      tunnel: [w1395] -> w1380
                      tunnel: w1380 -> [w1426]
                      frame #0 {
                        n1213 = Get Date/Time In Seconds() -> (seconds since 1Jan1904=w1386:timestamp)
                        n1214 = local write "Aktueller Messschritt"(0 ("Aktueller Messschritt")) -> ()
                        n1215 = local write "Start time [ms]"(w1386) -> ()
                        n1216 = local read "Spannungs-Koordinate"() -> (w1405:enum16{"Tip-Spannung", "Suppressor-Spannung"})
                        n1217 = local read "# x-U-Scan Spannungsschritte"() -> (w1410:i32)
                        n1218 = local read "x-U-Scan x-Rasterweite [µm]"() -> (w1408:dbl)
                        n1219 = local read "x-U-Scan Spannungsweite [V]"() -> (w1409:dbl)
                        n1220 = local read "# x-U-Scan x-Rasterschritte"() -> (w1407:i32)
                        n1221 = control-ref of="Shutter time (ms)"() -> (w1414:refnum<vi>)
                        n1222 = case shown="\"Suppressor-Spannung\", Voreinstellung" w1405 {
                          tunnel: [refnum<k21> "Dev0/Ao1" ("Spannungskanal") refnum<k21> "Dev0/Ao0" ("Spannungskanal")] -> w1404
                          tunnel: [w1415 w1417] -> w1387
                          frame #0 {
                            n1223 = local read "Tip-Spannung [V]"() -> (w1415:dbl)
                          }
                          frame #1 {
                            n1224 = local read "Suppressor-Spannung [V]"() -> (w1417:dbl)
                          }
                        }
                        n1225 = property class="Ring (strikt)"(reference=w1414) -> ("RingText.Text"=w1413:string)  [unwired: 1 in, 2 out]
                        n1226 = Divide(x=w1409, y=w1410) -> (x/y=w1411:dbl)
                        n1227 = Divide(x=w1408, y=w1407) -> (x/y=w1406:dbl)
                        n1228 = local read "# Bilder/Messschritt"() -> (w1396:i32)
                        n1229 = local write "x-U-Scan Spannungsschritt [V]"(w1411) -> ()
                        n1230 = local write "x-U-Scan x-Rasterschritt [µm]"(w1406) -> ()
                        n1231 = Decimal String To Number(string=w1413) -> (number=w1397:i32)  [unwired: 2 in, 1 out]
                        n1232 = local read "Suppressor-Spannung [V]"() -> (w1391:dbl)
                        n1233 = local read "P-Schirm-Spannung [V]"() -> (w1394:dbl)
                        n1234 = local read "MCP-Spannung [V]"() -> (w1393:dbl)
                        n1235 = local read "Leistung (iK) [mW]"() -> (w1392:dbl)
                        n1236 = local read "Tip-Spannung [V]"() -> (w1390:dbl)
                        n1237 = local read "Polarisation [°]"() -> (w1401:dbl)
                        n1238 = local read "Messlogbuch"() -> (w1403:path)
                        n1239 = local read "Proben-ID"() -> (w1402:string)
                        n1240 = Multiply(x=w1396, y=w1397) -> (x*y=w1398:i32)
                        n1241 = local read "ROI"() -> (w1399:i32[])
                        n1242 = local read "Raum-Koordinate 2 (Lagenausgleich)"() -> (w1383:enum16{"x-Achse", "y-Achse", "z-Achse"})
                        n1243 = local read "Raum-Koordinate 1"() -> (w1384:enum16{"x-Achse", "y-Achse", "z-Achse"})
                        n1244 = call "stage_get_current_xyz.vi"() -> ("Aktuelle xyz-Position OUT [mm]"=w1385:dbl[])  [unwired: 3 in, 1 out]
                        n1245 = call "create_measure_log_entry.vi"("Messlogbuch-Pfad"=w1403, "Probe"=w1402, "Polarisation [°]"=w1401, "Messart"="x-U-Scan", "ROI"=w1399, "Messungen/Messschritt"=w1396, "Maximalleistung (iK) [mW]"=w1392, "Tip-Spannung [V]"=w1390, "Suppressor-Spannung [V]"=w1391, "Zeit/Messschritt [ms]"=w1397, "MCP-Spannung [V]"=w1393, "Zeit/Messung [ms]"=w1398, "Phosphorschirm-Spannung [V]"=w1394, "xyz [mm]"=w1385) -> ("Messung Nr."=w1395:i32)  [unwired: 4 in, 1 out]
                        n1246 = local write "Start xyz-Position [mm]"(w1385) -> ()
                        n1247 = Index Array(array=w1385, index #1=w1384, index #2=w1383) -> (element #1=w1381:dbl, element #2=w1382:dbl)
                        n1248 = Add(x=w1384, y=1) -> (x+y=w1388:i32)
                        n1249 = local write "Spannungskanal"(w1404) -> ()
                        n1250 = local write "x-U-Scan Spannungsstart [V]"(w1387) -> ()
                        n1251 = local write "x-U-Scan aktuelle Spannung [V]"(w1387) -> ()
                        n1252 = local write "x-U-Scan x-Startposition [mm]"(w1381) -> ()
                        n1253 = local write "x-U-Scan aktuelle x-Position [mm]"(w1381) -> ()
                        n1254 = local write "x-U-Scan aktuelle y-Position [mm]"(w1382) -> ()
                        n1255 = local write "x-U-Scan y-Startposition [mm]"(w1382) -> ()
                        n1256 = local write "Achs-ID"(w1388) -> ()
                      }
                      frame #1 {
                        n1257 = local read "Fehler (Ausgang)"() -> (w1429:errorcluster)
                        n1258 = local read "Day folder"() -> (w1434:string)
                        n1259 = local read "Summierte Helligkeit speichern"() -> (w1422:bool)
                        n1260 = local read "# x-U-Scan Spannungsschritte"() -> (w1425:i32)
                        n1261 = local read "# x-U-Scan x-Rasterschritte"() -> (w1424:i32)
                        n1262 = local read "Gemittelte Bilder speichern"() -> (w1420:bool)
                        n1263 = local read "LAPD-Daten speichern"() -> (w1419:bool)
                        n1264 = local read "Einzelbilder speichern"() -> (w1421:bool)
                        n1265 = local read "Einzelbilder speichern"() -> (w1436:bool)
                        n1266 = call "create_save_folder.vi"("Day folder"=w1434, "Measuring number"=w1426, "Measuring folder"="x-U-Scan" ("Subfolder"), "error in"=w1429) -> ("Save Folder"=w1433:string, "Error Out"=w1432:errorcluster)  [unwired: 5 in]
                        n1267 = Multiply(x=w1425, y=w1424) -> (x*y=w1427:i32)
                        n1268 = local write "Save folder"(w1433) -> ()
                        n1269 = case shown="True" w1436 {
                          tunnel: w1432 -> [w1439 w1441]
                          tunnel: [w1439 w1440] -> w1431
                          frame #0 {
                          }
                          frame #1 {
                            n1270 = local read "Save folder"() -> (w1444:string)
                            n1271 = Concatenate Strings(w1444, "\\Einzelbilder" ("Subfolder")) -> (w1442:string)
                            n1272 = String To Path(string=w1442) -> (path=w1445:path)
                            n1273 = call <vilib>:"Check if File or Folder Exists.vi"("error in (no error)"=w1441, "path"=w1445) -> ("error out"=w1440:errorcluster, "file or folder exists?"=w1446:bool, "dup path"=w1447:path)  [unwired: 7 in]
                            n1274 = case shown="False" w1446 {
                              tunnel: w1447 -> [w1448 _]
                              frame #0 {
                                n1275 = Create Folder(path (use dialog)=w1448) -> ()  [unwired: 2 in, 3 out]
                              }
                              frame #1 {
                              }
                            }
                          }
                        }
                        n1276 = Compound Arithmetic op=OR(w1420, w1421, w1422, w1419) -> (w1423:bool)
                        n1277 = local write "Daten speichern"(w1423) -> ()
                        n1278 = local write "# Messschritte"(w1427) -> ()
                        n1279 = local read "Gemittelte Bilder speichern"() -> (w1437:bool)
                        n1280 = case shown="True" w1437 {
                          tunnel: w1431 -> [w1449 w1451]
                          tunnel: [w1449 w1450] -> w1430
                          frame #0 {
                          }
                          frame #1 {
                            n1281 = local read "Save folder"() -> (w1455:string)
                            n1282 = Concatenate Strings(w1455, "\\Gemittelte Bilder" ("Subfolder")) -> (w1457:string)
                            n1283 = String To Path(string=w1457) -> (path=w1454:path)
                            n1284 = call <vilib>:"Check if File or Folder Exists.vi"("error in (no error)"=w1451, "path"=w1454) -> ("error out"=w1450:errorcluster, "file or folder exists?"=w1453:bool, "dup path"=w1452:path)  [unwired: 7 in]
                            n1285 = case shown="False" w1453 {
                              tunnel: w1452 -> [w1458 _]
                              frame #0 {
                                n1286 = Create Folder(path (use dialog)=w1458) -> ()  [unwired: 2 in, 3 out]
                              }
                              frame #1 {
                              }
                            }
                          }
                        }
                        n1287 = local read "Kamera"() -> (w1438:bool)
                        n1288 = case shown="True" w1438 {
                          tunnel: [w1459 w1461] -> w1428
                          tunnel: w1430 -> [w1459 w1460]
                          frame #0 {
                          }
                          frame #1 {
                            n1289 = local read "Ereignis: FrameDone?"() -> (w1462:refnum<event-registration>)
                            n1290 = local read "Detektionskamera"() -> (w1463:T5)
                            n1291 = call "camera_release_configuration.vi"("error in"=w1460, "Session In"=w1463, "Ereignisregistrierung (Referenz) 2"=w1462) -> ("error out"=w1461:errorcluster)  [unwired: 1 out]
                          }
                        }
                        n1292 = local write "Fehler (Ausgang)"(w1428) -> ()
                      }
                    }
                  }
                  frame #2 {
                    n1293 = flat-sequence {
                      frame #0 {
                        n1294 = local read "# x-U-Scan Spannungsschritte"() -> (w1472:i32)
                        n1295 = local read "x-U-Scan x-Rasterschritt [µm]"() -> (w1465:dbl)
                        n1296 = local read "# x-U-Scan x-Rasterschritte"() -> (w1471:i32)
                        n1297 = Initialize Array(0.0 ("y"), w1471, w1472) -> (w1476:dbl[][])
                        n1298 = Divide(x=w1465, y=1000.0) -> (x/y=w1466:dbl)
                        n1299 = local write "2D-Intensitätsverteilung (MCP)"(w1476) -> ()
                        n1300 = local read "x-U-Scan Spannungsschritt [V]"() -> (w1468:dbl)
                        n1301 = local read "x-U-Scan x-Startposition [mm]"() -> (w1469:dbl)
                        n1302 = local read "x-U-Scan Spannungsstart [V]"() -> (w1470:dbl)
                        n1303 = control-ref of="2D-Intensitätsverteilung (MCP)"() -> (w1467:refnum<vi>)
                        n1304 = property class="IntGraph (strikt)"(reference=w1467, "XScale.Offset"=w1469, "XScale.Multiplier"=w1466, "YScale.Offset"=w1470, "YScale.Multiplier"=w1468, "XScale.MinorInc"=w1466, "YScale.MinorInc"=w1468, "XScale.NameLbl.Text"="Position [mm]" ("Y-Achse.Namensbeschriftung.Text"), "YScale.NameLbl.Text"="Spannung [V]" ("X-Achse.Namensbeschriftung.Text")) -> (error out=w1475:errorcluster)  [unwired: 1 in, 1 out]
                        n1305 = local write "Fehler (Ausgang)"(w1475) -> ()
                      }
                      frame #1 {
                        n1306 = local write "x-U-Scan läuft"(TRUE ("Messung läuft")) -> ()
                      }
                    }
                  }
                }
              }
            }
          }
          event #7 {
            n1307 = event-data() -> ("NewVal"=w1479:bool)  [unwired: 1 in]
            n1308 = case shown="True" w1479 {
              frame #0 {
              }
              frame #1 {
                n1309 = flat-sequence {
                  tunnel: [w1484] -> w1480
                  tunnel: w1480 -> [w1501]
                  frame #0 {
                    n1310 = local write "Ausgleichslage Start festlegen"(FALSE ("Ausgleichslage Ende festlegen")) -> ()
                    n1311 = local read "Raum-Koordinate 2 (Lagenausgleich)"() -> (w1482:enum16{"x-Achse", "y-Achse", "z-Achse"})
                    n1312 = local read "Raum-Koordinate 1"() -> (w1483:enum16{"x-Achse", "y-Achse", "z-Achse"})
                    n1313 = local read "x-U-Scan (Ausgleichslage) xy-Start [mm]"() -> (w1485:dbl[])
                    n1314 = call "stage_get_current_xyz.vi"() -> ("Aktuelle xyz-Position OUT [mm]"=w1490:dbl[])  [unwired: 3 in, 1 out]
                    n1315 = Index Array(array=w1490, index #1=w1483, index #2=w1482) -> (element #1=w1487:dbl, element #2=w1486:dbl)
                    n1316 = Replace Array Subset(array=w1485, new element #1=w1487, index #1=0 ("Index"), new element #2=w1486, index #2=1 ("Index")) -> (w1484:dbl[])
                    n1317 = local write "x-U-Scan (Ausgleichslage) xy-Start [mm]"(w1484) -> ()
                  }
                  frame #1 {
                    n1318 = local read "x-U-Scan (Ausgleichslage) xy-End [mm]"() -> (w1502:dbl[])
                    n1319 = Index Array(array=w1501, index #1=0 ("Index"), index #2=1 ("Index")) -> (element #1=w1493:dbl, element #2=w1496:dbl)
                    n1320 = Index Array(array=w1502, index #1=0 ("Index"), index #2=1 ("Index")) -> (element #1=w1492:dbl, element #2=w1495:dbl)
                    n1321 = Not Equal?(x=w1493, y=w1492) -> (x != y?=w1491:bool)
                    n1322 = case shown="True" w1491 {
                      tunnel: w1496 -> [_ w1508]
                      tunnel: w1495 -> [_ w1507]
                      tunnel: w1492 -> [_ w1506]
                      tunnel: w1493 -> [_ w1505]
                      tunnel: [0.0 w1504] -> w1494
                      frame #0 {
                      }
                      frame #1 {
                        n1323 = Subtract(x=w1508, y=w1507) -> (x-y=w1510:dbl)
                        n1324 = Subtract(x=w1505, y=w1506) -> (x-y=w1509:dbl)
                        n1325 = Divide(x=w1510, y=w1509) -> (x/y=w1504:dbl)
                      }
                    }
                    n1326 = local write "x-U-Scan (Ausgleichslage) Steigung"(w1494) -> ()
                  }
                }
              }
            }
          }
          event #8 {
            n1327 = event-data() -> ("NewVal"=w1511:bool)  [unwired: 1 in]
            n1328 = case shown="True" w1511 {
              frame #0 {
              }
              frame #1 {
                n1329 = flat-sequence {
                  tunnel: [w1516] -> w1512
                  tunnel: w1512 -> [w1533]
                  frame #0 {
                    n1330 = local write "Ausgleichslage Ende festlegen"(FALSE ("Ausgleichslage Ende festlegen")) -> ()
                    n1331 = local read "Raum-Koordinate 2 (Lagenausgleich)"() -> (w1514:enum16{"x-Achse", "y-Achse", "z-Achse"})
                    n1332 = local read "Raum-Koordinate 1"() -> (w1515:enum16{"x-Achse", "y-Achse", "z-Achse"})
                    n1333 = local read "x-U-Scan (Ausgleichslage) xy-End [mm]"() -> (w1517:dbl[])
                    n1334 = call "stage_get_current_xyz.vi"() -> ("Aktuelle xyz-Position OUT [mm]"=w1522:dbl[])  [unwired: 3 in, 1 out]
                    n1335 = Index Array(array=w1522, index #1=w1515, index #2=w1514) -> (element #1=w1519:dbl, element #2=w1518:dbl)
                    n1336 = Replace Array Subset(array=w1517, new element #1=w1519, index #1=0 ("Index"), new element #2=w1518, index #2=1 ("Index")) -> (w1516:dbl[])
                    n1337 = local write "x-U-Scan (Ausgleichslage) xy-End [mm]"(w1516) -> ()
                  }
                  frame #1 {
                    n1338 = local read "x-U-Scan (Ausgleichslage) xy-Start [mm]"() -> (w1534:dbl[])
                    n1339 = Index Array(array=w1533, index #1=0 ("Index"), index #2=1 ("Index")) -> (element #1=w1525:dbl, element #2=w1528:dbl)
                    n1340 = Index Array(array=w1534, index #1=0 ("Index"), index #2=1 ("Index")) -> (element #1=w1524:dbl, element #2=w1527:dbl)
                    n1341 = Not Equal?(x=w1525, y=w1524) -> (x != y?=w1523:bool)
                    n1342 = case shown="True" w1523 {
                      tunnel: w1528 -> [_ w1540]
                      tunnel: w1527 -> [_ w1539]
                      tunnel: w1524 -> [_ w1538]
                      tunnel: w1525 -> [_ w1537]
                      tunnel: [0.0 w1536] -> w1526
                      frame #0 {
                      }
                      frame #1 {
                        n1343 = Subtract(x=w1540, y=w1539) -> (x-y=w1542:dbl)
                        n1344 = Subtract(x=w1537, y=w1538) -> (x-y=w1541:dbl)
                        n1345 = Divide(x=w1542, y=w1541) -> (x/y=w1536:dbl)
                      }
                    }
                    n1346 = local write "x-U-Scan (Ausgleichslage) Steigung"(w1526) -> ()
                  }
                }
              }
            }
          }
          event #9 {
            n1347 = event-data() -> ("NewVal"=w1543:bool)  [unwired: 1 in]
            n1348 = case shown="True" w1543 {
              frame #0 {
              }
              frame #1 {
                n1349 = control-ref of="Shutter time (ms)"() -> (w1579:refnum<vi>)
                n1350 = property class="Ring (strikt)"(reference=w1579) -> ("RingText.Text"=w1561:string)  [unwired: 1 in, 2 out]
                n1351 = local read "# Bilder/Messschritt"() -> (w1557:i32)
                n1352 = local read "Suppressor-Spannung [V]"() -> (w1544:dbl)
                n1353 = local read "P-Schirm-Spannung [V]"() -> (w1549:dbl)
                n1354 = local read "MCP-Spannung [V]"() -> (w1548:dbl)
                n1355 = Decimal String To Number(string=w1561) -> (number=w1556:i32)  [unwired: 2 in, 1 out]
                n1356 = local read "Leistung (iK) [mW]"() -> (w1547:dbl)
                n1357 = local read "Tip-Spannung [V]"() -> (w1545:dbl)
                n1358 = local read "Polarisation [°]"() -> (w1552:dbl)
                n1359 = local read "Messlogbuch"() -> (w1554:path)
                n1360 = local read "Proben-ID"() -> (w1553:string)
                n1361 = Concatenate Strings(w1561, "ms_" ("String")) -> (w1560:string)
                n1362 = Multiply(x=w1557, y=w1556) -> (x*y=w1555:i32)
                n1363 = local read "Sequenz Ordner"() -> (w1577:string)
                n1364 = local read "ROI"() -> (w1550:i32[])
                n1365 = local read "Day folder"() -> (w1578:string)
                n1366 = call "stage_get_current_xyz.vi"() -> ("Aktuelle xyz-Position OUT [mm]"=w1558:dbl[])  [unwired: 3 in, 1 out]
                n1367 = call "create_measure_log_entry.vi"("Messlogbuch-Pfad"=w1554, "Probe"=w1553, "Polarisation [°]"=w1552, "Messart"="Referenzbilder", "ROI"=w1550, "Messungen/Messschritt"=w1557, "Maximalleistung (iK) [mW]"=w1547, "Tip-Spannung [V]"=w1545, "Suppressor-Spannung [V]"=w1544, "Zeit/Messschritt [ms]"=w1556, "MCP-Spannung [V]"=w1548, "Zeit/Messung [ms]"=w1555, "Phosphorschirm-Spannung [V]"=w1549, "xyz [mm]"=w1558) -> ("Messung Nr."=w1546:i32)  [unwired: 4 in, 1 out]
                n1368 = call "create_save_folder.vi"("Day folder"=w1578, "Measuring number"=w1546, "Measuring folder"=w1577) -> ("Save Folder"=w1564:string, "Error Out"=w1575:errorcluster)  [unwired: 6 in]
                n1369 = local write "Save folder"(w1564) -> ()
                n1370 = local read "Kamera"() -> (w1576:bool)
                n1371 = case shown="True" w1576 {
                  tunnel: [w1581 w1584] -> w1567
                  tunnel: w1575 -> [w1581 w1583]
                  tunnel: [w1580 w1582] -> w1566
                  frame #0 {
                    n1372 = local read "Detektionskamera"() -> (w1580:T5)
                  }
                  frame #1 {
                    n1373 = local read "Ereignis: FrameDone?"() -> (w1585:refnum<event-registration>)
                    n1374 = local read "Detektionskamera"() -> (w1586:T5)
                    n1375 = call "camera_release_configuration.vi"("error in"=w1583, "Session In"=w1586, "Ereignisregistrierung (Referenz) 2"=w1585) -> ("error out"=w1584:errorcluster, "Session Out"=w1582:T5)
                  }
                }
                n1376 = local read "# Bilder/Messschritt"() -> (w1573:i32)
                n1377 = call "camera_acquisition_sequence.vi"("Session In"=w1566, "Desired image number"=w1573, "error in"=w1567) -> ("Session Out"=w1565:T5, "Image Array"=w1574:T4[], "error out"=w1572:errorcluster)  [unwired: 1 in]
                n1378 = local read "Buffer Interval"() -> (w1570:u32)
                n1379 = call "save images.vi"("Save Folder"=w1564, "File name prefix"=w1560, "Array"=w1574, "error out 2"=w1572, "Bilder/Messschritt"=w1573) -> ("error out"=w1569:errorcluster)
                n1380 = call "camera_create_configuration.vi"("error in"=w1569, "BufferInterval"=w1570, "Session Out 2"=w1565) -> ("Fehler (Ausgang)"=w1563:errorcluster, "Session Out"=w1568:T5, "Ereignisregistrierung (Referenz)"=w1571:refnum<event-registration>)
                n1381 = local write "Ereignis: FrameDone?"(w1571) -> ()
                n1382 = local write "Detektionskamera"(w1568) -> ()
                n1383 = local write "Fehler (Ausgang)"(w1563) -> ()
                n1384 = Unbundle By Name(w1563) -> ("status"=w1559:bool)
                n1385 = local write "Sequenzaufnahme ON"(w1559) -> ()
              }
            }
          }
        }
        n1386 = local read "Fehler (Ausgang)"() -> (w633:errorcluster)
        n1387 = local read "Programm beenden"() -> (w631:bool)
        n1388 = Unbundle By Name(w633) -> ("status"=w632:bool)
        n1389 = Or(x=w632, y=w631) -> (x .or. y?=w628:bool)
        "Scanschleifenzähler" <- w629
      }
    }
    frame #2 {
      n1390 = flat-sequence {
        frame #0 {
          n1391 = local read "Kamera"() -> (w1647:bool)
          n1392 = case shown="True" w1647 {
            frame #0 {
            }
            frame #1 {
              n1393 = local read "Detektionskamera"() -> (w1649:T5)
              n1394 = local read "Image Memory"() -> (w1651:T4)
              n1395 = call "camera_release configuration_stop.vi"("Image Memory"=w1651, "Detektionskamera"=w1649) -> ("error out"=w1648:errorcluster, "status"=w1650:bool)
              n1396 = local write "Kamera"(w1650) -> ()
              n1397 = local write "Fehler (Ausgang)"(w1648) -> ()
            }
          }
        }
        frame #1 {
          # "Wegen Abstürzen des Programms wird dieser Teil verhindert\nAchtung: IMMER manuell Netzteile auf 0V setzen oder HV-\nSteuerung von Hand ausmachen"
          n1398 = local read "HV-Steuerung"() -> (w1654:bool)
          n1399 = And(x=w1654, y=FALSE) -> (x .and. y?=w1652:bool)
          n1400 = case shown="True" w1652 {
            frame #0 {
            }
            frame #1 {
              n1401 = call "HV_power_supply_set_voltage.vi"("Desired output voltage in V (HV power supply)"=0.0, "Channel of HV power supply"=refnum<k21> "Dev0/Ao1") -> ("error out"=w1655:errorcluster)  [unwired: 8 in]
              n1402 = call "HV_power_supply_set_voltage.vi"("Desired output voltage in V (HV power supply)"=0.0, "Channel of HV power supply"=refnum<k21> "Dev0/Ao0") -> ("error out"=w1656:errorcluster)  [unwired: 8 in]
              n1403 = local write "Fehler (Ausgang)"(w1655) -> ()
              n1404 = local write "Fehler (Ausgang)"(w1656) -> ()
            }
          }
        }
        frame #2 {
          n1405 = local read "Wellenplatte"() -> (w1661:bool)
          n1406 = case shown="True" w1661 {
            frame #0 {
            }
            frame #1 {
              n1407 = local read "Wellenplatte [°]"() -> (w1662:refnum<k7>)
              n1408 = invoke class="MG17Motor" method="StopCtrl"(reference=w1662) -> ()  [unwired: 2 in, 3 out]
            }
          }
        }
        frame #3 {
          w1663 = FALSE ("Bühne bereit")
          w1664 = 0.0 ("Suppressor-Spannung [V]")
          n1409 = local write "Tip-Spannung [V]"(w1664) -> ()
          n1410 = local write "Suppressor-Spannung [V]"(w1664) -> ()
          n1411 = local write "Bühne"(w1663) -> ()
          n1412 = local write "Leistungs-/Polarisationsscan ON/OFF"(w1663) -> ()
          n1413 = local write "Wellenplatte"(w1663) -> ()
          n1414 = local write "Spannungsscan läuft"(w1663) -> ()
          n1415 = local write "HV-Steuerung"(w1663) -> ()
          n1416 = local write "x-U-Scan läuft"(w1663) -> ()
          n1417 = local write "Waveplate ON/OFF"(w1663) -> ()
          n1418 = local write "x-U-Scan ON/OFF"(w1663) -> ()
          n1419 = local write "Kamera ON/OFF"(w1663) -> ()
          n1420 = local write "Leistungs-/Polarisationscan läuft"(w1663) -> ()
        }
      }
    }
  }
